vi "KVP Parser.vi"(4 "Values":variant[](array[variant]), 6 "Keys":string[](array[string]), 8 "Strict type matching? (F)":bool, 9 "Default Value Name (empty: label)":string, 10 "Default Value":variant, 11 "Parent Name":string) -> (0 "all found?":bool, 1 "any found?":bool, 2 "Value":variant, 3 "name out":string)   [LabVIEW 2013]
doc: "This VI takes a default value as the input and replaces it recursively (cluster, array) with values found in key value pair arrays."
uses:
  TypeDescriptor/TypeDescriptor_GetPString.vi
  TypeDescriptor/TypeDescriptor_SetName.vi
  <vilib>/Utility/GetType.llb/TD_Create Cluster.vi
  TypeDescriptor/OpenDescriptor.lvlib
  Variant/OpenVariant.lvlib
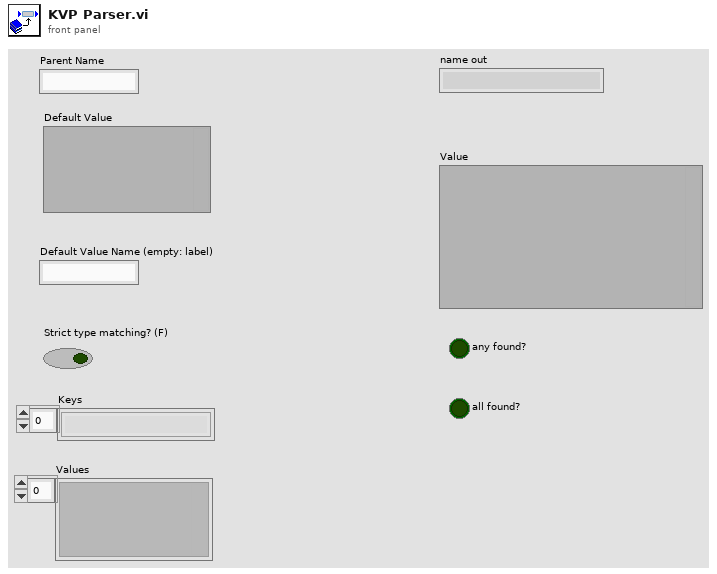
[diagram p1: front panel]
types:
  T1 = typedef "Type Enum.ctl" = enum8{"Void", "I8", "I16", "I32", "I64", "U8", "U16", "U32", "U64", "Single Float", "Double Float", "Extended Float", "Single Complex", "Double Complex", "Extended Complex", "Enum I8 NEVER", "Enum I16 NEVER", "Enum I32 NEVER", "Enum I64 NEVER", "Enum U8", "Enum U16", "Enum U32", "Enum U64", "Single Float With Unit", "Double Float With Unit", "Extended Float With Unit", "Single Complex With Unit", "Double Complex With Unit", "Extended Complex With Unit", "boolU16", "Boolean", "String", "Handle", "Path", "Picture", "C String", "Pascal String", "Tag", "SubString", "Array", "SubArray", "Cluster", "Numeric Cluster", "Variant", "LV Variant", "Measure Data (waveform)", "Refnum", "ExtData", "function", "Typedef", "Poly VI", "bad wire", "LabVIEW Class Instance"}
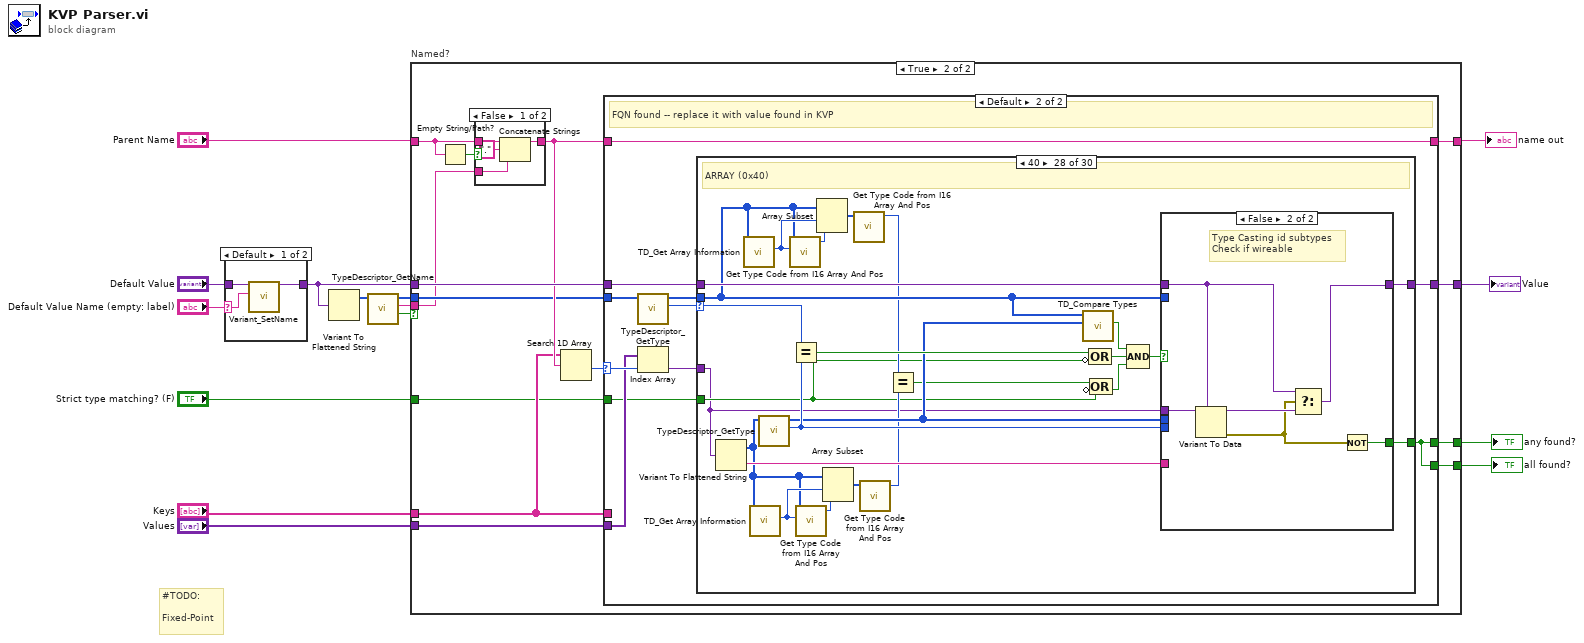
[diagram p0: block diagram]
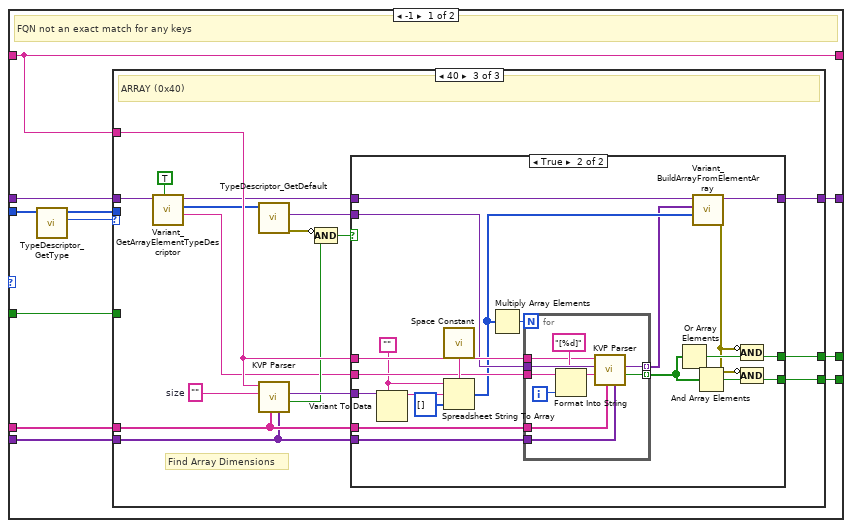
[diagram p5: hidden frame]
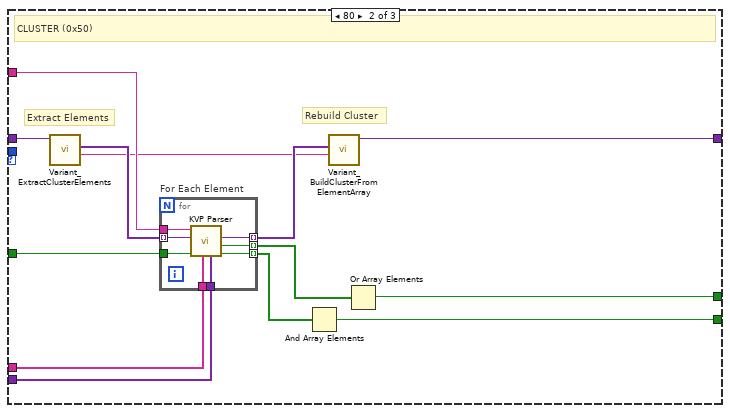
[diagram p7: hidden frame]
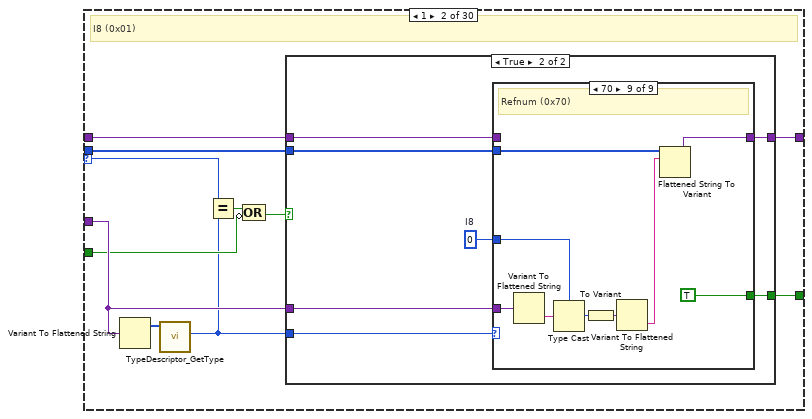
[diagram p10: hidden frame]
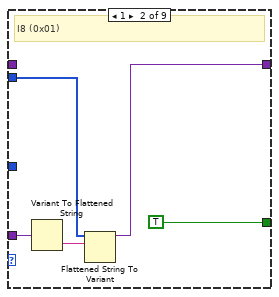
[diagram p13: hidden frame]
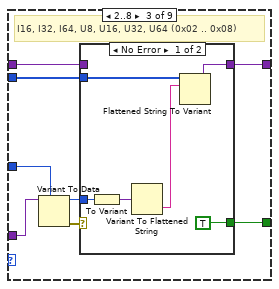
[diagram p14: hidden frame]
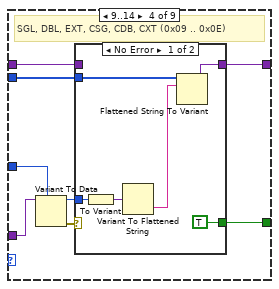
[diagram p16: hidden frame]
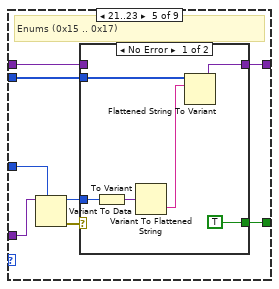
[diagram p18: hidden frame]
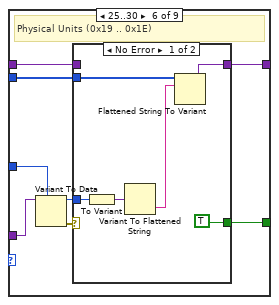
[diagram p20: hidden frame]
diagram:
  # "#TODO: \n\nFixed-Point"
  n1 = case shown="Default" "Default Value Name (empty: label)" {
    selector: "Default Value Name (empty: label)" -> [w17 _]
    tunnel: "Default Value" -> [w18 w19]
    tunnel: [w16 w19] -> w4
    frame Default {
      n2 = call "Variant_SetName.vi"("Name"=w17, "Variant"=w18) -> ("Named Variant"=w16:variant)  [unwired: 9 in]
    }
    frame "" {
    }
  }
  n3 = Variant To Flattened String(Variant=w4) -> (1:w3:i16[])  [unwired: 1 out]
  n4 = call "TypeDescriptor_GetName.vi"("type descriptor"=w3) -> ("found"=w1:bool, "name"=w2:string, "type descriptor dup"=w15:i16[])  [unwired: 8 in]
  n5 = case "Named?" shown="True" w1 {
    tunnel: [w21 w35] -> w13
    tunnel: w4 -> [w21 w34]
    tunnel: w15 -> [_ w26]
    tunnel: w2 -> [_ w22]
    tunnel: "Values" -> [_ w33]
    tunnel: "Keys" -> [_ w27]
    tunnel: "Parent Name" -> [w20 w29]
    tunnel: [w20 w32] -> w14
    tunnel: "Strict type matching? (F)" -> [_ w25]
    tunnel: [_ w24] -> w8
    tunnel: [_ w23] -> w7
    frame False {
      # "No Name Found -- no value to replace"
    }
    frame True {
      # "Has Name?"
      n6 = Empty String/Path?(string/path=w29) -> (empty?=w30:bool)
      n7 = case shown="False" w30 {
        tunnel: w22 -> [w37 w40]
        tunnel: [w38 w40] -> w28
        tunnel: w29 -> [w39 _]
        frame False {
          n8 = Concatenate Strings(w39, "." ("string"), w37) -> (w38:string)
        }
        frame True {
        }
      }
      n9 = Search 1D Array(1D array=w27, element=w28) -> (index of element=w31:i32)  [unwired: 1 in]
      n10 = case shown="Default" w31 {
        selector: w31 -> [_ w127]
        tunnel: [w50 w133] -> w35
        tunnel: w34 -> [w49 w132]
        tunnel: w26 -> [w51 w131]
        tunnel: w33 -> [w47 w126]
        tunnel: w28 -> [w45 w128]
        tunnel: [w45 w128] -> w32
        tunnel: w27 -> [w48 _]
        tunnel: w25 -> [w44 w124]
        tunnel: [w43 w123] -> w24
        tunnel: [w42 w123] -> w23
        frame -1 {
          # "FQN not an exact match for any keys"
          n11 = call "TypeDescriptor_GetType.vi"("type descriptor"=w51) -> ("Type"=w46:u8, "type descriptor dup"=w41:i16[])  [unwired: 9 in]
          n12 = case shown="40" w46 {
            tunnel: [w52 w54 w88] -> w50
            tunnel: w49 -> [w52 w63 w76]
            tunnel: w47 -> [_ w65 w86]
            tunnel: w48 -> [_ w64 w87]
            tunnel: w45 -> [_ w62 w83]
            tunnel: w44 -> [_ w61 _]
            tunnel: [_ w59 w90] -> w43
            tunnel: [_ w57 w89] -> w42
            tunnel: w41 -> [_ _ _]
            frame Default {
              # "No Match"
            }
            frame 80 {
              # "Rebuild Cluster"
              # "Extract Elements"
              # "CLUSTER (0x50)"
              n13 = call "Variant_ExtractClusterElements.vi"("Cluster"=w63) -> ("name"=w53:string, "Elements"=w55:variant[])  [unwired: 8 in, 1 out]
              n14 = for "For Each Element" {
                tunnel: [w73] -> w56 mode=indexing
                tunnel: w65 -> [w66]
                tunnel: w64 -> [w72]
                tunnel: w55 -> [w71] mode=indexing
                tunnel: w62 -> [w70]
                tunnel: [w69] -> w60 mode=indexing
                tunnel: [w68] -> w58 mode=indexing
                tunnel: w61 -> [w67]
                n15 = call "KVP Parser.vi"("Values"=w66, "Keys"=w72, "Strict type matching? (F)"=w67, "Default Value"=w71, "Parent Name"=w70) -> ("all found?"=w69:bool, "any found?"=w68:bool, "Value"=w73:variant)  [unwired: 3 in, 1 out]
              }
              n16 = And Array Elements(Boolean array=w60) -> (logical AND=w59:bool)
              n17 = call "Variant_BuildClusterFromElementArray.vi"("name"=w53, "Elements"=w56) -> ("Cluster"=w54:variant)  [unwired: 9 in]
              n18 = Or Array Elements(Boolean array=w58) -> (logical OR=w57:bool)
            }
            frame 64 {
              w84 = ""  # size
              # "Find Array Dimensions"
              # "ARRAY (0x40)"
              n19 = call "Variant_GetArrayElementTypeDescriptor.vi"("Name Element if empty string (F)"=TRUE, "Array"=w76) -> ("Element Name"=w78:string, "Element Descriptor"=w77:i16[], "Array dup"=w75:variant)  [unwired: 7 in]
              n20 = call "TypeDescriptor_GetDefault.vi"("type descriptor"=w77) -> ("error out"=w74:errorcluster, "Default"=w81:variant)  [unwired: 8 in, 1 out]
              n21 = call "KVP Parser.vi"("Values"=w86, "Keys"=w87, "Default Value"=w84, "Parent Name"=w83) -> ("any found?"=w80:bool, "Value"=w85:variant)  [unwired: 4 in, 2 out]
              n22 = Compound Arithmetic op=AND(invert w74, w80) -> (w79:bool)
              n23 = case shown="True" w79 {
                tunnel: [_ w95] -> w90
                tunnel: [_ w98] -> w89
                tunnel: [w91 w100] -> w88
                tunnel: w87 -> [_ w108]
                tunnel: w86 -> [_ w107]
                tunnel: w85 -> [_ w106]
                tunnel: w83 -> [_ w104]
                tunnel: w78 -> [_ w103]
                tunnel: w75 -> [w91 w101]
                tunnel: w81 -> [_ w94]
                frame False {
                  # "No Array Dimensions Found in the key value pairs"
                }
                frame True {
                  w102 = "" ("format string")
                  n24 = Variant To Data(type=w102, Variant=w106) -> (data=w105:string)  [unwired: 1 in, 1 out]
                  n25 = call <vilib>:"Space Constant.vi"() -> ("String"=w109:string)
                  n26 = Spreadsheet String To Array(delimiter (Tab)=w109, format string=w102, spreadsheet string=w105, array type (2D Dbl)=u32[] [] ("Dimensions")) -> (array=w93:u32[])
                  n27 = Multiply Array Elements(1:w93) -> (0:w112:u32)
                  n28 = for {
                    N: w112 -> [_]
                    tunnel: w94 -> [w122]
                    tunnel: w107 -> [w120]
                    tunnel: w108 -> [w118]
                    tunnel: w104 -> [w117]
                    tunnel: [w116] -> w111 mode=indexing
                    tunnel: w103 -> [w115]
                    tunnel: [w113] -> w92 mode=indexing
                    i -> [w114]
                    n29 = Format Into String(format string="[%d]", initial string=w115, w114) -> (resulting string=w119:string)  [unwired: 1 in, 1 out]
                    n30 = call "KVP Parser.vi"("Values"=w120, "Keys"=w118, "Default Value Name (empty: label)"=w119, "Default Value"=w122, "Parent Name"=w117) -> ("any found?"=w116:bool, "Value"=w113:variant)  [unwired: 3 in, 2 out]
                  }
                  n31 = Or Array Elements(Boolean array=w111) -> (logical OR=w99:bool)
                  n32 = call "Variant_BuildArrayFromElementArray.vi"("Dimensions"=w93, "Elements"=w92, "Default Array"=w101) -> ("error out"=w97:errorcluster, "Output Array"=w100:variant)  [unwired: 7 in]
                  n33 = And Array Elements(Boolean array=w111) -> (logical AND=w96:bool)
                  n34 = Compound Arithmetic op=AND(invert w97, w99) -> (w98:bool)
                  n35 = Compound Arithmetic op=AND(invert w97, w96) -> (w95:bool)
                }
              }
            }
          }
        }
        frame Default {
          # "FQN found -- replace it with value found in KVP"
          n36 = call "TypeDescriptor_GetType.vi"("type descriptor"=w131) -> ("Type"=w129:u8, "type descriptor dup"=w130:i16[])  [unwired: 9 in]
          n37 = Index Array(array=w126, index=w127) -> (element=w125:variant)
          n38 = case shown="40" w129 {
            selector: w129 -> [_ w136 w268 w398 w530 w661 w792 w923 w1054 w1184 w1272 w1361 w1449 w1519 w1588 w1658 w1763 w1867 w1969 w2041 w2110 w2181 w2251 w2320 w2390 w2448 w2749 w2810 _ w2850]
            tunnel: w125 -> [_ w141 w272 w403 w534 w665 w796 w927 w1058 w1189 w1277 w1365 w1453 w1524 w1593 w1663 w1768 w1872 w1975 w2045 w2115 w2185 w2255 w2325 w2395 w2454 w2758 w2791 w2839 w2864]
            tunnel: [w134 w143 w274 w405 w536 w667 w798 w929 w1060 w1191 w1279 w1367 w1455 w1526 w1595 w1665 w1770 w1874 w1977 w2047 w2117 w2187 w2257 w2327 w2397 w2457 w2754 w2813 w2831 w2860] -> w133
            tunnel: w132 -> [w134 w144 w275 w406 w537 w668 w799 w930 w1061 w1192 w1280 w1368 w1456 w1522 w1596 w1666 w1771 w1875 w1978 w2048 w2118 w2188 w2258 w2328 w2398 w2458 w2755 w2814 w2840 w2861]
            tunnel: w130 -> [_ w142 w273 w404 w535 w666 w797 w928 w1059 w1190 w1278 w1366 w1454 w1525 w1594 w1664 w1769 w1873 w1976 w2046 w2116 w2186 w2256 w2326 w2396 w2456 w2753 w2805 _ w2857]
            tunnel: [_ w140 w271 w402 w533 w664 w795 w926 w1057 w1188 w1276 w1364 w1452 w1523 w1592 w1662 w1767 w1871 w1974 w2044 w2114 w2184 w2254 w2324 w2394 w2451 w2751 w2812 w2832 w2855] -> w123
            tunnel: w124 -> [_ w137 w266 w399 w528 w659 w791 w921 w1053 w1185 w1273 w1359 w1447 w1518 w1589 w1659 w1764 w1868 w1971 w2039 w2111 w2180 w2249 w2321 w2391 w2446 w2747 w2793 w2836 w2852]
            frame Default {
            }
            frame 1 {
              # "I8 (0x01)"
              n39 = Variant To Flattened String(Variant=w141) -> (1:w145:i16[])  [unwired: 1 out]
              n40 = call "TypeDescriptor_GetType.vi"("type descriptor"=w145) -> ("Type"=w135:u8)  [unwired: 9 in, 1 out]
              n41 = Equal?(x=w136, y=w135) -> (x = y?=w139:bool)
              n42 = Compound Arithmetic op=OR(w139, invert w137) -> (w138:bool)
              n43 = case shown="True" w138 {
                tunnel: w144 -> [w146 w153]
                tunnel: [w146 w152] -> w143
                tunnel: w142 -> [_ w151]
                tunnel: w135 -> [_ w150]
                tunnel: w141 -> [_ w148]
                tunnel: [_ w147] -> w140
                frame False {
                }
                frame True {
                  w149 = i8 0  # I8
                  n44 = case shown="70" w150 {
                    tunnel: w153 -> [w154 _ w164 w179 w194 w209 w221 w243 _]
                    tunnel: [w154 w156 w166 w181 w196 w211 w227 w245 w264] -> w152
                    tunnel: w151 -> [_ w157 w167 w182 w197 w212 w228 w247 w265]
                    tunnel: w149 -> [_ _ w162 w177 w192 w207 w222 w241 w263]
                    tunnel: w148 -> [_ w159 w161 w176 w191 w206 w226 w240 w259]
                    tunnel: [_ TRUE w160 w175 w190 w205 w220 w239 TRUE] -> w147
                    frame Default {
                      # "INCOMPATIBLE DATATYPES"
                    }
                    frame 1 {
                      # "I8 (0x01)"
                      n45 = Variant To Flattened String(Variant=w159) -> (data string=w158:string)  [unwired: 1 out]
                      n46 = Flattened String To Variant(6:w158, 7:w157) -> (3:w156:variant)  [unwired: 1 in, 1 out]
                    }
                    frame 2..8 {
                      # "I16, I32, I64, U8, U16, U32, U64 (0x02 .. 0x08)"
                      n47 = Variant To Data(type=w162, Variant=w161) -> (data=w163:i8, error out=w165:errorcluster)  [unwired: 1 in]
                      n48 = case shown="No Error" w165 {
                        tunnel: w167 -> [w173 _]
                        tunnel: [w172 w174] -> w166
                        tunnel: w164 -> [_ w174]
                        tunnel: w163 -> [w170 _]
                        tunnel: [TRUE _] -> w160
                        frame No Error {
                          n49 = To Variant(anything=w170) -> (Variant=w169:variant)
                          n50 = Variant To Flattened String(Variant=w169) -> (data string=w171:string)  [unwired: 1 out]
                          n51 = Flattened String To Variant(6:w171, 7:w173) -> (3:w172:variant)  [unwired: 1 in, 1 out]
                        }
                        frame Error {
                        }
                      }
                    }
                    frame 9..14 {
                      # "SGL, DBL, EXT, CSG, CDB, CXT (0x09 .. 0x0E)"
                      n52 = Variant To Data(type=w177, Variant=w176) -> (data=w178:i8, error out=w180:errorcluster)  [unwired: 1 in]
                      n53 = case shown="No Error" w180 {
                        tunnel: w182 -> [w188 _]
                        tunnel: [w187 w189] -> w181
                        tunnel: w179 -> [_ w189]
                        tunnel: w178 -> [w185 _]
                        tunnel: [TRUE _] -> w175
                        frame No Error {
                          n54 = To Variant(anything=w185) -> (Variant=w184:variant)
                          n55 = Variant To Flattened String(Variant=w184) -> (data string=w186:string)  [unwired: 1 out]
                          n56 = Flattened String To Variant(6:w186, 7:w188) -> (3:w187:variant)  [unwired: 1 in, 1 out]
                        }
                        frame Error {
                        }
                      }
                    }
                    frame 21..23 {
                      # "Enums (0x15 .. 0x17)"
                      n57 = Variant To Data(type=w192, Variant=w191) -> (data=w193:i8, error out=w195:errorcluster)  [unwired: 1 in]
                      n58 = case shown="No Error" w195 {
                        tunnel: w197 -> [w203 _]
                        tunnel: [w202 w204] -> w196
                        tunnel: w194 -> [_ w204]
                        tunnel: w193 -> [w200 _]
                        tunnel: [TRUE _] -> w190
                        frame No Error {
                          n59 = To Variant(anything=w200) -> (Variant=w199:variant)
                          n60 = Variant To Flattened String(Variant=w199) -> (data string=w201:string)  [unwired: 1 out]
                          n61 = Flattened String To Variant(6:w201, 7:w203) -> (3:w202:variant)  [unwired: 1 in, 1 out]
                        }
                        frame Error {
                        }
                      }
                    }
                    frame 25..30 {
                      # "Physical Units (0x19 .. 0x1E)"
                      n62 = Variant To Data(type=w207, Variant=w206) -> (data=w208:i8, error out=w210:errorcluster)  [unwired: 1 in]
                      n63 = case shown="No Error" w210 {
                        tunnel: w212 -> [w218 _]
                        tunnel: [w217 w219] -> w211
                        tunnel: w209 -> [_ w219]
                        tunnel: w208 -> [w215 _]
                        tunnel: [TRUE _] -> w205
                        frame No Error {
                          n64 = To Variant(anything=w215) -> (Variant=w214:variant)
                          n65 = Variant To Flattened String(Variant=w214) -> (data string=w216:string)  [unwired: 1 out]
                          n66 = Flattened String To Variant(6:w216, 7:w218) -> (3:w217:variant)  [unwired: 1 in, 1 out]
                        }
                        frame Error {
                        }
                      }
                    }
                    frame 33 {
                      # "Boolean (0x21)"
                      n67 = Variant To Data(type=FALSE, Variant=w226) -> (data=w223:bool, error out=w224:errorcluster)  [unwired: 1 in]
                      n68 = case shown="No Error" w224 {
                        tunnel: w228 -> [w237 _]
                        tunnel: [w236 w238] -> w227
                        tunnel: w223 -> [w233 _]
                        tunnel: w222 -> [w231 _]
                        tunnel: w221 -> [_ w238]
                        tunnel: [TRUE _] -> w220
                        frame No Error {
                          n69 = Boolean To (0,1)(Boolean=w233) -> (0, 1=w232:i16)
                          n70 = Variant To Data(type=w231, Variant=w232) -> (data=w230:i8)  [unwired: 1 in, 1 out]
                          n71 = To Variant(anything=w230) -> (Variant=w234:variant)
                          n72 = Variant To Flattened String(Variant=w234) -> (data string=w235:string)  [unwired: 1 out]
                          n73 = Flattened String To Variant(6:w235, 7:w237) -> (3:w236:variant)  [unwired: 1 in, 1 out]
                        }
                        frame Error {
                        }
                      }
                    }
                    frame 48 {
                      # "STRING (0x30)"
                      n74 = Variant To Data(type="", Variant=w240) -> (data=w242:string, error out=w244:errorcluster)  [unwired: 1 in]
                      n75 = case shown="No Error" w244 {
                        tunnel: w247 -> [w255 _]
                        tunnel: [w254 w256] -> w245
                        tunnel: w243 -> [_ w256]
                        tunnel: w242 -> [w251 _]
                        tunnel: w241 -> [w249 _]
                        tunnel: [TRUE _] -> w239
                        frame No Error {
                          n76 = Fract/Exp String To Number(string=w251, default (0 dbl)=w249) -> (number=w250:i8)  [unwired: 2 in, 1 out]
                          n77 = To Variant(anything=w250) -> (Variant=w253:variant)
                          n78 = Variant To Flattened String(Variant=w253) -> (data string=w252:string)  [unwired: 1 out]
                          n79 = Flattened String To Variant(6:w252, 7:w255) -> (3:w254:variant)  [unwired: 1 in, 1 out]
                        }
                        frame Error {
                        }
                      }
                    }
                    frame 112 {
                      # "Refnum (0x70)"
                      n80 = Variant To Flattened String(Variant=w259) -> (data string=w258:string)  [unwired: 1 out]
                      n81 = Type Cast(type=w263, x=w258) -> (*(type *) &x=w262:i8)
                      n82 = To Variant(anything=w262) -> (Variant=w261:variant)
                      n83 = Variant To Flattened String(Variant=w261) -> (data string=w260:string)  [unwired: 1 out]
                      n84 = Flattened String To Variant(6:w260, 7:w265) -> (3:w264:variant)  [unwired: 1 in, 1 out]
                    }
                  }
                }
              }
            }
            frame 2 {
              # "I16 (0x02)"
              n85 = Variant To Flattened String(Variant=w272) -> (1:w276:i16[])  [unwired: 1 out]
              n86 = call "TypeDescriptor_GetType.vi"("type descriptor"=w276) -> ("Type"=w267:u8)  [unwired: 9 in, 1 out]
              n87 = Equal?(x=w268, y=w267) -> (x = y?=w270:bool)
              n88 = Compound Arithmetic op=OR(w270, invert w266) -> (w269:bool)
              n89 = case shown="True" w269 {
                tunnel: w275 -> [w277 w284]
                tunnel: [w277 w283] -> w274
                tunnel: w273 -> [_ w282]
                tunnel: w267 -> [_ w281]
                tunnel: w272 -> [_ w279]
                tunnel: [_ w278] -> w271
                frame False {
                }
                frame True {
                  w280 = i16 0  # I16
                  n90 = case shown="1, 3..8" w281 {
                    tunnel: w284 -> [w285 _ w295 w310 w325 w340 w352 w374 _]
                    tunnel: [w285 w287 w297 w312 w327 w342 w358 w376 w395] -> w283
                    tunnel: w282 -> [_ w288 w298 w313 w328 w343 w359 w378 w396]
                    tunnel: w280 -> [_ _ w293 w308 w323 w338 w353 w372 w394]
                    tunnel: w279 -> [_ w290 w292 w307 w322 w337 w357 w371 w390]
                    tunnel: [_ TRUE w291 w306 w321 w336 w351 w370 TRUE] -> w278
                    frame Default {
                      # "INCOMPATIBLE DATATYPES"
                    }
                    frame 2 {
                      # "I16 (0x02)"
                      n91 = Variant To Flattened String(Variant=w290) -> (data string=w289:string)  [unwired: 1 out]
                      n92 = Flattened String To Variant(6:w289, 7:w288) -> (3:w287:variant)  [unwired: 1 in, 1 out]
                    }
                    frame 1, 3..8 {
                      # "I8, I32, I64, U8, U16, U32, U64 (0x02 .. 0x08)"
                      n93 = Variant To Data(type=w293, Variant=w292) -> (data=w294:i16, error out=w296:errorcluster)  [unwired: 1 in]
                      n94 = case shown="No Error" w296 {
                        tunnel: w298 -> [w304 _]
                        tunnel: [w303 w305] -> w297
                        tunnel: w295 -> [_ w305]
                        tunnel: w294 -> [w301 _]
                        tunnel: [TRUE _] -> w291
                        frame No Error {
                          n95 = To Variant(anything=w301) -> (Variant=w300:variant)
                          n96 = Variant To Flattened String(Variant=w300) -> (data string=w302:string)  [unwired: 1 out]
                          n97 = Flattened String To Variant(6:w302, 7:w304) -> (3:w303:variant)  [unwired: 1 in, 1 out]
                        }
                        frame Error {
                        }
                      }
                    }
                    frame 9..14 {
                      # "SGL, DBL, EXT, CSG, CDB, CXT (0x09 .. 0x0E)"
                      n98 = Variant To Data(type=w308, Variant=w307) -> (data=w309:i16, error out=w311:errorcluster)  [unwired: 1 in]
                      n99 = case shown="No Error" w311 {
                        tunnel: w313 -> [w319 _]
                        tunnel: [w318 w320] -> w312
                        tunnel: w310 -> [_ w320]
                        tunnel: w309 -> [w316 _]
                        tunnel: [TRUE _] -> w306
                        frame No Error {
                          n100 = To Variant(anything=w316) -> (Variant=w315:variant)
                          n101 = Variant To Flattened String(Variant=w315) -> (data string=w317:string)  [unwired: 1 out]
                          n102 = Flattened String To Variant(6:w317, 7:w319) -> (3:w318:variant)  [unwired: 1 in, 1 out]
                        }
                        frame Error {
                        }
                      }
                    }
                    frame 21..23 {
                      # "Enums (0x15 .. 0x17)"
                      n103 = Variant To Data(type=w323, Variant=w322) -> (data=w324:i16, error out=w326:errorcluster)  [unwired: 1 in]
                      n104 = case shown="No Error" w326 {
                        tunnel: w328 -> [w334 _]
                        tunnel: [w333 w335] -> w327
                        tunnel: w325 -> [_ w335]
                        tunnel: w324 -> [w331 _]
                        tunnel: [TRUE _] -> w321
                        frame No Error {
                          n105 = To Variant(anything=w331) -> (Variant=w330:variant)
                          n106 = Variant To Flattened String(Variant=w330) -> (data string=w332:string)  [unwired: 1 out]
                          n107 = Flattened String To Variant(6:w332, 7:w334) -> (3:w333:variant)  [unwired: 1 in, 1 out]
                        }
                        frame Error {
                        }
                      }
                    }
                    frame 25..30 {
                      # "Physical Units (0x19 .. 0x1E)"
                      n108 = Variant To Data(type=w338, Variant=w337) -> (data=w339:i16, error out=w341:errorcluster)  [unwired: 1 in]
                      n109 = case shown="No Error" w341 {
                        tunnel: w343 -> [w349 _]
                        tunnel: [w348 w350] -> w342
                        tunnel: w340 -> [_ w350]
                        tunnel: w339 -> [w346 _]
                        tunnel: [TRUE _] -> w336
                        frame No Error {
                          n110 = To Variant(anything=w346) -> (Variant=w345:variant)
                          n111 = Variant To Flattened String(Variant=w345) -> (data string=w347:string)  [unwired: 1 out]
                          n112 = Flattened String To Variant(6:w347, 7:w349) -> (3:w348:variant)  [unwired: 1 in, 1 out]
                        }
                        frame Error {
                        }
                      }
                    }
                    frame 33 {
                      # "Boolean (0x21)"
                      n113 = Variant To Data(type=FALSE, Variant=w357) -> (data=w354:bool, error out=w355:errorcluster)  [unwired: 1 in]
                      n114 = case shown="No Error" w355 {
                        tunnel: w359 -> [w368 _]
                        tunnel: [w367 w369] -> w358
                        tunnel: w354 -> [w364 _]
                        tunnel: w353 -> [w362 _]
                        tunnel: w352 -> [_ w369]
                        tunnel: [TRUE _] -> w351
                        frame No Error {
                          n115 = Boolean To (0,1)(Boolean=w364) -> (0, 1=w363:i16)
                          n116 = Variant To Data(type=w362, Variant=w363) -> (data=w361:i16)  [unwired: 1 in, 1 out]
                          n117 = To Variant(anything=w361) -> (Variant=w365:variant)
                          n118 = Variant To Flattened String(Variant=w365) -> (data string=w366:string)  [unwired: 1 out]
                          n119 = Flattened String To Variant(6:w366, 7:w368) -> (3:w367:variant)  [unwired: 1 in, 1 out]
                        }
                        frame Error {
                        }
                      }
                    }
                    frame 48 {
                      # "STRING (0x30)"
                      n120 = Variant To Data(type="", Variant=w371) -> (data=w373:string, error out=w375:errorcluster)  [unwired: 1 in]
                      n121 = case shown="No Error" w375 {
                        tunnel: w378 -> [w386 _]
                        tunnel: [w385 w387] -> w376
                        tunnel: w374 -> [_ w387]
                        tunnel: w373 -> [w382 _]
                        tunnel: w372 -> [w380 _]
                        tunnel: [TRUE _] -> w370
                        frame No Error {
                          n122 = Fract/Exp String To Number(string=w382, default (0 dbl)=w380) -> (number=w381:i16)  [unwired: 2 in, 1 out]
                          n123 = To Variant(anything=w381) -> (Variant=w384:variant)
                          n124 = Variant To Flattened String(Variant=w384) -> (data string=w383:string)  [unwired: 1 out]
                          n125 = Flattened String To Variant(6:w383, 7:w386) -> (3:w385:variant)  [unwired: 1 in, 1 out]
                        }
                        frame Error {
                        }
                      }
                    }
                    frame 112 {
                      # "Refnum (0x70)"
                      n126 = Variant To Flattened String(Variant=w390) -> (data string=w389:string)  [unwired: 1 out]
                      n127 = Type Cast(type=w394, x=w389) -> (*(type *) &x=w393:i16)
                      n128 = To Variant(anything=w393) -> (Variant=w392:variant)
                      n129 = Variant To Flattened String(Variant=w392) -> (data string=w391:string)  [unwired: 1 out]
                      n130 = Flattened String To Variant(6:w391, 7:w396) -> (3:w395:variant)  [unwired: 1 in, 1 out]
                    }
                  }
                }
              }
            }
            frame 3 {
              # "I32 (0x03)"
              n131 = Variant To Flattened String(Variant=w403) -> (1:w407:i16[])  [unwired: 1 out]
              n132 = call "TypeDescriptor_GetType.vi"("type descriptor"=w407) -> ("Type"=w397:u8)  [unwired: 9 in, 1 out]
              n133 = Equal?(x=w398, y=w397) -> (x = y?=w401:bool)
              n134 = Compound Arithmetic op=OR(w401, invert w399) -> (w400:bool)
              n135 = case shown="True" w400 {
                tunnel: w406 -> [w408 w415]
                tunnel: [w408 w414] -> w405
                tunnel: w404 -> [_ w413]
                tunnel: w397 -> [_ w412]
                tunnel: w403 -> [_ w410]
                tunnel: [_ w409] -> w402
                frame False {
                }
                frame True {
                  w411 = 0  # I32
                  n136 = case shown="21" w412 {
                    tunnel: w415 -> [w416 _ w426 w441 w456 w471 w483 w505 _]
                    tunnel: [w416 w418 w428 w443 w458 w473 w489 w507 w526] -> w414
                    tunnel: w413 -> [_ w419 w429 w444 w459 w474 w490 w509 w527]
                    tunnel: w411 -> [_ _ w424 w439 w454 w469 w484 w503 w525]
                    tunnel: w410 -> [_ w421 w423 w438 w453 w468 w488 w502 w521]
                    tunnel: [_ TRUE w422 w437 w452 w467 w482 w501 TRUE] -> w409
                    frame Default {
                      # "INCOMPATIBLE DATATYPES"
                    }
                    frame 3 {
                      # "I32 (0x03)"
                      n137 = Variant To Flattened String(Variant=w421) -> (data string=w420:string)  [unwired: 1 out]
                      n138 = Flattened String To Variant(6:w420, 7:w419) -> (3:w418:variant)  [unwired: 1 in, 1 out]
                    }
                    frame 1, 2, 4..8 {
                      # "I8, I16, I64, U8, U16, U32, U64 (0x02 .. 0x08)"
                      n139 = Variant To Data(type=w424, Variant=w423) -> (data=w425:i32, error out=w427:errorcluster)  [unwired: 1 in]
                      n140 = case shown="No Error" w427 {
                        tunnel: w429 -> [w435 _]
                        tunnel: [w434 w436] -> w428
                        tunnel: w426 -> [_ w436]
                        tunnel: w425 -> [w432 _]
                        tunnel: [TRUE _] -> w422
                        frame No Error {
                          n141 = To Variant(anything=w432) -> (Variant=w431:variant)
                          n142 = Variant To Flattened String(Variant=w431) -> (data string=w433:string)  [unwired: 1 out]
                          n143 = Flattened String To Variant(6:w433, 7:w435) -> (3:w434:variant)  [unwired: 1 in, 1 out]
                        }
                        frame Error {
                        }
                      }
                    }
                    frame 9..14 {
                      # "SGL, DBL, EXT, CSG, CDB, CXT (0x09 .. 0x0E)"
                      n144 = Variant To Data(type=w439, Variant=w438) -> (data=w440:i32, error out=w442:errorcluster)  [unwired: 1 in]
                      n145 = case shown="No Error" w442 {
                        tunnel: w444 -> [w450 _]
                        tunnel: [w449 w451] -> w443
                        tunnel: w441 -> [_ w451]
                        tunnel: w440 -> [w447 _]
                        tunnel: [TRUE _] -> w437
                        frame No Error {
                          n146 = To Variant(anything=w447) -> (Variant=w446:variant)
                          n147 = Variant To Flattened String(Variant=w446) -> (data string=w448:string)  [unwired: 1 out]
                          n148 = Flattened String To Variant(6:w448, 7:w450) -> (3:w449:variant)  [unwired: 1 in, 1 out]
                        }
                        frame Error {
                        }
                      }
                    }
                    frame 21..23 {
                      # "Enums (0x15 .. 0x17)"
                      n149 = Variant To Data(type=w454, Variant=w453) -> (data=w455:i32, error out=w457:errorcluster)  [unwired: 1 in]
                      n150 = case shown="No Error" w457 {
                        tunnel: w459 -> [w465 _]
                        tunnel: [w464 w466] -> w458
                        tunnel: w456 -> [_ w466]
                        tunnel: w455 -> [w462 _]
                        tunnel: [TRUE _] -> w452
                        frame No Error {
                          n151 = To Variant(anything=w462) -> (Variant=w461:variant)
                          n152 = Variant To Flattened String(Variant=w461) -> (data string=w463:string)  [unwired: 1 out]
                          n153 = Flattened String To Variant(6:w463, 7:w465) -> (3:w464:variant)  [unwired: 1 in, 1 out]
                        }
                        frame Error {
                        }
                      }
                    }
                    frame 25..30 {
                      # "Physical Units (0x19 .. 0x1E)"
                      n154 = Variant To Data(type=w469, Variant=w468) -> (data=w470:i32, error out=w472:errorcluster)  [unwired: 1 in]
                      n155 = case shown="No Error" w472 {
                        tunnel: w474 -> [w480 _]
                        tunnel: [w479 w481] -> w473
                        tunnel: w471 -> [_ w481]
                        tunnel: w470 -> [w477 _]
                        tunnel: [TRUE _] -> w467
                        frame No Error {
                          n156 = To Variant(anything=w477) -> (Variant=w476:variant)
                          n157 = Variant To Flattened String(Variant=w476) -> (data string=w478:string)  [unwired: 1 out]
                          n158 = Flattened String To Variant(6:w478, 7:w480) -> (3:w479:variant)  [unwired: 1 in, 1 out]
                        }
                        frame Error {
                        }
                      }
                    }
                    frame 33 {
                      # "Boolean (0x21)"
                      n159 = Variant To Data(type=FALSE, Variant=w488) -> (data=w485:bool, error out=w486:errorcluster)  [unwired: 1 in]
                      n160 = case shown="No Error" w486 {
                        tunnel: w490 -> [w499 _]
                        tunnel: [w498 w500] -> w489
                        tunnel: w485 -> [w495 _]
                        tunnel: w484 -> [w493 _]
                        tunnel: w483 -> [_ w500]
                        tunnel: [TRUE _] -> w482
                        frame No Error {
                          n161 = Boolean To (0,1)(Boolean=w495) -> (0, 1=w494:i16)
                          n162 = Variant To Data(type=w493, Variant=w494) -> (data=w492:i32)  [unwired: 1 in, 1 out]
                          n163 = To Variant(anything=w492) -> (Variant=w496:variant)
                          n164 = Variant To Flattened String(Variant=w496) -> (data string=w497:string)  [unwired: 1 out]
                          n165 = Flattened String To Variant(6:w497, 7:w499) -> (3:w498:variant)  [unwired: 1 in, 1 out]
                        }
                        frame Error {
                        }
                      }
                    }
                    frame 48 {
                      # "STRING (0x30)"
                      n166 = Variant To Data(type="", Variant=w502) -> (data=w504:string, error out=w506:errorcluster)  [unwired: 1 in]
                      n167 = case shown="No Error" w506 {
                        tunnel: w509 -> [w517 _]
                        tunnel: [w516 w518] -> w507
                        tunnel: w505 -> [_ w518]
                        tunnel: w504 -> [w513 _]
                        tunnel: w503 -> [w511 _]
                        tunnel: [TRUE _] -> w501
                        frame No Error {
                          n168 = Fract/Exp String To Number(string=w513, default (0 dbl)=w511) -> (number=w512:i32)  [unwired: 2 in, 1 out]
                          n169 = To Variant(anything=w512) -> (Variant=w515:variant)
                          n170 = Variant To Flattened String(Variant=w515) -> (data string=w514:string)  [unwired: 1 out]
                          n171 = Flattened String To Variant(6:w514, 7:w517) -> (3:w516:variant)  [unwired: 1 in, 1 out]
                        }
                        frame Error {
                        }
                      }
                    }
                    frame 112 {
                      # "Refnum (0x70)"
                      n172 = Variant To Flattened String(Variant=w521) -> (data string=w520:string)  [unwired: 1 out]
                      n173 = Type Cast(type=w525, x=w520) -> (*(type *) &x=w524:i32)
                      n174 = To Variant(anything=w524) -> (Variant=w523:variant)
                      n175 = Variant To Flattened String(Variant=w523) -> (data string=w522:string)  [unwired: 1 out]
                      n176 = Flattened String To Variant(6:w522, 7:w527) -> (3:w526:variant)  [unwired: 1 in, 1 out]
                    }
                  }
                }
              }
            }
            frame 4 {
              # "I64 (0x04)"
              n177 = Variant To Flattened String(Variant=w534) -> (1:w538:i16[])  [unwired: 1 out]
              n178 = call "TypeDescriptor_GetType.vi"("type descriptor"=w538) -> ("Type"=w529:u8)  [unwired: 9 in, 1 out]
              n179 = Equal?(x=w530, y=w529) -> (x = y?=w532:bool)
              n180 = Compound Arithmetic op=OR(w532, invert w528) -> (w531:bool)
              n181 = case shown="True" w531 {
                tunnel: w537 -> [w539 w546]
                tunnel: [w539 w545] -> w536
                tunnel: w535 -> [_ w544]
                tunnel: w529 -> [_ w543]
                tunnel: w534 -> [_ w541]
                tunnel: [_ w540] -> w533
                frame False {
                }
                frame True {
                  w542 = i64 0  # I64
                  n182 = case shown="1..3, 5..8" w543 {
                    tunnel: w546 -> [w547 _ w557 w572 w587 w602 w614 w636 _]
                    tunnel: [w547 w549 w559 w574 w589 w604 w620 w638 w657] -> w545
                    tunnel: w544 -> [_ w550 w560 w575 w590 w605 w621 w640 w658]
                    tunnel: w542 -> [_ _ w555 w570 w585 w600 w615 w634 w656]
                    tunnel: w541 -> [_ w552 w554 w569 w584 w599 w619 w633 w652]
                    tunnel: [_ TRUE w553 w568 w583 w598 w613 w632 TRUE] -> w540
                    frame Default {
                      # "INCOMPATIBLE DATATYPES"
                    }
                    frame 4 {
                      # "I64 (0x04)"
                      n183 = Variant To Flattened String(Variant=w552) -> (data string=w551:string)  [unwired: 1 out]
                      n184 = Flattened String To Variant(6:w551, 7:w550) -> (3:w549:variant)  [unwired: 1 in, 1 out]
                    }
                    frame 1..3, 5..8 {
                      # "I8, I16, I32, U8, U16, U32, U64"
                      n185 = Variant To Data(type=w555, Variant=w554) -> (data=w556:i64, error out=w558:errorcluster)  [unwired: 1 in]
                      n186 = case shown="No Error" w558 {
                        tunnel: w560 -> [w566 _]
                        tunnel: [w565 w567] -> w559
                        tunnel: w557 -> [_ w567]
                        tunnel: w556 -> [w563 _]
                        tunnel: [TRUE _] -> w553
                        frame No Error {
                          n187 = To Variant(anything=w563) -> (Variant=w562:variant)
                          n188 = Variant To Flattened String(Variant=w562) -> (data string=w564:string)  [unwired: 1 out]
                          n189 = Flattened String To Variant(6:w564, 7:w566) -> (3:w565:variant)  [unwired: 1 in, 1 out]
                        }
                        frame Error {
                        }
                      }
                    }
                    frame 9..14 {
                      # "SGL, DBL, EXT, CSG, CDB, CXT (0x09 .. 0x0E)"
                      n190 = Variant To Data(type=w570, Variant=w569) -> (data=w571:i64, error out=w573:errorcluster)  [unwired: 1 in]
                      n191 = case shown="No Error" w573 {
                        tunnel: w575 -> [w581 _]
                        tunnel: [w580 w582] -> w574
                        tunnel: w572 -> [_ w582]
                        tunnel: w571 -> [w578 _]
                        tunnel: [TRUE _] -> w568
                        frame No Error {
                          n192 = To Variant(anything=w578) -> (Variant=w577:variant)
                          n193 = Variant To Flattened String(Variant=w577) -> (data string=w579:string)  [unwired: 1 out]
                          n194 = Flattened String To Variant(6:w579, 7:w581) -> (3:w580:variant)  [unwired: 1 in, 1 out]
                        }
                        frame Error {
                        }
                      }
                    }
                    frame 21..23 {
                      # "Enums (0x15 .. 0x17)"
                      n195 = Variant To Data(type=w585, Variant=w584) -> (data=w586:i64, error out=w588:errorcluster)  [unwired: 1 in]
                      n196 = case shown="No Error" w588 {
                        tunnel: w590 -> [w596 _]
                        tunnel: [w595 w597] -> w589
                        tunnel: w587 -> [_ w597]
                        tunnel: w586 -> [w593 _]
                        tunnel: [TRUE _] -> w583
                        frame No Error {
                          n197 = To Variant(anything=w593) -> (Variant=w592:variant)
                          n198 = Variant To Flattened String(Variant=w592) -> (data string=w594:string)  [unwired: 1 out]
                          n199 = Flattened String To Variant(6:w594, 7:w596) -> (3:w595:variant)  [unwired: 1 in, 1 out]
                        }
                        frame Error {
                        }
                      }
                    }
                    frame 25..30 {
                      # "Physical Units (0x19 .. 0x1E)"
                      n200 = Variant To Data(type=w600, Variant=w599) -> (data=w601:i64, error out=w603:errorcluster)  [unwired: 1 in]
                      n201 = case shown="No Error" w603 {
                        tunnel: w605 -> [w611 _]
                        tunnel: [w610 w612] -> w604
                        tunnel: w602 -> [_ w612]
                        tunnel: w601 -> [w608 _]
                        tunnel: [TRUE _] -> w598
                        frame No Error {
                          n202 = To Variant(anything=w608) -> (Variant=w607:variant)
                          n203 = Variant To Flattened String(Variant=w607) -> (data string=w609:string)  [unwired: 1 out]
                          n204 = Flattened String To Variant(6:w609, 7:w611) -> (3:w610:variant)  [unwired: 1 in, 1 out]
                        }
                        frame Error {
                        }
                      }
                    }
                    frame 33 {
                      # "Boolean (0x21)"
                      n205 = Variant To Data(type=FALSE, Variant=w619) -> (data=w616:bool, error out=w617:errorcluster)  [unwired: 1 in]
                      n206 = case shown="No Error" w617 {
                        tunnel: w621 -> [w630 _]
                        tunnel: [w629 w631] -> w620
                        tunnel: w616 -> [w626 _]
                        tunnel: w615 -> [w624 _]
                        tunnel: w614 -> [_ w631]
                        tunnel: [TRUE _] -> w613
                        frame No Error {
                          n207 = Boolean To (0,1)(Boolean=w626) -> (0, 1=w625:i16)
                          n208 = Variant To Data(type=w624, Variant=w625) -> (data=w623:i64)  [unwired: 1 in, 1 out]
                          n209 = To Variant(anything=w623) -> (Variant=w627:variant)
                          n210 = Variant To Flattened String(Variant=w627) -> (data string=w628:string)  [unwired: 1 out]
                          n211 = Flattened String To Variant(6:w628, 7:w630) -> (3:w629:variant)  [unwired: 1 in, 1 out]
                        }
                        frame Error {
                        }
                      }
                    }
                    frame 48 {
                      # "STRING (0x30)"
                      n212 = Variant To Data(type="", Variant=w633) -> (data=w635:string, error out=w637:errorcluster)  [unwired: 1 in]
                      n213 = case shown="No Error" w637 {
                        tunnel: w640 -> [w648 _]
                        tunnel: [w647 w649] -> w638
                        tunnel: w636 -> [_ w649]
                        tunnel: w635 -> [w644 _]
                        tunnel: w634 -> [w642 _]
                        tunnel: [TRUE _] -> w632
                        frame No Error {
                          n214 = Fract/Exp String To Number(string=w644, default (0 dbl)=w642) -> (number=w643:i64)  [unwired: 2 in, 1 out]
                          n215 = To Variant(anything=w643) -> (Variant=w646:variant)
                          n216 = Variant To Flattened String(Variant=w646) -> (data string=w645:string)  [unwired: 1 out]
                          n217 = Flattened String To Variant(6:w645, 7:w648) -> (3:w647:variant)  [unwired: 1 in, 1 out]
                        }
                        frame Error {
                        }
                      }
                    }
                    frame 112 {
                      # "Refnum (0x70)"
                      n218 = Variant To Flattened String(Variant=w652) -> (data string=w651:string)  [unwired: 1 out]
                      n219 = Type Cast(type=w656, x=w651) -> (*(type *) &x=w655:i64)
                      n220 = To Variant(anything=w655) -> (Variant=w654:variant)
                      n221 = Variant To Flattened String(Variant=w654) -> (data string=w653:string)  [unwired: 1 out]
                      n222 = Flattened String To Variant(6:w653, 7:w658) -> (3:w657:variant)  [unwired: 1 in, 1 out]
                    }
                  }
                }
              }
            }
            frame 5 {
              # "U8 (0x05)"
              n223 = Variant To Flattened String(Variant=w665) -> (1:w669:i16[])  [unwired: 1 out]
              n224 = call "TypeDescriptor_GetType.vi"("type descriptor"=w669) -> ("Type"=w660:u8)  [unwired: 9 in, 1 out]
              n225 = Equal?(x=w661, y=w660) -> (x = y?=w663:bool)
              n226 = Compound Arithmetic op=OR(w663, invert w659) -> (w662:bool)
              n227 = case shown="True" w662 {
                tunnel: w668 -> [w670 w677]
                tunnel: [w670 w676] -> w667
                tunnel: w666 -> [_ w675]
                tunnel: w660 -> [_ w674]
                tunnel: w665 -> [_ w672]
                tunnel: [_ w671] -> w664
                frame False {
                }
                frame True {
                  w673 = u8 0  # U8
                  n228 = case shown="1..4, 6..8" w674 {
                    tunnel: w677 -> [w678 _ w688 w703 w718 w733 w745 w767 _]
                    tunnel: [w678 w680 w690 w705 w720 w735 w751 w769 w788] -> w676
                    tunnel: w675 -> [_ w681 w691 w706 w721 w736 w752 w771 w789]
                    tunnel: w673 -> [_ _ w686 w701 w716 w731 w746 w765 w787]
                    tunnel: w672 -> [_ w683 w685 w700 w715 w730 w750 w764 w783]
                    tunnel: [_ TRUE w684 w699 w714 w729 w744 w763 TRUE] -> w671
                    frame Default {
                      # "INCOMPATIBLE DATATYPES"
                    }
                    frame 5 {
                      # "U8 (0x05)"
                      n229 = Variant To Flattened String(Variant=w683) -> (data string=w682:string)  [unwired: 1 out]
                      n230 = Flattened String To Variant(6:w682, 7:w681) -> (3:w680:variant)  [unwired: 1 in, 1 out]
                    }
                    frame 1..4, 6..8 {
                      # "I8, I16, I32, I64, U16, U32, U64"
                      n231 = Variant To Data(type=w686, Variant=w685) -> (data=w687:u8, error out=w689:errorcluster)  [unwired: 1 in]
                      n232 = case shown="No Error" w689 {
                        tunnel: w691 -> [w697 _]
                        tunnel: [w696 w698] -> w690
                        tunnel: w688 -> [_ w698]
                        tunnel: w687 -> [w694 _]
                        tunnel: [TRUE _] -> w684
                        frame No Error {
                          n233 = To Variant(anything=w694) -> (Variant=w693:variant)
                          n234 = Variant To Flattened String(Variant=w693) -> (data string=w695:string)  [unwired: 1 out]
                          n235 = Flattened String To Variant(6:w695, 7:w697) -> (3:w696:variant)  [unwired: 1 in, 1 out]
                        }
                        frame Error {
                        }
                      }
                    }
                    frame 9..14 {
                      # "SGL, DBL, EXT, CSG, CDB, CXT (0x09 .. 0x0E)"
                      n236 = Variant To Data(type=w701, Variant=w700) -> (data=w702:u8, error out=w704:errorcluster)  [unwired: 1 in]
                      n237 = case shown="No Error" w704 {
                        tunnel: w706 -> [w712 _]
                        tunnel: [w711 w713] -> w705
                        tunnel: w703 -> [_ w713]
                        tunnel: w702 -> [w709 _]
                        tunnel: [TRUE _] -> w699
                        frame No Error {
                          n238 = To Variant(anything=w709) -> (Variant=w708:variant)
                          n239 = Variant To Flattened String(Variant=w708) -> (data string=w710:string)  [unwired: 1 out]
                          n240 = Flattened String To Variant(6:w710, 7:w712) -> (3:w711:variant)  [unwired: 1 in, 1 out]
                        }
                        frame Error {
                        }
                      }
                    }
                    frame 21..23 {
                      # "Enums (0x15 .. 0x17)"
                      n241 = Variant To Data(type=w716, Variant=w715) -> (data=w717:u8, error out=w719:errorcluster)  [unwired: 1 in]
                      n242 = case shown="No Error" w719 {
                        tunnel: w721 -> [w727 _]
                        tunnel: [w726 w728] -> w720
                        tunnel: w718 -> [_ w728]
                        tunnel: w717 -> [w724 _]
                        tunnel: [TRUE _] -> w714
                        frame No Error {
                          n243 = To Variant(anything=w724) -> (Variant=w723:variant)
                          n244 = Variant To Flattened String(Variant=w723) -> (data string=w725:string)  [unwired: 1 out]
                          n245 = Flattened String To Variant(6:w725, 7:w727) -> (3:w726:variant)  [unwired: 1 in, 1 out]
                        }
                        frame Error {
                        }
                      }
                    }
                    frame 25..30 {
                      # "Physical Units (0x19 .. 0x1E)"
                      n246 = Variant To Data(type=w731, Variant=w730) -> (data=w732:u8, error out=w734:errorcluster)  [unwired: 1 in]
                      n247 = case shown="No Error" w734 {
                        tunnel: w736 -> [w742 _]
                        tunnel: [w741 w743] -> w735
                        tunnel: w733 -> [_ w743]
                        tunnel: w732 -> [w739 _]
                        tunnel: [TRUE _] -> w729
                        frame No Error {
                          n248 = To Variant(anything=w739) -> (Variant=w738:variant)
                          n249 = Variant To Flattened String(Variant=w738) -> (data string=w740:string)  [unwired: 1 out]
                          n250 = Flattened String To Variant(6:w740, 7:w742) -> (3:w741:variant)  [unwired: 1 in, 1 out]
                        }
                        frame Error {
                        }
                      }
                    }
                    frame 33 {
                      # "Boolean (0x21)"
                      n251 = Variant To Data(type=FALSE, Variant=w750) -> (data=w747:bool, error out=w748:errorcluster)  [unwired: 1 in]
                      n252 = case shown="No Error" w748 {
                        tunnel: w752 -> [w761 _]
                        tunnel: [w760 w762] -> w751
                        tunnel: w747 -> [w757 _]
                        tunnel: w746 -> [w755 _]
                        tunnel: w745 -> [_ w762]
                        tunnel: [TRUE _] -> w744
                        frame No Error {
                          n253 = Boolean To (0,1)(Boolean=w757) -> (0, 1=w756:i16)
                          n254 = Variant To Data(type=w755, Variant=w756) -> (data=w754:u8)  [unwired: 1 in, 1 out]
                          n255 = To Variant(anything=w754) -> (Variant=w758:variant)
                          n256 = Variant To Flattened String(Variant=w758) -> (data string=w759:string)  [unwired: 1 out]
                          n257 = Flattened String To Variant(6:w759, 7:w761) -> (3:w760:variant)  [unwired: 1 in, 1 out]
                        }
                        frame Error {
                        }
                      }
                    }
                    frame 48 {
                      # "STRING (0x30)"
                      n258 = Variant To Data(type="", Variant=w764) -> (data=w766:string, error out=w768:errorcluster)  [unwired: 1 in]
                      n259 = case shown="No Error" w768 {
                        tunnel: w771 -> [w779 _]
                        tunnel: [w778 w780] -> w769
                        tunnel: w767 -> [_ w780]
                        tunnel: w766 -> [w775 _]
                        tunnel: w765 -> [w773 _]
                        tunnel: [TRUE _] -> w763
                        frame No Error {
                          n260 = Fract/Exp String To Number(string=w775, default (0 dbl)=w773) -> (number=w774:u8)  [unwired: 2 in, 1 out]
                          n261 = To Variant(anything=w774) -> (Variant=w777:variant)
                          n262 = Variant To Flattened String(Variant=w777) -> (data string=w776:string)  [unwired: 1 out]
                          n263 = Flattened String To Variant(6:w776, 7:w779) -> (3:w778:variant)  [unwired: 1 in, 1 out]
                        }
                        frame Error {
                        }
                      }
                    }
                    frame 112 {
                      # "Refnum (0x70)"
                      n264 = Variant To Flattened String(Variant=w783) -> (data string=w782:string)  [unwired: 1 out]
                      n265 = Type Cast(type=w787, x=w782) -> (*(type *) &x=w786:u8)
                      n266 = To Variant(anything=w786) -> (Variant=w785:variant)
                      n267 = Variant To Flattened String(Variant=w785) -> (data string=w784:string)  [unwired: 1 out]
                      n268 = Flattened String To Variant(6:w784, 7:w789) -> (3:w788:variant)  [unwired: 1 in, 1 out]
                    }
                  }
                }
              }
            }
            frame 6 {
              # "U16 (0x06)"
              n269 = Variant To Flattened String(Variant=w796) -> (1:w800:i16[])  [unwired: 1 out]
              n270 = call "TypeDescriptor_GetType.vi"("type descriptor"=w800) -> ("Type"=w790:u8)  [unwired: 9 in, 1 out]
              n271 = Equal?(x=w792, y=w790) -> (x = y?=w794:bool)
              n272 = Compound Arithmetic op=OR(w794, invert w791) -> (w793:bool)
              n273 = case shown="True" w793 {
                tunnel: w799 -> [w801 w808]
                tunnel: [w801 w807] -> w798
                tunnel: w797 -> [_ w806]
                tunnel: w790 -> [_ w805]
                tunnel: w796 -> [_ w803]
                tunnel: [_ w802] -> w795
                frame False {
                }
                frame True {
                  w804 = u16 0  # U16
                  n274 = case shown="1..5, 7, 8" w805 {
                    tunnel: w808 -> [w809 _ w819 w834 w849 w864 w876 w898 _]
                    tunnel: [w809 w811 w821 w836 w851 w866 w882 w900 w919] -> w807
                    tunnel: w806 -> [_ w812 w822 w837 w852 w867 w883 w902 w920]
                    tunnel: w804 -> [_ _ w817 w832 w847 w862 w877 w896 w918]
                    tunnel: w803 -> [_ w814 w816 w831 w846 w861 w881 w895 w914]
                    tunnel: [_ TRUE w815 w830 w845 w860 w875 w894 TRUE] -> w802
                    frame Default {
                      # "INCOMPATIBLE DATATYPES"
                    }
                    frame 6 {
                      # "U16 (0x06)"
                      n275 = Variant To Flattened String(Variant=w814) -> (data string=w813:string)  [unwired: 1 out]
                      n276 = Flattened String To Variant(6:w813, 7:w812) -> (3:w811:variant)  [unwired: 1 in, 1 out]
                    }
                    frame 1..5, 7, 8 {
                      # "I8, I16, I32, I64, U8, U32, U64"
                      n277 = Variant To Data(type=w817, Variant=w816) -> (data=w818:u16, error out=w820:errorcluster)  [unwired: 1 in]
                      n278 = case shown="No Error" w820 {
                        tunnel: w822 -> [w828 _]
                        tunnel: [w827 w829] -> w821
                        tunnel: w819 -> [_ w829]
                        tunnel: w818 -> [w825 _]
                        tunnel: [TRUE _] -> w815
                        frame No Error {
                          n279 = To Variant(anything=w825) -> (Variant=w824:variant)
                          n280 = Variant To Flattened String(Variant=w824) -> (data string=w826:string)  [unwired: 1 out]
                          n281 = Flattened String To Variant(6:w826, 7:w828) -> (3:w827:variant)  [unwired: 1 in, 1 out]
                        }
                        frame Error {
                        }
                      }
                    }
                    frame 9..14 {
                      # "SGL, DBL, EXT, CSG, CDB, CXT (0x09 .. 0x0E)"
                      n282 = Variant To Data(type=w832, Variant=w831) -> (data=w833:u16, error out=w835:errorcluster)  [unwired: 1 in]
                      n283 = case shown="No Error" w835 {
                        tunnel: w837 -> [w843 _]
                        tunnel: [w842 w844] -> w836
                        tunnel: w834 -> [_ w844]
                        tunnel: w833 -> [w840 _]
                        tunnel: [TRUE _] -> w830
                        frame No Error {
                          n284 = To Variant(anything=w840) -> (Variant=w839:variant)
                          n285 = Variant To Flattened String(Variant=w839) -> (data string=w841:string)  [unwired: 1 out]
                          n286 = Flattened String To Variant(6:w841, 7:w843) -> (3:w842:variant)  [unwired: 1 in, 1 out]
                        }
                        frame Error {
                        }
                      }
                    }
                    frame 21..23 {
                      # "Enums (0x15 .. 0x17)"
                      n287 = Variant To Data(type=w847, Variant=w846) -> (data=w848:u16, error out=w850:errorcluster)  [unwired: 1 in]
                      n288 = case shown="No Error" w850 {
                        tunnel: w852 -> [w858 _]
                        tunnel: [w857 w859] -> w851
                        tunnel: w849 -> [_ w859]
                        tunnel: w848 -> [w855 _]
                        tunnel: [TRUE _] -> w845
                        frame No Error {
                          n289 = To Variant(anything=w855) -> (Variant=w854:variant)
                          n290 = Variant To Flattened String(Variant=w854) -> (data string=w856:string)  [unwired: 1 out]
                          n291 = Flattened String To Variant(6:w856, 7:w858) -> (3:w857:variant)  [unwired: 1 in, 1 out]
                        }
                        frame Error {
                        }
                      }
                    }
                    frame 25..30 {
                      # "Physical Units (0x19 .. 0x1E)"
                      n292 = Variant To Data(type=w862, Variant=w861) -> (data=w863:u16, error out=w865:errorcluster)  [unwired: 1 in]
                      n293 = case shown="No Error" w865 {
                        tunnel: w867 -> [w873 _]
                        tunnel: [w872 w874] -> w866
                        tunnel: w864 -> [_ w874]
                        tunnel: w863 -> [w870 _]
                        tunnel: [TRUE _] -> w860
                        frame No Error {
                          n294 = To Variant(anything=w870) -> (Variant=w869:variant)
                          n295 = Variant To Flattened String(Variant=w869) -> (data string=w871:string)  [unwired: 1 out]
                          n296 = Flattened String To Variant(6:w871, 7:w873) -> (3:w872:variant)  [unwired: 1 in, 1 out]
                        }
                        frame Error {
                        }
                      }
                    }
                    frame 33 {
                      # "Boolean (0x21)"
                      n297 = Variant To Data(type=FALSE, Variant=w881) -> (data=w878:bool, error out=w879:errorcluster)  [unwired: 1 in]
                      n298 = case shown="No Error" w879 {
                        tunnel: w883 -> [w892 _]
                        tunnel: [w891 w893] -> w882
                        tunnel: w878 -> [w888 _]
                        tunnel: w877 -> [w886 _]
                        tunnel: w876 -> [_ w893]
                        tunnel: [TRUE _] -> w875
                        frame No Error {
                          n299 = Boolean To (0,1)(Boolean=w888) -> (0, 1=w887:i16)
                          n300 = Variant To Data(type=w886, Variant=w887) -> (data=w885:u16)  [unwired: 1 in, 1 out]
                          n301 = To Variant(anything=w885) -> (Variant=w889:variant)
                          n302 = Variant To Flattened String(Variant=w889) -> (data string=w890:string)  [unwired: 1 out]
                          n303 = Flattened String To Variant(6:w890, 7:w892) -> (3:w891:variant)  [unwired: 1 in, 1 out]
                        }
                        frame Error {
                        }
                      }
                    }
                    frame 48 {
                      # "STRING (0x30)"
                      n304 = Variant To Data(type="", Variant=w895) -> (data=w897:string, error out=w899:errorcluster)  [unwired: 1 in]
                      n305 = case shown="No Error" w899 {
                        tunnel: w902 -> [w910 _]
                        tunnel: [w909 w911] -> w900
                        tunnel: w898 -> [_ w911]
                        tunnel: w897 -> [w906 _]
                        tunnel: w896 -> [w904 _]
                        tunnel: [TRUE _] -> w894
                        frame No Error {
                          n306 = Fract/Exp String To Number(string=w906, default (0 dbl)=w904) -> (number=w905:u16)  [unwired: 2 in, 1 out]
                          n307 = To Variant(anything=w905) -> (Variant=w908:variant)
                          n308 = Variant To Flattened String(Variant=w908) -> (data string=w907:string)  [unwired: 1 out]
                          n309 = Flattened String To Variant(6:w907, 7:w910) -> (3:w909:variant)  [unwired: 1 in, 1 out]
                        }
                        frame Error {
                        }
                      }
                    }
                    frame 112 {
                      # "Refnum (0x70)"
                      n310 = Variant To Flattened String(Variant=w914) -> (data string=w913:string)  [unwired: 1 out]
                      n311 = Type Cast(type=w918, x=w913) -> (*(type *) &x=w917:u16)
                      n312 = To Variant(anything=w917) -> (Variant=w916:variant)
                      n313 = Variant To Flattened String(Variant=w916) -> (data string=w915:string)  [unwired: 1 out]
                      n314 = Flattened String To Variant(6:w915, 7:w920) -> (3:w919:variant)  [unwired: 1 in, 1 out]
                    }
                  }
                }
              }
            }
            frame 7 {
              # "U32 (0x07)"
              n315 = Variant To Flattened String(Variant=w927) -> (1:w931:i16[])  [unwired: 1 out]
              n316 = call "TypeDescriptor_GetType.vi"("type descriptor"=w931) -> ("Type"=w922:u8)  [unwired: 9 in, 1 out]
              n317 = Equal?(x=w923, y=w922) -> (x = y?=w925:bool)
              n318 = Compound Arithmetic op=OR(w925, invert w921) -> (w924:bool)
              n319 = case shown="True" w924 {
                tunnel: w930 -> [w932 w939]
                tunnel: [w932 w938] -> w929
                tunnel: w928 -> [_ w937]
                tunnel: w922 -> [_ w936]
                tunnel: w927 -> [_ w934]
                tunnel: [_ w933] -> w926
                frame False {
                }
                frame True {
                  w935 = u32 0  # U32
                  n320 = case shown="1..6, 8" w936 {
                    tunnel: w939 -> [w940 _ w950 w965 w980 w995 w1007 w1029 _]
                    tunnel: [w940 w942 w952 w967 w982 w997 w1013 w1031 w1050] -> w938
                    tunnel: w937 -> [_ w943 w953 w968 w983 w998 w1014 w1033 w1051]
                    tunnel: w935 -> [_ _ w948 w963 w978 w993 w1008 w1027 w1049]
                    tunnel: w934 -> [_ w945 w947 w962 w977 w992 w1012 w1026 w1045]
                    tunnel: [_ TRUE w946 w961 w976 w991 w1006 w1025 TRUE] -> w933
                    frame Default {
                      # "INCOMPATIBLE DATATYPES"
                    }
                    frame 7 {
                      # "U32 (0x07)"
                      n321 = Variant To Flattened String(Variant=w945) -> (data string=w944:string)  [unwired: 1 out]
                      n322 = Flattened String To Variant(6:w944, 7:w943) -> (3:w942:variant)  [unwired: 1 in, 1 out]
                    }
                    frame 1..6, 8 {
                      # "I8, I16, I32, I64, U8, U16, U64"
                      n323 = Variant To Data(type=w948, Variant=w947) -> (data=w949:u32, error out=w951:errorcluster)  [unwired: 1 in]
                      n324 = case shown="No Error" w951 {
                        tunnel: w953 -> [w959 _]
                        tunnel: [w958 w960] -> w952
                        tunnel: w950 -> [_ w960]
                        tunnel: w949 -> [w956 _]
                        tunnel: [TRUE _] -> w946
                        frame No Error {
                          n325 = To Variant(anything=w956) -> (Variant=w955:variant)
                          n326 = Variant To Flattened String(Variant=w955) -> (data string=w957:string)  [unwired: 1 out]
                          n327 = Flattened String To Variant(6:w957, 7:w959) -> (3:w958:variant)  [unwired: 1 in, 1 out]
                        }
                        frame Error {
                        }
                      }
                    }
                    frame 9..14 {
                      # "SGL, DBL, EXT, CSG, CDB, CXT (0x09 .. 0x0E)"
                      n328 = Variant To Data(type=w963, Variant=w962) -> (data=w964:u32, error out=w966:errorcluster)  [unwired: 1 in]
                      n329 = case shown="No Error" w966 {
                        tunnel: w968 -> [w974 _]
                        tunnel: [w973 w975] -> w967
                        tunnel: w965 -> [_ w975]
                        tunnel: w964 -> [w971 _]
                        tunnel: [TRUE _] -> w961
                        frame No Error {
                          n330 = To Variant(anything=w971) -> (Variant=w970:variant)
                          n331 = Variant To Flattened String(Variant=w970) -> (data string=w972:string)  [unwired: 1 out]
                          n332 = Flattened String To Variant(6:w972, 7:w974) -> (3:w973:variant)  [unwired: 1 in, 1 out]
                        }
                        frame Error {
                        }
                      }
                    }
                    frame 21..23 {
                      # "Enums (0x15 .. 0x17)"
                      n333 = Variant To Data(type=w978, Variant=w977) -> (data=w979:u32, error out=w981:errorcluster)  [unwired: 1 in]
                      n334 = case shown="No Error" w981 {
                        tunnel: w983 -> [w989 _]
                        tunnel: [w988 w990] -> w982
                        tunnel: w980 -> [_ w990]
                        tunnel: w979 -> [w986 _]
                        tunnel: [TRUE _] -> w976
                        frame No Error {
                          n335 = To Variant(anything=w986) -> (Variant=w985:variant)
                          n336 = Variant To Flattened String(Variant=w985) -> (data string=w987:string)  [unwired: 1 out]
                          n337 = Flattened String To Variant(6:w987, 7:w989) -> (3:w988:variant)  [unwired: 1 in, 1 out]
                        }
                        frame Error {
                        }
                      }
                    }
                    frame 25..30 {
                      # "Physical Units (0x19 .. 0x1E)"
                      n338 = Variant To Data(type=w993, Variant=w992) -> (data=w994:u32, error out=w996:errorcluster)  [unwired: 1 in]
                      n339 = case shown="No Error" w996 {
                        tunnel: w998 -> [w1004 _]
                        tunnel: [w1003 w1005] -> w997
                        tunnel: w995 -> [_ w1005]
                        tunnel: w994 -> [w1001 _]
                        tunnel: [TRUE _] -> w991
                        frame No Error {
                          n340 = To Variant(anything=w1001) -> (Variant=w1000:variant)
                          n341 = Variant To Flattened String(Variant=w1000) -> (data string=w1002:string)  [unwired: 1 out]
                          n342 = Flattened String To Variant(6:w1002, 7:w1004) -> (3:w1003:variant)  [unwired: 1 in, 1 out]
                        }
                        frame Error {
                        }
                      }
                    }
                    frame 33 {
                      # "Boolean (0x21)"
                      n343 = Variant To Data(type=FALSE, Variant=w1012) -> (data=w1009:bool, error out=w1010:errorcluster)  [unwired: 1 in]
                      n344 = case shown="No Error" w1010 {
                        tunnel: w1014 -> [w1023 _]
                        tunnel: [w1022 w1024] -> w1013
                        tunnel: w1009 -> [w1019 _]
                        tunnel: w1008 -> [w1017 _]
                        tunnel: w1007 -> [_ w1024]
                        tunnel: [TRUE _] -> w1006
                        frame No Error {
                          n345 = Boolean To (0,1)(Boolean=w1019) -> (0, 1=w1018:i16)
                          n346 = Variant To Data(type=w1017, Variant=w1018) -> (data=w1016:u32)  [unwired: 1 in, 1 out]
                          n347 = To Variant(anything=w1016) -> (Variant=w1020:variant)
                          n348 = Variant To Flattened String(Variant=w1020) -> (data string=w1021:string)  [unwired: 1 out]
                          n349 = Flattened String To Variant(6:w1021, 7:w1023) -> (3:w1022:variant)  [unwired: 1 in, 1 out]
                        }
                        frame Error {
                        }
                      }
                    }
                    frame 48 {
                      # "STRING (0x30)"
                      n350 = Variant To Data(type="", Variant=w1026) -> (data=w1028:string, error out=w1030:errorcluster)  [unwired: 1 in]
                      n351 = case shown="No Error" w1030 {
                        tunnel: w1033 -> [w1041 _]
                        tunnel: [w1040 w1042] -> w1031
                        tunnel: w1029 -> [_ w1042]
                        tunnel: w1028 -> [w1037 _]
                        tunnel: w1027 -> [w1035 _]
                        tunnel: [TRUE _] -> w1025
                        frame No Error {
                          n352 = Fract/Exp String To Number(string=w1037, default (0 dbl)=w1035) -> (number=w1036:u32)  [unwired: 2 in, 1 out]
                          n353 = To Variant(anything=w1036) -> (Variant=w1039:variant)
                          n354 = Variant To Flattened String(Variant=w1039) -> (data string=w1038:string)  [unwired: 1 out]
                          n355 = Flattened String To Variant(6:w1038, 7:w1041) -> (3:w1040:variant)  [unwired: 1 in, 1 out]
                        }
                        frame Error {
                        }
                      }
                    }
                    frame 112 {
                      # "Refnum (0x70)"
                      n356 = Variant To Flattened String(Variant=w1045) -> (data string=w1044:string)  [unwired: 1 out]
                      n357 = Type Cast(type=w1049, x=w1044) -> (*(type *) &x=w1048:u32)
                      n358 = To Variant(anything=w1048) -> (Variant=w1047:variant)
                      n359 = Variant To Flattened String(Variant=w1047) -> (data string=w1046:string)  [unwired: 1 out]
                      n360 = Flattened String To Variant(6:w1046, 7:w1051) -> (3:w1050:variant)  [unwired: 1 in, 1 out]
                    }
                  }
                }
              }
            }
            frame 8 {
              # "U64 (0x08)"
              n361 = Variant To Flattened String(Variant=w1058) -> (1:w1062:i16[])  [unwired: 1 out]
              n362 = call "TypeDescriptor_GetType.vi"("type descriptor"=w1062) -> ("Type"=w1052:u8)  [unwired: 9 in, 1 out]
              n363 = Equal?(x=w1054, y=w1052) -> (x = y?=w1056:bool)
              n364 = Compound Arithmetic op=OR(w1056, invert w1053) -> (w1055:bool)
              n365 = case shown="True" w1055 {
                tunnel: w1061 -> [w1063 w1070]
                tunnel: [w1063 w1069] -> w1060
                tunnel: w1059 -> [_ w1068]
                tunnel: w1052 -> [_ w1067]
                tunnel: w1058 -> [_ w1065]
                tunnel: [_ w1064] -> w1057
                frame False {
                }
                frame True {
                  w1066 = u64 0  # U64
                  n366 = case shown="1..7" w1067 {
                    tunnel: w1070 -> [w1071 _ w1081 w1096 w1111 w1126 w1138 w1160 _]
                    tunnel: [w1071 w1073 w1083 w1098 w1113 w1128 w1144 w1162 w1181] -> w1069
                    tunnel: w1068 -> [_ w1074 w1084 w1099 w1114 w1129 w1145 w1164 w1182]
                    tunnel: w1066 -> [_ _ w1079 w1094 w1109 w1124 w1139 w1158 w1180]
                    tunnel: w1065 -> [_ w1076 w1078 w1093 w1108 w1123 w1143 w1157 w1176]
                    tunnel: [_ TRUE w1077 w1092 w1107 w1122 w1137 w1156 TRUE] -> w1064
                    frame Default {
                      # "INCOMPATIBLE DATATYPES"
                    }
                    frame 8 {
                      # "U64 (0x08)"
                      n367 = Variant To Flattened String(Variant=w1076) -> (data string=w1075:string)  [unwired: 1 out]
                      n368 = Flattened String To Variant(6:w1075, 7:w1074) -> (3:w1073:variant)  [unwired: 1 in, 1 out]
                    }
                    frame 1..7 {
                      # "I8, I16, I32, I64, U8, U16, U32"
                      n369 = Variant To Data(type=w1079, Variant=w1078) -> (data=w1080:u64, error out=w1082:errorcluster)  [unwired: 1 in]
                      n370 = case shown="No Error" w1082 {
                        tunnel: w1084 -> [w1090 _]
                        tunnel: [w1089 w1091] -> w1083
                        tunnel: w1081 -> [_ w1091]
                        tunnel: w1080 -> [w1087 _]
                        tunnel: [TRUE _] -> w1077
                        frame No Error {
                          n371 = To Variant(anything=w1087) -> (Variant=w1086:variant)
                          n372 = Variant To Flattened String(Variant=w1086) -> (data string=w1088:string)  [unwired: 1 out]
                          n373 = Flattened String To Variant(6:w1088, 7:w1090) -> (3:w1089:variant)  [unwired: 1 in, 1 out]
                        }
                        frame Error {
                        }
                      }
                    }
                    frame 9..14 {
                      # "SGL, DBL, EXT, CSG, CDB, CXT (0x09 .. 0x0E)"
                      n374 = Variant To Data(type=w1094, Variant=w1093) -> (data=w1095:u64, error out=w1097:errorcluster)  [unwired: 1 in]
                      n375 = case shown="No Error" w1097 {
                        tunnel: w1099 -> [w1105 _]
                        tunnel: [w1104 w1106] -> w1098
                        tunnel: w1096 -> [_ w1106]
                        tunnel: w1095 -> [w1102 _]
                        tunnel: [TRUE _] -> w1092
                        frame No Error {
                          n376 = To Variant(anything=w1102) -> (Variant=w1101:variant)
                          n377 = Variant To Flattened String(Variant=w1101) -> (data string=w1103:string)  [unwired: 1 out]
                          n378 = Flattened String To Variant(6:w1103, 7:w1105) -> (3:w1104:variant)  [unwired: 1 in, 1 out]
                        }
                        frame Error {
                        }
                      }
                    }
                    frame 21..23 {
                      # "Enums (0x15 .. 0x17)"
                      n379 = Variant To Data(type=w1109, Variant=w1108) -> (data=w1110:u64, error out=w1112:errorcluster)  [unwired: 1 in]
                      n380 = case shown="No Error" w1112 {
                        tunnel: w1114 -> [w1120 _]
                        tunnel: [w1119 w1121] -> w1113
                        tunnel: w1111 -> [_ w1121]
                        tunnel: w1110 -> [w1117 _]
                        tunnel: [TRUE _] -> w1107
                        frame No Error {
                          n381 = To Variant(anything=w1117) -> (Variant=w1116:variant)
                          n382 = Variant To Flattened String(Variant=w1116) -> (data string=w1118:string)  [unwired: 1 out]
                          n383 = Flattened String To Variant(6:w1118, 7:w1120) -> (3:w1119:variant)  [unwired: 1 in, 1 out]
                        }
                        frame Error {
                        }
                      }
                    }
                    frame 25..30 {
                      # "Physical Units (0x19 .. 0x1E)"
                      n384 = Variant To Data(type=w1124, Variant=w1123) -> (data=w1125:u64, error out=w1127:errorcluster)  [unwired: 1 in]
                      n385 = case shown="No Error" w1127 {
                        tunnel: w1129 -> [w1135 _]
                        tunnel: [w1134 w1136] -> w1128
                        tunnel: w1126 -> [_ w1136]
                        tunnel: w1125 -> [w1132 _]
                        tunnel: [TRUE _] -> w1122
                        frame No Error {
                          n386 = To Variant(anything=w1132) -> (Variant=w1131:variant)
                          n387 = Variant To Flattened String(Variant=w1131) -> (data string=w1133:string)  [unwired: 1 out]
                          n388 = Flattened String To Variant(6:w1133, 7:w1135) -> (3:w1134:variant)  [unwired: 1 in, 1 out]
                        }
                        frame Error {
                        }
                      }
                    }
                    frame 33 {
                      # "Boolean (0x21)"
                      n389 = Variant To Data(type=FALSE, Variant=w1143) -> (data=w1140:bool, error out=w1141:errorcluster)  [unwired: 1 in]
                      n390 = case shown="No Error" w1141 {
                        tunnel: w1145 -> [w1154 _]
                        tunnel: [w1153 w1155] -> w1144
                        tunnel: w1140 -> [w1150 _]
                        tunnel: w1139 -> [w1148 _]
                        tunnel: w1138 -> [_ w1155]
                        tunnel: [TRUE _] -> w1137
                        frame No Error {
                          n391 = Boolean To (0,1)(Boolean=w1150) -> (0, 1=w1149:i16)
                          n392 = Variant To Data(type=w1148, Variant=w1149) -> (data=w1147:u64)  [unwired: 1 in, 1 out]
                          n393 = To Variant(anything=w1147) -> (Variant=w1151:variant)
                          n394 = Variant To Flattened String(Variant=w1151) -> (data string=w1152:string)  [unwired: 1 out]
                          n395 = Flattened String To Variant(6:w1152, 7:w1154) -> (3:w1153:variant)  [unwired: 1 in, 1 out]
                        }
                        frame Error {
                        }
                      }
                    }
                    frame 48 {
                      # "STRING (0x30)"
                      n396 = Variant To Data(type="", Variant=w1157) -> (data=w1159:string, error out=w1161:errorcluster)  [unwired: 1 in]
                      n397 = case shown="No Error" w1161 {
                        tunnel: w1164 -> [w1172 _]
                        tunnel: [w1171 w1173] -> w1162
                        tunnel: w1160 -> [_ w1173]
                        tunnel: w1159 -> [w1168 _]
                        tunnel: w1158 -> [w1166 _]
                        tunnel: [TRUE _] -> w1156
                        frame No Error {
                          n398 = Fract/Exp String To Number(string=w1168, default (0 dbl)=w1166) -> (number=w1167:u64)  [unwired: 2 in, 1 out]
                          n399 = To Variant(anything=w1167) -> (Variant=w1170:variant)
                          n400 = Variant To Flattened String(Variant=w1170) -> (data string=w1169:string)  [unwired: 1 out]
                          n401 = Flattened String To Variant(6:w1169, 7:w1172) -> (3:w1171:variant)  [unwired: 1 in, 1 out]
                        }
                        frame Error {
                        }
                      }
                    }
                    frame 112 {
                      # "Refnum (0x70)"
                      n402 = Variant To Flattened String(Variant=w1176) -> (data string=w1175:string)  [unwired: 1 out]
                      n403 = Type Cast(type=w1180, x=w1175) -> (*(type *) &x=w1179:u64)
                      n404 = To Variant(anything=w1179) -> (Variant=w1178:variant)
                      n405 = Variant To Flattened String(Variant=w1178) -> (data string=w1177:string)  [unwired: 1 out]
                      n406 = Flattened String To Variant(6:w1177, 7:w1182) -> (3:w1181:variant)  [unwired: 1 in, 1 out]
                    }
                  }
                }
              }
            }
            frame 9 {
              # "SGL (0x09)"
              n407 = Variant To Flattened String(Variant=w1189) -> (1:w1193:i16[])  [unwired: 1 out]
              n408 = call "TypeDescriptor_GetType.vi"("type descriptor"=w1193) -> ("Type"=w1183:u8)  [unwired: 9 in, 1 out]
              n409 = Equal?(x=w1184, y=w1183) -> (x = y?=w1187:bool)
              n410 = Compound Arithmetic op=OR(w1187, invert w1185) -> (w1186:bool)
              n411 = case shown="True" w1186 {
                tunnel: w1192 -> [w1194 w1201]
                tunnel: [w1194 w1200] -> w1191
                tunnel: w1190 -> [_ w1199]
                tunnel: w1183 -> [_ w1198]
                tunnel: w1189 -> [_ w1196]
                tunnel: [_ w1195] -> w1188
                frame False {
                }
                frame True {
                  w1197 = sgl 0.0  # SGL
                  n412 = case shown="30" w1198 {
                    tunnel: w1201 -> [w1202 _ w1212 w1227 w1242 w1257]
                    tunnel: [w1202 w1203 w1214 w1229 w1244 w1259] -> w1200
                    tunnel: w1199 -> [_ w1205 w1215 w1230 w1245 w1261]
                    tunnel: w1197 -> [_ _ w1210 w1225 w1240 w1255]
                    tunnel: w1196 -> [_ w1207 w1209 w1224 w1239 w1254]
                    tunnel: [_ TRUE w1208 w1223 w1238 w1253] -> w1195
                    frame Default {
                      # "INCOMPATIBLE DATATYPES"
                    }
                    frame 9 {
                      # "SGL (0x09)"
                      n413 = Variant To Flattened String(Variant=w1207) -> (data string=w1206:string)  [unwired: 1 out]
                      n414 = Flattened String To Variant(6:w1206, 7:w1205) -> (3:w1203:variant)  [unwired: 1 in, 1 out]
                    }
                    frame 1..8 {
                      # "I8, I16, I32, I64, U8, U16, U32, U64"
                      n415 = Variant To Data(type=w1210, Variant=w1209) -> (data=w1211:sgl, error out=w1213:errorcluster)  [unwired: 1 in]
                      n416 = case shown="No Error" w1213 {
                        tunnel: w1215 -> [w1221 _]
                        tunnel: [w1220 w1222] -> w1214
                        tunnel: w1212 -> [_ w1222]
                        tunnel: w1211 -> [w1218 _]
                        tunnel: [TRUE _] -> w1208
                        frame No Error {
                          n417 = To Variant(anything=w1218) -> (Variant=w1217:variant)
                          n418 = Variant To Flattened String(Variant=w1217) -> (data string=w1219:string)  [unwired: 1 out]
                          n419 = Flattened String To Variant(6:w1219, 7:w1221) -> (3:w1220:variant)  [unwired: 1 in, 1 out]
                        }
                        frame Error {
                        }
                      }
                    }
                    frame 10..14 {
                      # "DBL, EXT, CSG, CDB, CXT (0x10 .. 0x0E)"
                      n420 = Variant To Data(type=w1225, Variant=w1224) -> (data=w1226:sgl, error out=w1228:errorcluster)  [unwired: 1 in]
                      n421 = case shown="No Error" w1228 {
                        tunnel: w1230 -> [w1236 _]
                        tunnel: [w1235 w1237] -> w1229
                        tunnel: w1227 -> [_ w1237]
                        tunnel: w1226 -> [w1233 _]
                        tunnel: [TRUE _] -> w1223
                        frame No Error {
                          n422 = To Variant(anything=w1233) -> (Variant=w1232:variant)
                          n423 = Variant To Flattened String(Variant=w1232) -> (data string=w1234:string)  [unwired: 1 out]
                          n424 = Flattened String To Variant(6:w1234, 7:w1236) -> (3:w1235:variant)  [unwired: 1 in, 1 out]
                        }
                        frame Error {
                        }
                      }
                    }
                    frame 25..30 {
                      # "Physical Units (0x19 .. 0x1E)"
                      n425 = Variant To Data(type=w1240, Variant=w1239) -> (data=w1241:sgl, error out=w1243:errorcluster)  [unwired: 1 in]
                      n426 = case shown="No Error" w1243 {
                        tunnel: w1245 -> [w1251 _]
                        tunnel: [w1250 w1252] -> w1244
                        tunnel: w1242 -> [_ w1252]
                        tunnel: w1241 -> [w1248 _]
                        tunnel: [TRUE _] -> w1238
                        frame No Error {
                          n427 = To Variant(anything=w1248) -> (Variant=w1247:variant)
                          n428 = Variant To Flattened String(Variant=w1247) -> (data string=w1249:string)  [unwired: 1 out]
                          n429 = Flattened String To Variant(6:w1249, 7:w1251) -> (3:w1250:variant)  [unwired: 1 in, 1 out]
                        }
                        frame Error {
                        }
                      }
                    }
                    frame 48 {
                      # "STRING (0x30)"
                      n430 = Variant To Data(type="", Variant=w1254) -> (data=w1256:string, error out=w1258:errorcluster)  [unwired: 1 in]
                      n431 = case shown="No Error" w1258 {
                        tunnel: w1261 -> [w1269 _]
                        tunnel: [w1268 w1270] -> w1259
                        tunnel: w1257 -> [_ w1270]
                        tunnel: w1256 -> [w1265 _]
                        tunnel: w1255 -> [w1263 _]
                        tunnel: [TRUE _] -> w1253
                        frame No Error {
                          n432 = Fract/Exp String To Number(string=w1265, default (0 dbl)=w1263) -> (number=w1264:sgl)  [unwired: 2 in, 1 out]
                          n433 = To Variant(anything=w1264) -> (Variant=w1267:variant)
                          n434 = Variant To Flattened String(Variant=w1267) -> (data string=w1266:string)  [unwired: 1 out]
                          n435 = Flattened String To Variant(6:w1266, 7:w1269) -> (3:w1268:variant)  [unwired: 1 in, 1 out]
                        }
                        frame Error {
                        }
                      }
                    }
                  }
                }
              }
            }
            frame 10 {
              # "DBL (0xA)"
              n436 = Variant To Flattened String(Variant=w1277) -> (1:w1281:i16[])  [unwired: 1 out]
              n437 = call "TypeDescriptor_GetType.vi"("type descriptor"=w1281) -> ("Type"=w1271:u8)  [unwired: 9 in, 1 out]
              n438 = Equal?(x=w1272, y=w1271) -> (x = y?=w1275:bool)
              n439 = Compound Arithmetic op=OR(w1275, invert w1273) -> (w1274:bool)
              n440 = case shown="True" w1274 {
                tunnel: w1280 -> [w1282 w1289]
                tunnel: [w1282 w1288] -> w1279
                tunnel: w1278 -> [_ w1287]
                tunnel: w1271 -> [_ w1286]
                tunnel: w1277 -> [_ w1284]
                tunnel: [_ w1283] -> w1276
                frame False {
                }
                frame True {
                  w1285 = 0.0  # DBL
                  n441 = case shown="1..8" w1286 {
                    tunnel: w1289 -> [w1290 _ w1300 w1315 w1330 w1345]
                    tunnel: [w1290 w1292 w1302 w1317 w1332 w1347] -> w1288
                    tunnel: w1287 -> [_ w1293 w1303 w1318 w1333 w1349]
                    tunnel: w1285 -> [_ _ w1298 w1313 w1328 w1343]
                    tunnel: w1284 -> [_ w1295 w1297 w1312 w1327 w1342]
                    tunnel: [_ TRUE w1296 w1311 w1326 w1341] -> w1283
                    frame Default {
                      # "INCOMPATIBLE DATATYPES"
                    }
                    frame 10 {
                      # "DBL (0x0A)"
                      n442 = Variant To Flattened String(Variant=w1295) -> (data string=w1294:string)  [unwired: 1 out]
                      n443 = Flattened String To Variant(6:w1294, 7:w1293) -> (3:w1292:variant)  [unwired: 1 in, 1 out]
                    }
                    frame 1..8 {
                      # "I8, I16, I32, I64, U8, U16, U32, U64"
                      n444 = Variant To Data(type=w1298, Variant=w1297) -> (data=w1299:dbl, error out=w1301:errorcluster)  [unwired: 1 in]
                      n445 = case shown="No Error" w1301 {
                        tunnel: w1303 -> [w1309 _]
                        tunnel: [w1308 w1310] -> w1302
                        tunnel: w1300 -> [_ w1310]
                        tunnel: w1299 -> [w1306 _]
                        tunnel: [TRUE _] -> w1296
                        frame No Error {
                          n446 = To Variant(anything=w1306) -> (Variant=w1305:variant)
                          n447 = Variant To Flattened String(Variant=w1305) -> (data string=w1307:string)  [unwired: 1 out]
                          n448 = Flattened String To Variant(6:w1307, 7:w1309) -> (3:w1308:variant)  [unwired: 1 in, 1 out]
                        }
                        frame Error {
                        }
                      }
                    }
                    frame 9, 11..14 {
                      # "SGL, EXT, CSG, CDB, CXT (0x09 .. 0x0E)"
                      n449 = Variant To Data(type=w1313, Variant=w1312) -> (data=w1314:dbl, error out=w1316:errorcluster)  [unwired: 1 in]
                      n450 = case shown="No Error" w1316 {
                        tunnel: w1318 -> [w1324 _]
                        tunnel: [w1323 w1325] -> w1317
                        tunnel: w1315 -> [_ w1325]
                        tunnel: w1314 -> [w1321 _]
                        tunnel: [TRUE _] -> w1311
                        frame No Error {
                          n451 = To Variant(anything=w1321) -> (Variant=w1320:variant)
                          n452 = Variant To Flattened String(Variant=w1320) -> (data string=w1322:string)  [unwired: 1 out]
                          n453 = Flattened String To Variant(6:w1322, 7:w1324) -> (3:w1323:variant)  [unwired: 1 in, 1 out]
                        }
                        frame Error {
                        }
                      }
                    }
                    frame 25..30 {
                      # "Physical Units (0x19 .. 0x1E)"
                      n454 = Variant To Data(type=w1328, Variant=w1327) -> (data=w1329:dbl, error out=w1331:errorcluster)  [unwired: 1 in]
                      n455 = case shown="No Error" w1331 {
                        tunnel: w1333 -> [w1339 _]
                        tunnel: [w1338 w1340] -> w1332
                        tunnel: w1330 -> [_ w1340]
                        tunnel: w1329 -> [w1336 _]
                        tunnel: [TRUE _] -> w1326
                        frame No Error {
                          n456 = To Variant(anything=w1336) -> (Variant=w1335:variant)
                          n457 = Variant To Flattened String(Variant=w1335) -> (data string=w1337:string)  [unwired: 1 out]
                          n458 = Flattened String To Variant(6:w1337, 7:w1339) -> (3:w1338:variant)  [unwired: 1 in, 1 out]
                        }
                        frame Error {
                        }
                      }
                    }
                    frame 48 {
                      # "STRING (0x30)"
                      n459 = Variant To Data(type="", Variant=w1342) -> (data=w1344:string, error out=w1346:errorcluster)  [unwired: 1 in]
                      n460 = case shown="No Error" w1346 {
                        tunnel: w1349 -> [w1357 _]
                        tunnel: [w1356 w1358] -> w1347
                        tunnel: w1345 -> [_ w1358]
                        tunnel: w1344 -> [w1353 _]
                        tunnel: w1343 -> [w1351 _]
                        tunnel: [TRUE _] -> w1341
                        frame No Error {
                          n461 = Fract/Exp String To Number(string=w1353, default (0 dbl)=w1351) -> (number=w1352:dbl)  [unwired: 2 in, 1 out]
                          n462 = To Variant(anything=w1352) -> (Variant=w1355:variant)
                          n463 = Variant To Flattened String(Variant=w1355) -> (data string=w1354:string)  [unwired: 1 out]
                          n464 = Flattened String To Variant(6:w1354, 7:w1357) -> (3:w1356:variant)  [unwired: 1 in, 1 out]
                        }
                        frame Error {
                        }
                      }
                    }
                  }
                }
              }
            }
            frame 11 {
              # "EXT (0x0B)"
              n465 = Variant To Flattened String(Variant=w1365) -> (1:w1369:i16[])  [unwired: 1 out]
              n466 = call "TypeDescriptor_GetType.vi"("type descriptor"=w1369) -> ("Type"=w1360:u8)  [unwired: 9 in, 1 out]
              n467 = Equal?(x=w1361, y=w1360) -> (x = y?=w1363:bool)
              n468 = Compound Arithmetic op=OR(w1363, invert w1359) -> (w1362:bool)
              n469 = case shown="True" w1362 {
                tunnel: w1368 -> [w1370 w1377]
                tunnel: [w1370 w1376] -> w1367
                tunnel: w1366 -> [_ w1375]
                tunnel: w1360 -> [_ w1374]
                tunnel: w1365 -> [_ w1372]
                tunnel: [_ w1371] -> w1364
                frame False {
                }
                frame True {
                  w1373 = ext 0.0  # EXT
                  n470 = case shown="1..8" w1374 {
                    tunnel: w1377 -> [w1378 _ w1388 w1403 w1418 w1433]
                    tunnel: [w1378 w1379 w1390 w1405 w1420 w1435] -> w1376
                    tunnel: w1375 -> [_ w1381 w1391 w1406 w1421 w1437]
                    tunnel: w1373 -> [_ _ w1386 w1401 w1416 w1431]
                    tunnel: w1372 -> [_ w1383 w1385 w1400 w1415 w1430]
                    tunnel: [_ TRUE w1384 w1399 w1414 w1429] -> w1371
                    frame Default {
                      # "INCOMPATIBLE DATATYPES"
                    }
                    frame 11 {
                      # "EXT (0x0B)"
                      n471 = Variant To Flattened String(Variant=w1383) -> (data string=w1382:string)  [unwired: 1 out]
                      n472 = Flattened String To Variant(6:w1382, 7:w1381) -> (3:w1379:variant)  [unwired: 1 in, 1 out]
                    }
                    frame 1..8 {
                      # "I8, I16, I32, I64, U8, U16, U32, U64"
                      n473 = Variant To Data(type=w1386, Variant=w1385) -> (data=w1387:ext, error out=w1389:errorcluster)  [unwired: 1 in]
                      n474 = case shown="No Error" w1389 {
                        tunnel: w1391 -> [w1397 _]
                        tunnel: [w1396 w1398] -> w1390
                        tunnel: w1388 -> [_ w1398]
                        tunnel: w1387 -> [w1394 _]
                        tunnel: [TRUE _] -> w1384
                        frame No Error {
                          n475 = To Variant(anything=w1394) -> (Variant=w1393:variant)
                          n476 = Variant To Flattened String(Variant=w1393) -> (data string=w1395:string)  [unwired: 1 out]
                          n477 = Flattened String To Variant(6:w1395, 7:w1397) -> (3:w1396:variant)  [unwired: 1 in, 1 out]
                        }
                        frame Error {
                        }
                      }
                    }
                    frame 9, 10, 12..14 {
                      # "SGL, DBL, CSG, CDB, CXT (0x09 .. 0x0E)"
                      n478 = Variant To Data(type=w1401, Variant=w1400) -> (data=w1402:ext, error out=w1404:errorcluster)  [unwired: 1 in]
                      n479 = case shown="No Error" w1404 {
                        tunnel: w1406 -> [w1412 _]
                        tunnel: [w1411 w1413] -> w1405
                        tunnel: w1403 -> [_ w1413]
                        tunnel: w1402 -> [w1409 _]
                        tunnel: [TRUE _] -> w1399
                        frame No Error {
                          n480 = To Variant(anything=w1409) -> (Variant=w1408:variant)
                          n481 = Variant To Flattened String(Variant=w1408) -> (data string=w1410:string)  [unwired: 1 out]
                          n482 = Flattened String To Variant(6:w1410, 7:w1412) -> (3:w1411:variant)  [unwired: 1 in, 1 out]
                        }
                        frame Error {
                        }
                      }
                    }
                    frame 25..30 {
                      # "Physical Units (0x19 .. 0x1E)"
                      n483 = Variant To Data(type=w1416, Variant=w1415) -> (data=w1417:ext, error out=w1419:errorcluster)  [unwired: 1 in]
                      n484 = case shown="No Error" w1419 {
                        tunnel: w1421 -> [w1427 _]
                        tunnel: [w1426 w1428] -> w1420
                        tunnel: w1418 -> [_ w1428]
                        tunnel: w1417 -> [w1424 _]
                        tunnel: [TRUE _] -> w1414
                        frame No Error {
                          n485 = To Variant(anything=w1424) -> (Variant=w1423:variant)
                          n486 = Variant To Flattened String(Variant=w1423) -> (data string=w1425:string)  [unwired: 1 out]
                          n487 = Flattened String To Variant(6:w1425, 7:w1427) -> (3:w1426:variant)  [unwired: 1 in, 1 out]
                        }
                        frame Error {
                        }
                      }
                    }
                    frame 48 {
                      # "STRING (0x30)"
                      n488 = Variant To Data(type="", Variant=w1430) -> (data=w1432:string, error out=w1434:errorcluster)  [unwired: 1 in]
                      n489 = case shown="No Error" w1434 {
                        tunnel: w1437 -> [w1445 _]
                        tunnel: [w1444 w1446] -> w1435
                        tunnel: w1433 -> [_ w1446]
                        tunnel: w1432 -> [w1441 _]
                        tunnel: w1431 -> [w1439 _]
                        tunnel: [TRUE _] -> w1429
                        frame No Error {
                          n490 = Fract/Exp String To Number(string=w1441, default (0 dbl)=w1439) -> (number=w1440:ext)  [unwired: 2 in, 1 out]
                          n491 = To Variant(anything=w1440) -> (Variant=w1443:variant)
                          n492 = Variant To Flattened String(Variant=w1443) -> (data string=w1442:string)  [unwired: 1 out]
                          n493 = Flattened String To Variant(6:w1442, 7:w1445) -> (3:w1444:variant)  [unwired: 1 in, 1 out]
                        }
                        frame Error {
                        }
                      }
                    }
                  }
                }
              }
            }
            frame 12 {
              # "CSG (0x0C)"
              n494 = Variant To Flattened String(Variant=w1453) -> (1:w1457:i16[])  [unwired: 1 out]
              n495 = call "TypeDescriptor_GetType.vi"("type descriptor"=w1457) -> ("Type"=w1448:u8)  [unwired: 9 in, 1 out]
              n496 = Equal?(x=w1449, y=w1448) -> (x = y?=w1451:bool)
              n497 = Compound Arithmetic op=OR(w1451, invert w1447) -> (w1450:bool)
              n498 = case shown="True" w1450 {
                tunnel: w1456 -> [w1458 w1465]
                tunnel: [w1458 w1464] -> w1455
                tunnel: w1454 -> [_ w1463]
                tunnel: w1448 -> [_ w1462]
                tunnel: w1453 -> [_ w1460]
                tunnel: [_ w1459] -> w1452
                frame False {
                }
                frame True {
                  w1461 = csg 0.0+0.0i  # CSG
                  n499 = case shown="1..8" w1462 {
                    tunnel: w1465 -> [w1466 _ w1476 w1491 w1506]
                    tunnel: [w1466 w1467 w1478 w1493 w1508] -> w1464
                    tunnel: w1463 -> [_ w1469 w1479 w1494 w1509]
                    tunnel: w1461 -> [_ _ w1474 w1489 w1504]
                    tunnel: w1460 -> [_ w1471 w1473 w1488 w1503]
                    tunnel: [_ TRUE w1472 w1487 w1502] -> w1459
                    frame Default {
                      # "INCOMPATIBLE DATATYPES"
                    }
                    frame 12 {
                      # "CSG (0x0C)"
                      n500 = Variant To Flattened String(Variant=w1471) -> (data string=w1470:string)  [unwired: 1 out]
                      n501 = Flattened String To Variant(6:w1470, 7:w1469) -> (3:w1467:variant)  [unwired: 1 in, 1 out]
                    }
                    frame 1..8 {
                      # "I8, I16, I32, I64, U8, U16, U32, U64"
                      n502 = Variant To Data(type=w1474, Variant=w1473) -> (data=w1475:csg, error out=w1477:errorcluster)  [unwired: 1 in]
                      n503 = case shown="No Error" w1477 {
                        tunnel: w1479 -> [w1485 _]
                        tunnel: [w1484 w1486] -> w1478
                        tunnel: w1476 -> [_ w1486]
                        tunnel: w1475 -> [w1482 _]
                        tunnel: [TRUE _] -> w1472
                        frame No Error {
                          n504 = To Variant(anything=w1482) -> (Variant=w1481:variant)
                          n505 = Variant To Flattened String(Variant=w1481) -> (data string=w1483:string)  [unwired: 1 out]
                          n506 = Flattened String To Variant(6:w1483, 7:w1485) -> (3:w1484:variant)  [unwired: 1 in, 1 out]
                        }
                        frame Error {
                        }
                      }
                    }
                    frame 9..11, 13, 14 {
                      # "SGL, DBL, EXT, CDB, CXT (0x09 .. 0x0E)"
                      n507 = Variant To Data(type=w1489, Variant=w1488) -> (data=w1490:csg, error out=w1492:errorcluster)  [unwired: 1 in]
                      n508 = case shown="No Error" w1492 {
                        tunnel: w1494 -> [w1500 _]
                        tunnel: [w1499 w1501] -> w1493
                        tunnel: w1491 -> [_ w1501]
                        tunnel: w1490 -> [w1497 _]
                        tunnel: [TRUE _] -> w1487
                        frame No Error {
                          n509 = To Variant(anything=w1497) -> (Variant=w1496:variant)
                          n510 = Variant To Flattened String(Variant=w1496) -> (data string=w1498:string)  [unwired: 1 out]
                          n511 = Flattened String To Variant(6:w1498, 7:w1500) -> (3:w1499:variant)  [unwired: 1 in, 1 out]
                        }
                        frame Error {
                        }
                      }
                    }
                    frame 25..30 {
                      # "Physical Units (0x19 .. 0x1E)"
                      n512 = Variant To Data(type=w1504, Variant=w1503) -> (data=w1505:csg, error out=w1507:errorcluster)  [unwired: 1 in]
                      n513 = case shown="No Error" w1507 {
                        tunnel: w1509 -> [w1515 _]
                        tunnel: [w1514 w1516] -> w1508
                        tunnel: w1506 -> [_ w1516]
                        tunnel: w1505 -> [w1512 _]
                        tunnel: [TRUE _] -> w1502
                        frame No Error {
                          n514 = To Variant(anything=w1512) -> (Variant=w1511:variant)
                          n515 = Variant To Flattened String(Variant=w1511) -> (data string=w1513:string)  [unwired: 1 out]
                          n516 = Flattened String To Variant(6:w1513, 7:w1515) -> (3:w1514:variant)  [unwired: 1 in, 1 out]
                        }
                        frame Error {
                        }
                      }
                    }
                  }
                }
              }
            }
            frame 13 {
              # "CDB (0x0D)"
              n517 = Variant To Flattened String(Variant=w1524) -> (1:w1527:i16[])  [unwired: 1 out]
              n518 = call "TypeDescriptor_GetType.vi"("type descriptor"=w1527) -> ("Type"=w1517:u8)  [unwired: 9 in, 1 out]
              n519 = Equal?(x=w1519, y=w1517) -> (x = y?=w1521:bool)
              n520 = Compound Arithmetic op=OR(w1521, invert w1518) -> (w1520:bool)
              n521 = case shown="True" w1520 {
                tunnel: [w1528 w1534] -> w1526
                tunnel: w1525 -> [_ w1533]
                tunnel: w1517 -> [_ w1532]
                tunnel: w1524 -> [_ w1530]
                tunnel: [_ w1529] -> w1523
                tunnel: w1522 -> [w1528 w1535]
                frame False {
                }
                frame True {
                  w1531 = cdb 0.0+0.0i  # CDB
                  n522 = case shown="1..8" w1532 {
                    tunnel: w1535 -> [w1536 _ w1546 w1561 w1576]
                    tunnel: [w1536 w1537 w1548 w1563 w1578] -> w1534
                    tunnel: w1533 -> [_ w1539 w1549 w1564 w1579]
                    tunnel: w1531 -> [_ _ w1544 w1559 w1574]
                    tunnel: w1530 -> [_ w1541 w1543 w1558 w1573]
                    tunnel: [_ TRUE w1542 w1557 w1572] -> w1529
                    frame Default {
                      # "INCOMPATIBLE DATATYPES"
                    }
                    frame 13 {
                      # "CDB (0x0D)"
                      n523 = Variant To Flattened String(Variant=w1541) -> (data string=w1540:string)  [unwired: 1 out]
                      n524 = Flattened String To Variant(6:w1540, 7:w1539) -> (3:w1537:variant)  [unwired: 1 in, 1 out]
                    }
                    frame 1..8 {
                      # "I8, I16, I32, I64, U8, U16, U32, U64"
                      n525 = Variant To Data(type=w1544, Variant=w1543) -> (data=w1545:cdb, error out=w1547:errorcluster)  [unwired: 1 in]
                      n526 = case shown="No Error" w1547 {
                        tunnel: w1549 -> [w1555 _]
                        tunnel: [w1554 w1556] -> w1548
                        tunnel: w1546 -> [_ w1556]
                        tunnel: w1545 -> [w1552 _]
                        tunnel: [TRUE _] -> w1542
                        frame No Error {
                          n527 = To Variant(anything=w1552) -> (Variant=w1551:variant)
                          n528 = Variant To Flattened String(Variant=w1551) -> (data string=w1553:string)  [unwired: 1 out]
                          n529 = Flattened String To Variant(6:w1553, 7:w1555) -> (3:w1554:variant)  [unwired: 1 in, 1 out]
                        }
                        frame Error {
                        }
                      }
                    }
                    frame 9..12, 14 {
                      # "SGL, DBL, EXT, CSG, CXT (0x09 .. 0x0E)"
                      n530 = Variant To Data(type=w1559, Variant=w1558) -> (data=w1560:cdb, error out=w1562:errorcluster)  [unwired: 1 in]
                      n531 = case shown="No Error" w1562 {
                        tunnel: w1564 -> [w1570 _]
                        tunnel: [w1569 w1571] -> w1563
                        tunnel: w1561 -> [_ w1571]
                        tunnel: w1560 -> [w1567 _]
                        tunnel: [TRUE _] -> w1557
                        frame No Error {
                          n532 = To Variant(anything=w1567) -> (Variant=w1566:variant)
                          n533 = Variant To Flattened String(Variant=w1566) -> (data string=w1568:string)  [unwired: 1 out]
                          n534 = Flattened String To Variant(6:w1568, 7:w1570) -> (3:w1569:variant)  [unwired: 1 in, 1 out]
                        }
                        frame Error {
                        }
                      }
                    }
                    frame 25..30 {
                      # "Physical Units (0x19 .. 0x1E)"
                      n535 = Variant To Data(type=w1574, Variant=w1573) -> (data=w1575:cdb, error out=w1577:errorcluster)  [unwired: 1 in]
                      n536 = case shown="No Error" w1577 {
                        tunnel: w1579 -> [w1585 _]
                        tunnel: [w1584 w1586] -> w1578
                        tunnel: w1576 -> [_ w1586]
                        tunnel: w1575 -> [w1582 _]
                        tunnel: [TRUE _] -> w1572
                        frame No Error {
                          n537 = To Variant(anything=w1582) -> (Variant=w1581:variant)
                          n538 = Variant To Flattened String(Variant=w1581) -> (data string=w1583:string)  [unwired: 1 out]
                          n539 = Flattened String To Variant(6:w1583, 7:w1585) -> (3:w1584:variant)  [unwired: 1 in, 1 out]
                        }
                        frame Error {
                        }
                      }
                    }
                  }
                }
              }
            }
            frame 14 {
              # "CXT (0x0E)"
              n540 = Variant To Flattened String(Variant=w1593) -> (1:w1597:i16[])  [unwired: 1 out]
              n541 = call "TypeDescriptor_GetType.vi"("type descriptor"=w1597) -> ("Type"=w1587:u8)  [unwired: 9 in, 1 out]
              n542 = Equal?(x=w1588, y=w1587) -> (x = y?=w1591:bool)
              n543 = Compound Arithmetic op=OR(w1591, invert w1589) -> (w1590:bool)
              n544 = case shown="True" w1590 {
                tunnel: w1596 -> [w1598 w1605]
                tunnel: [w1598 w1604] -> w1595
                tunnel: w1594 -> [_ w1603]
                tunnel: w1587 -> [_ w1602]
                tunnel: w1593 -> [_ w1600]
                tunnel: [_ w1599] -> w1592
                frame False {
                }
                frame True {
                  w1601 = cxt 0.0+0.0i  # CXT
                  n545 = case shown="1..8" w1602 {
                    tunnel: w1605 -> [w1606 _ w1616 w1631 w1646]
                    tunnel: [w1606 w1607 w1618 w1633 w1648] -> w1604
                    tunnel: w1603 -> [_ w1609 w1619 w1634 w1649]
                    tunnel: w1601 -> [_ _ w1614 w1629 w1644]
                    tunnel: w1600 -> [_ w1611 w1613 w1628 w1643]
                    tunnel: [_ TRUE w1612 w1627 w1642] -> w1599
                    frame Default {
                      # "INCOMPATIBLE DATATYPES"
                    }
                    frame 14 {
                      # "CXT (0x0E)"
                      n546 = Variant To Flattened String(Variant=w1611) -> (data string=w1610:string)  [unwired: 1 out]
                      n547 = Flattened String To Variant(6:w1610, 7:w1609) -> (3:w1607:variant)  [unwired: 1 in, 1 out]
                    }
                    frame 1..8 {
                      # "I8, I16, I32, I64, U8, U16, U32, U64"
                      n548 = Variant To Data(type=w1614, Variant=w1613) -> (data=w1615:cxt, error out=w1617:errorcluster)  [unwired: 1 in]
                      n549 = case shown="No Error" w1617 {
                        tunnel: w1619 -> [w1625 _]
                        tunnel: [w1624 w1626] -> w1618
                        tunnel: w1616 -> [_ w1626]
                        tunnel: w1615 -> [w1622 _]
                        tunnel: [TRUE _] -> w1612
                        frame No Error {
                          n550 = To Variant(anything=w1622) -> (Variant=w1621:variant)
                          n551 = Variant To Flattened String(Variant=w1621) -> (data string=w1623:string)  [unwired: 1 out]
                          n552 = Flattened String To Variant(6:w1623, 7:w1625) -> (3:w1624:variant)  [unwired: 1 in, 1 out]
                        }
                        frame Error {
                        }
                      }
                    }
                    frame 9..13 {
                      # "SGL, DBL, EXT, CSG, CDB (0x09 .. 0x0E)"
                      n553 = Variant To Data(type=w1629, Variant=w1628) -> (data=w1630:cxt, error out=w1632:errorcluster)  [unwired: 1 in]
                      n554 = case shown="No Error" w1632 {
                        tunnel: w1634 -> [w1640 _]
                        tunnel: [w1639 w1641] -> w1633
                        tunnel: w1631 -> [_ w1641]
                        tunnel: w1630 -> [w1637 _]
                        tunnel: [TRUE _] -> w1627
                        frame No Error {
                          n555 = To Variant(anything=w1637) -> (Variant=w1636:variant)
                          n556 = Variant To Flattened String(Variant=w1636) -> (data string=w1638:string)  [unwired: 1 out]
                          n557 = Flattened String To Variant(6:w1638, 7:w1640) -> (3:w1639:variant)  [unwired: 1 in, 1 out]
                        }
                        frame Error {
                        }
                      }
                    }
                    frame 25..30 {
                      # "Physical Units (0x19 .. 0x1E)"
                      n558 = Variant To Data(type=w1644, Variant=w1643) -> (data=w1645:cxt, error out=w1647:errorcluster)  [unwired: 1 in]
                      n559 = case shown="No Error" w1647 {
                        tunnel: w1649 -> [w1655 _]
                        tunnel: [w1654 w1656] -> w1648
                        tunnel: w1646 -> [_ w1656]
                        tunnel: w1645 -> [w1652 _]
                        tunnel: [TRUE _] -> w1642
                        frame No Error {
                          n560 = To Variant(anything=w1652) -> (Variant=w1651:variant)
                          n561 = Variant To Flattened String(Variant=w1651) -> (data string=w1653:string)  [unwired: 1 out]
                          n562 = Flattened String To Variant(6:w1653, 7:w1655) -> (3:w1654:variant)  [unwired: 1 in, 1 out]
                        }
                        frame Error {
                        }
                      }
                    }
                  }
                }
              }
            }
            frame 23 {
              # "Enum U32 (0x17)"
              n563 = Variant To Flattened String(Variant=w1663) -> (1:w1667:i16[])  [unwired: 1 out]
              n564 = call "TypeDescriptor_GetType.vi"("type descriptor"=w1667) -> ("Type"=w1657:u8)  [unwired: 9 in, 1 out]
              n565 = Equal?(x=w1658, y=w1657) -> (x = y?=w1661:bool)
              n566 = Compound Arithmetic op=OR(w1661, invert w1659) -> (w1660:bool)
              n567 = case shown="True" w1660 {
                tunnel: w1666 -> [w1668 w1670]
                tunnel: [w1668 w1675] -> w1665
                tunnel: w1664 -> [_ w1674]
                tunnel: w1657 -> [_ w1673]
                tunnel: w1663 -> [_ w1669]
                tunnel: [_ w1671] -> w1662
                frame False {
                }
                frame True {
                  w1672 = u32 0  # U32
                  n568 = case shown="30" w1673 {
                    tunnel: w1670 -> [w1676 w1678 _ _ _ w1714 w1736 w1751]
                    tunnel: [w1676 w1684 w1695 w1704 w1712 w1722 w1738 w1753] -> w1675
                    tunnel: w1674 -> [_ w1677 w1696 w1697 w1705 w1719 w1739 w1754]
                    tunnel: w1672 -> [_ w1681 _ _ _ w1716 w1734 w1749]
                    tunnel: w1669 -> [_ w1680 w1693 w1702 w1710 w1720 w1733 w1748]
                    tunnel: [_ w1679 TRUE TRUE TRUE w1713 w1732 w1747] -> w1671
                    frame Default {
                      # "INCOMPATIBLE DATATYPES"
                    }
                    frame 1..8 {
                      # "I8, I16, I32, I64, U8, U16, U32, U64"
                      n569 = Variant To Data(type=w1681, Variant=w1680) -> (data=w1682:u32, error out=w1683:errorcluster)  [unwired: 1 in]
                      n570 = case shown="No Error" w1683 {
                        tunnel: w1677 -> [w1690 _]
                        tunnel: [w1689 w1691] -> w1684
                        tunnel: w1678 -> [_ w1691]
                        tunnel: w1682 -> [w1687 _]
                        tunnel: [TRUE _] -> w1679
                        frame No Error {
                          n571 = To Variant(anything=w1687) -> (Variant=w1686:variant)
                          n572 = Variant To Flattened String(Variant=w1686) -> (data string=w1688:string)  [unwired: 1 out]
                          n573 = Flattened String To Variant(6:w1688, 7:w1690) -> (3:w1689:variant)  [unwired: 1 in, 1 out]
                        }
                        frame Error {
                        }
                      }
                    }
                    frame 23 {
                      # "Enum U32"
                      n574 = Variant To Flattened String(Variant=w1693) -> (data string=w1692:string)  [unwired: 1 out]
                      n575 = Flattened String To Variant(6:w1692, 7:w1696) -> (3:w1695:variant)  [unwired: 1 in, 1 out]
                    }
                    frame 22 {
                      # "Enum U16"
                      n576 = Variant To Flattened String(Variant=w1702) -> (data string=w1701:string)  [unwired: 1 out]
                      n577 = Byte Array To String(unsigned byte array=u8[] [0, 0]) -> (string=w1700:string)
                      n578 = Concatenate Strings(w1700, w1701) -> (w1698:string)
                      n579 = Flattened String To Variant(6:w1698, 7:w1697) -> (3:w1704:variant)  [unwired: 1 in, 1 out]
                    }
                    frame 21 {
                      # "Enum U8"
                      n580 = Variant To Flattened String(Variant=w1710) -> (data string=w1709:string)  [unwired: 1 out]
                      n581 = Byte Array To String(unsigned byte array=u8[] [0, 0, 0]) -> (string=w1708:string)
                      n582 = Concatenate Strings(w1708, w1709) -> (w1706:string)
                      n583 = Flattened String To Variant(6:w1706, 7:w1705) -> (3:w1712:variant)  [unwired: 1 in, 1 out]
                    }
                    frame 48 {
                      # "String (0x30)"
                      n584 = call "TypeDescriptor_ListElementNames.vi"("type descriptor"=w1719) -> ("element names"=w1718:string[])  [unwired: 7 in, 3 out]
                      n585 = Variant To Data(type="", Variant=w1720) -> (data=w1717:string)  [unwired: 1 in, 1 out]
                      n586 = Search 1D Array(1D array=w1718, element=w1717) -> (index of element=w1715:i32)  [unwired: 1 in]
                      n587 = case shown="Default" w1715 {
                        selector: w1715 -> [_ w1725]
                        tunnel: [w1723 w1731] -> w1722
                        tunnel: w1719 -> [_ w1730]
                        tunnel: w1716 -> [_ w1728]
                        tunnel: w1714 -> [w1723 _]
                        tunnel: [_ TRUE] -> w1713
                        frame -1 {
                        }
                        frame Default {
                          n588 = Variant To Data(type=w1728, Variant=w1725) -> (data=w1727:u32)  [unwired: 1 in, 1 out]
                          n589 = To Variant(anything=w1727) -> (Variant=w1729:variant)
                          n590 = Variant To Flattened String(Variant=w1729) -> (data string=w1726:string)  [unwired: 1 out]
                          n591 = Flattened String To Variant(6:w1726, 7:w1730) -> (3:w1731:variant)  [unwired: 1 in, 1 out]
                        }
                      }
                    }
                    frame 9..13 {
                      # "SGL, DBL, EXT, CSG, CDB (0x09 .. 0x0E)"
                      n592 = Variant To Data(type=w1734, Variant=w1733) -> (data=w1735:u32, error out=w1737:errorcluster)  [unwired: 1 in]
                      n593 = case shown="No Error" w1737 {
                        tunnel: w1739 -> [w1745 _]
                        tunnel: [w1744 w1746] -> w1738
                        tunnel: w1736 -> [_ w1746]
                        tunnel: w1735 -> [w1742 _]
                        tunnel: [TRUE _] -> w1732
                        frame No Error {
                          n594 = To Variant(anything=w1742) -> (Variant=w1741:variant)
                          n595 = Variant To Flattened String(Variant=w1741) -> (data string=w1743:string)  [unwired: 1 out]
                          n596 = Flattened String To Variant(6:w1743, 7:w1745) -> (3:w1744:variant)  [unwired: 1 in, 1 out]
                        }
                        frame Error {
                        }
                      }
                    }
                    frame 25..30 {
                      # "Physical Units (0x19 .. 0x1E)"
                      n597 = Variant To Data(type=w1749, Variant=w1748) -> (data=w1750:u32, error out=w1752:errorcluster)  [unwired: 1 in]
                      n598 = case shown="No Error" w1752 {
                        tunnel: w1754 -> [w1760 _]
                        tunnel: [w1759 w1761] -> w1753
                        tunnel: w1751 -> [_ w1761]
                        tunnel: w1750 -> [w1757 _]
                        tunnel: [TRUE _] -> w1747
                        frame No Error {
                          n599 = To Variant(anything=w1757) -> (Variant=w1756:variant)
                          n600 = Variant To Flattened String(Variant=w1756) -> (data string=w1758:string)  [unwired: 1 out]
                          n601 = Flattened String To Variant(6:w1758, 7:w1760) -> (3:w1759:variant)  [unwired: 1 in, 1 out]
                        }
                        frame Error {
                        }
                      }
                    }
                  }
                }
              }
            }
            frame 22 {
              # "Enum U16 (0x16)"
              n602 = Variant To Flattened String(Variant=w1768) -> (1:w1772:i16[])  [unwired: 1 out]
              n603 = call "TypeDescriptor_GetType.vi"("type descriptor"=w1772) -> ("Type"=w1762:u8)  [unwired: 9 in, 1 out]
              n604 = Equal?(x=w1763, y=w1762) -> (x = y?=w1766:bool)
              n605 = Compound Arithmetic op=OR(w1766, invert w1764) -> (w1765:bool)
              n606 = case shown="True" w1765 {
                tunnel: w1771 -> [w1773 w1775]
                tunnel: [w1773 w1780] -> w1770
                tunnel: w1769 -> [_ w1779]
                tunnel: w1762 -> [_ w1778]
                tunnel: w1768 -> [_ w1774]
                tunnel: [_ w1776] -> w1767
                frame False {
                }
                frame True {
                  w1777 = u16 0  # U16
                  n607 = case shown="17" w1778 {
                    tunnel: w1775 -> [w1781 w1783 _ _ _ w1818 w1840 w1855]
                    tunnel: [w1781 w1789 w1800 w1808 w1816 w1826 w1842 w1857] -> w1780
                    tunnel: w1779 -> [_ w1782 w1801 w1805 w1809 w1823 w1843 w1858]
                    tunnel: w1777 -> [_ w1786 _ _ _ w1820 w1838 w1853]
                    tunnel: w1774 -> [_ w1785 w1798 w1806 w1814 w1824 w1837 w1852]
                    tunnel: [_ w1784 TRUE TRUE TRUE w1817 w1836 w1851] -> w1776
                    frame Default {
                      # "INCOMPATIBLE DATATYPES"
                    }
                    frame 1..8 {
                      # "I8, I16, I32, I64, U8, U16, U32, U64"
                      n608 = Variant To Data(type=w1786, Variant=w1785) -> (data=w1787:u16, error out=w1788:errorcluster)  [unwired: 1 in]
                      n609 = case shown="No Error" w1788 {
                        tunnel: w1782 -> [w1795 _]
                        tunnel: [w1794 w1796] -> w1789
                        tunnel: w1783 -> [_ w1796]
                        tunnel: w1787 -> [w1792 _]
                        tunnel: [TRUE _] -> w1784
                        frame No Error {
                          n610 = To Variant(anything=w1792) -> (Variant=w1791:variant)
                          n611 = Variant To Flattened String(Variant=w1791) -> (data string=w1793:string)  [unwired: 1 out]
                          n612 = Flattened String To Variant(6:w1793, 7:w1795) -> (3:w1794:variant)  [unwired: 1 in, 1 out]
                        }
                        frame Error {
                        }
                      }
                    }
                    frame 22 {
                      # "Enum U16"
                      n613 = Variant To Flattened String(Variant=w1798) -> (data string=w1797:string)  [unwired: 1 out]
                      n614 = Flattened String To Variant(6:w1797, 7:w1801) -> (3:w1800:variant)  [unwired: 1 in, 1 out]
                    }
                    frame 23 {
                      # "Enum U32"
                      n615 = Variant To Flattened String(Variant=w1806) -> (data string=w1804:string)  [unwired: 1 out]
                      n616 = String Subset(string=w1804, offset (0)=2) -> (substring=w1802:string)  [unwired: 1 in]
                      n617 = Flattened String To Variant(6:w1802, 7:w1805) -> (3:w1808:variant)  [unwired: 1 in, 1 out]
                    }
                    frame 21 {
                      # "Enum U8"
                      n618 = Variant To Flattened String(Variant=w1814) -> (data string=w1813:string)  [unwired: 1 out]
                      n619 = Byte Array To String(unsigned byte array=u8[] [0]) -> (string=w1812:string)
                      n620 = Concatenate Strings(w1812, w1813) -> (w1810:string)
                      n621 = Flattened String To Variant(6:w1810, 7:w1809) -> (3:w1816:variant)  [unwired: 1 in, 1 out]
                    }
                    frame 48 {
                      # "String (0x30)"
                      n622 = call "TypeDescriptor_ListElementNames.vi"("type descriptor"=w1823) -> ("element names"=w1822:string[])  [unwired: 7 in, 3 out]
                      n623 = Variant To Data(type="", Variant=w1824) -> (data=w1821:string)  [unwired: 1 in, 1 out]
                      n624 = Search 1D Array(1D array=w1822, element=w1821) -> (index of element=w1819:i32)  [unwired: 1 in]
                      n625 = case shown="Default" w1819 {
                        selector: w1819 -> [_ w1829]
                        tunnel: [w1827 w1835] -> w1826
                        tunnel: w1823 -> [_ w1834]
                        tunnel: w1820 -> [_ w1832]
                        tunnel: w1818 -> [w1827 _]
                        tunnel: [_ TRUE] -> w1817
                        frame -1 {
                        }
                        frame Default {
                          n626 = Variant To Data(type=w1832, Variant=w1829) -> (data=w1831:u16)  [unwired: 1 in, 1 out]
                          n627 = To Variant(anything=w1831) -> (Variant=w1833:variant)
                          n628 = Variant To Flattened String(Variant=w1833) -> (data string=w1830:string)  [unwired: 1 out]
                          n629 = Flattened String To Variant(6:w1830, 7:w1834) -> (3:w1835:variant)  [unwired: 1 in, 1 out]
                        }
                      }
                    }
                    frame 9..13 {
                      # "SGL, DBL, EXT, CSG, CDB (0x09 .. 0x0E)"
                      n630 = Variant To Data(type=w1838, Variant=w1837) -> (data=w1839:u16, error out=w1841:errorcluster)  [unwired: 1 in]
                      n631 = case shown="No Error" w1841 {
                        tunnel: w1843 -> [w1849 _]
                        tunnel: [w1848 w1850] -> w1842
                        tunnel: w1840 -> [_ w1850]
                        tunnel: w1839 -> [w1846 _]
                        tunnel: [TRUE _] -> w1836
                        frame No Error {
                          n632 = To Variant(anything=w1846) -> (Variant=w1845:variant)
                          n633 = Variant To Flattened String(Variant=w1845) -> (data string=w1847:string)  [unwired: 1 out]
                          n634 = Flattened String To Variant(6:w1847, 7:w1849) -> (3:w1848:variant)  [unwired: 1 in, 1 out]
                        }
                        frame Error {
                        }
                      }
                    }
                    frame 25..30 {
                      # "Physical Units (0x19 .. 0x1E)"
                      n635 = Variant To Data(type=w1853, Variant=w1852) -> (data=w1854:u16, error out=w1856:errorcluster)  [unwired: 1 in]
                      n636 = case shown="No Error" w1856 {
                        tunnel: w1858 -> [w1864 _]
                        tunnel: [w1863 w1865] -> w1857
                        tunnel: w1855 -> [_ w1865]
                        tunnel: w1854 -> [w1861 _]
                        tunnel: [TRUE _] -> w1851
                        frame No Error {
                          n637 = To Variant(anything=w1861) -> (Variant=w1860:variant)
                          n638 = Variant To Flattened String(Variant=w1860) -> (data string=w1862:string)  [unwired: 1 out]
                          n639 = Flattened String To Variant(6:w1862, 7:w1864) -> (3:w1863:variant)  [unwired: 1 in, 1 out]
                        }
                        frame Error {
                        }
                      }
                    }
                  }
                }
              }
            }
            frame 21 {
              # "Enum U8 (0x15)"
              n640 = Variant To Flattened String(Variant=w1872) -> (1:w1876:i16[])  [unwired: 1 out]
              n641 = call "TypeDescriptor_GetType.vi"("type descriptor"=w1876) -> ("Type"=w1866:u8)  [unwired: 9 in, 1 out]
              n642 = Equal?(x=w1867, y=w1866) -> (x = y?=w1870:bool)
              n643 = Compound Arithmetic op=OR(w1870, invert w1868) -> (w1869:bool)
              n644 = case shown="True" w1869 {
                tunnel: w1875 -> [w1877 w1879]
                tunnel: [w1877 w1884] -> w1874
                tunnel: w1873 -> [_ w1883]
                tunnel: w1866 -> [_ w1882]
                tunnel: w1872 -> [_ w1878]
                tunnel: [_ w1880] -> w1871
                frame False {
                }
                frame True {
                  w1881 = u8 0  # U8
                  n645 = case shown="30" w1882 {
                    tunnel: w1879 -> [w1885 w1887 _ _ _ w1921 w1943 w1958]
                    tunnel: [w1885 w1893 w1904 w1912 w1919 w1929 w1945 w1960] -> w1884
                    tunnel: w1883 -> [_ w1886 w1905 w1909 w1916 w1926 w1946 w1961]
                    tunnel: w1881 -> [_ w1890 _ _ _ w1923 w1941 w1956]
                    tunnel: w1878 -> [_ w1889 w1902 w1910 w1917 w1927 w1940 w1955]
                    tunnel: [_ w1888 TRUE TRUE TRUE w1920 w1939 w1954] -> w1880
                    frame Default {
                      # "INCOMPATIBLE DATATYPES"
                    }
                    frame 1..8 {
                      # "I8, I16, I32, I64, U8, U16, U32, U64"
                      n646 = Variant To Data(type=w1890, Variant=w1889) -> (data=w1891:u8, error out=w1892:errorcluster)  [unwired: 1 in]
                      n647 = case shown="No Error" w1892 {
                        tunnel: w1886 -> [w1899 _]
                        tunnel: [w1898 w1900] -> w1893
                        tunnel: w1887 -> [_ w1900]
                        tunnel: w1891 -> [w1896 _]
                        tunnel: [TRUE _] -> w1888
                        frame No Error {
                          n648 = To Variant(anything=w1896) -> (Variant=w1895:variant)
                          n649 = Variant To Flattened String(Variant=w1895) -> (data string=w1897:string)  [unwired: 1 out]
                          n650 = Flattened String To Variant(6:w1897, 7:w1899) -> (3:w1898:variant)  [unwired: 1 in, 1 out]
                        }
                        frame Error {
                        }
                      }
                    }
                    frame 21 {
                      # "Enum U8"
                      n651 = Variant To Flattened String(Variant=w1902) -> (data string=w1901:string)  [unwired: 1 out]
                      n652 = Flattened String To Variant(6:w1901, 7:w1905) -> (3:w1904:variant)  [unwired: 1 in, 1 out]
                    }
                    frame 23 {
                      # "Enum U32"
                      n653 = Variant To Flattened String(Variant=w1910) -> (data string=w1908:string)  [unwired: 1 out]
                      n654 = String Subset(string=w1908, offset (0)=3) -> (substring=w1906:string)  [unwired: 1 in]
                      n655 = Flattened String To Variant(6:w1906, 7:w1909) -> (3:w1912:variant)  [unwired: 1 in, 1 out]
                    }
                    frame 22 {
                      # "Enum U16"
                      n656 = Variant To Flattened String(Variant=w1917) -> (data string=w1915:string)  [unwired: 1 out]
                      n657 = String Subset(string=w1915, offset (0)=1) -> (substring=w1914:string)  [unwired: 1 in]
                      n658 = Flattened String To Variant(6:w1914, 7:w1916) -> (3:w1919:variant)  [unwired: 1 in, 1 out]
                    }
                    frame 48 {
                      # "String (0x30)"
                      n659 = call "TypeDescriptor_ListElementNames.vi"("type descriptor"=w1926) -> ("element names"=w1925:string[])  [unwired: 7 in, 3 out]
                      n660 = Variant To Data(type="", Variant=w1927) -> (data=w1924:string)  [unwired: 1 in, 1 out]
                      n661 = Search 1D Array(1D array=w1925, element=w1924) -> (index of element=w1922:i32)  [unwired: 1 in]
                      n662 = case shown="Default" w1922 {
                        selector: w1922 -> [_ w1932]
                        tunnel: [w1930 w1938] -> w1929
                        tunnel: w1926 -> [_ w1937]
                        tunnel: w1923 -> [_ w1935]
                        tunnel: w1921 -> [w1930 _]
                        tunnel: [_ TRUE] -> w1920
                        frame -1 {
                        }
                        frame Default {
                          n663 = Variant To Data(type=w1935, Variant=w1932) -> (data=w1934:u8)  [unwired: 1 in, 1 out]
                          n664 = To Variant(anything=w1934) -> (Variant=w1936:variant)
                          n665 = Variant To Flattened String(Variant=w1936) -> (data string=w1933:string)  [unwired: 1 out]
                          n666 = Flattened String To Variant(6:w1933, 7:w1937) -> (3:w1938:variant)  [unwired: 1 in, 1 out]
                        }
                      }
                    }
                    frame 9..13 {
                      # "SGL, DBL, EXT, CSG, CDB (0x09 .. 0x0E)"
                      n667 = Variant To Data(type=w1941, Variant=w1940) -> (data=w1942:u8, error out=w1944:errorcluster)  [unwired: 1 in]
                      n668 = case shown="No Error" w1944 {
                        tunnel: w1946 -> [w1952 _]
                        tunnel: [w1951 w1953] -> w1945
                        tunnel: w1943 -> [_ w1953]
                        tunnel: w1942 -> [w1949 _]
                        tunnel: [TRUE _] -> w1939
                        frame No Error {
                          n669 = To Variant(anything=w1949) -> (Variant=w1948:variant)
                          n670 = Variant To Flattened String(Variant=w1948) -> (data string=w1950:string)  [unwired: 1 out]
                          n671 = Flattened String To Variant(6:w1950, 7:w1952) -> (3:w1951:variant)  [unwired: 1 in, 1 out]
                        }
                        frame Error {
                        }
                      }
                    }
                    frame 25..30 {
                      # "Physical Units (0x19 .. 0x1E)"
                      n672 = Variant To Data(type=w1956, Variant=w1955) -> (data=w1957:u8, error out=w1959:errorcluster)  [unwired: 1 in]
                      n673 = case shown="No Error" w1959 {
                        tunnel: w1961 -> [w1967 _]
                        tunnel: [w1966 w1968] -> w1960
                        tunnel: w1958 -> [_ w1968]
                        tunnel: w1957 -> [w1964 _]
                        tunnel: [TRUE _] -> w1954
                        frame No Error {
                          n674 = To Variant(anything=w1964) -> (Variant=w1963:variant)
                          n675 = Variant To Flattened String(Variant=w1963) -> (data string=w1965:string)  [unwired: 1 out]
                          n676 = Flattened String To Variant(6:w1965, 7:w1967) -> (3:w1966:variant)  [unwired: 1 in, 1 out]
                        }
                        frame Error {
                        }
                      }
                    }
                  }
                }
              }
            }
            frame 25 {
              # "SGL PhysUnit (0x19)"
              n677 = Variant To Flattened String(Variant=w1975) -> (1:w1979:i16[])  [unwired: 1 out]
              n678 = call "TypeDescriptor_GetType.vi"("type descriptor"=w1979) -> ("Type"=w1970:u8)  [unwired: 9 in, 1 out]
              n679 = Equal?(x=w1969, y=w1970) -> (x = y?=w1973:bool)
              n680 = Compound Arithmetic op=OR(w1973, invert w1971) -> (w1972:bool)
              n681 = case shown="True" w1972 {
                tunnel: w1978 -> [w1980 w1987]
                tunnel: [w1980 w1986] -> w1977
                tunnel: w1976 -> [_ w1985]
                tunnel: w1970 -> [_ w1984]
                tunnel: w1975 -> [_ w1982]
                tunnel: [_ w1981] -> w1974
                frame False {
                }
                frame True {
                  w1983 = sgl 0.0  # SGL
                  n682 = case shown="1..8" w1984 {
                    tunnel: w1987 -> [w1988 _ w1998 w2013 w2028]
                    tunnel: [w1988 w1990 w2000 w2015 w2030] -> w1986
                    tunnel: w1985 -> [_ w1991 w2001 w2016 w2031]
                    tunnel: w1983 -> [_ _ w1996 w2011 w2026]
                    tunnel: w1982 -> [_ w1993 w1995 w2010 w2025]
                    tunnel: [_ TRUE w1994 w2009 w2024] -> w1981
                    frame Default {
                      # "INCOMPATIBLE DATATYPES"
                    }
                    frame 25 {
                      # "SGL PhysUnit (0x19)"
                      n683 = Variant To Flattened String(Variant=w1993) -> (data string=w1992:string)  [unwired: 1 out]
                      n684 = Flattened String To Variant(6:w1992, 7:w1991) -> (3:w1990:variant)  [unwired: 1 in, 1 out]
                    }
                    frame 1..8 {
                      # "I8, I16, I32, I64, U8, U16, U32, U64"
                      n685 = Variant To Data(type=w1996, Variant=w1995) -> (data=w1997:sgl, error out=w1999:errorcluster)  [unwired: 1 in]
                      n686 = case shown="No Error" w1999 {
                        tunnel: w2001 -> [w2007 _]
                        tunnel: [w2006 w2008] -> w2000
                        tunnel: w1998 -> [_ w2008]
                        tunnel: w1997 -> [w2004 _]
                        tunnel: [TRUE _] -> w1994
                        frame No Error {
                          n687 = To Variant(anything=w2004) -> (Variant=w2003:variant)
                          n688 = Variant To Flattened String(Variant=w2003) -> (data string=w2005:string)  [unwired: 1 out]
                          n689 = Flattened String To Variant(6:w2005, 7:w2007) -> (3:w2006:variant)  [unwired: 1 in, 1 out]
                        }
                        frame Error {
                        }
                      }
                    }
                    frame 9..14 {
                      # "SGL, DBL, EXT, CSG, CDB (0x09 .. 0x0E)"
                      n690 = Variant To Data(type=w2011, Variant=w2010) -> (data=w2012:sgl, error out=w2014:errorcluster)  [unwired: 1 in]
                      n691 = case shown="No Error" w2014 {
                        tunnel: w2016 -> [w2022 _]
                        tunnel: [w2021 w2023] -> w2015
                        tunnel: w2013 -> [_ w2023]
                        tunnel: w2012 -> [w2019 _]
                        tunnel: [TRUE _] -> w2009
                        frame No Error {
                          n692 = To Variant(anything=w2019) -> (Variant=w2018:variant)
                          n693 = Variant To Flattened String(Variant=w2018) -> (data string=w2020:string)  [unwired: 1 out]
                          n694 = Flattened String To Variant(6:w2020, 7:w2022) -> (3:w2021:variant)  [unwired: 1 in, 1 out]
                        }
                        frame Error {
                        }
                      }
                    }
                    frame 26..30 {
                      # "Physical Units (0x19 .. 0x1E)"
                      n695 = Variant To Data(type=w2026, Variant=w2025) -> (data=w2027:sgl, error out=w2029:errorcluster)  [unwired: 1 in]
                      n696 = case shown="No Error" w2029 {
                        tunnel: w2031 -> [w2037 _]
                        tunnel: [w2036 w2038] -> w2030
                        tunnel: w2028 -> [_ w2038]
                        tunnel: w2027 -> [w2034 _]
                        tunnel: [TRUE _] -> w2024
                        frame No Error {
                          n697 = To Variant(anything=w2034) -> (Variant=w2033:variant)
                          n698 = Variant To Flattened String(Variant=w2033) -> (data string=w2035:string)  [unwired: 1 out]
                          n699 = Flattened String To Variant(6:w2035, 7:w2037) -> (3:w2036:variant)  [unwired: 1 in, 1 out]
                        }
                        frame Error {
                        }
                      }
                    }
                  }
                }
              }
            }
            frame 26 {
              # "DBL PhysUnit (0x1A)"
              n700 = Variant To Flattened String(Variant=w2045) -> (1:w2049:i16[])  [unwired: 1 out]
              n701 = call "TypeDescriptor_GetType.vi"("type descriptor"=w2049) -> ("Type"=w2040:u8)  [unwired: 9 in, 1 out]
              n702 = Equal?(x=w2041, y=w2040) -> (x = y?=w2043:bool)
              n703 = Compound Arithmetic op=OR(w2043, invert w2039) -> (w2042:bool)
              n704 = case shown="True" w2042 {
                tunnel: w2048 -> [w2050 w2057]
                tunnel: [w2050 w2056] -> w2047
                tunnel: w2046 -> [_ w2055]
                tunnel: w2040 -> [_ w2054]
                tunnel: w2045 -> [_ w2052]
                tunnel: [_ w2051] -> w2044
                frame False {
                }
                frame True {
                  w2053 = 0.0  # DBL
                  n705 = case shown="1..8" w2054 {
                    tunnel: w2057 -> [w2058 _ w2068 w2083 w2098]
                    tunnel: [w2058 w2060 w2070 w2085 w2100] -> w2056
                    tunnel: w2055 -> [_ w2061 w2071 w2086 w2101]
                    tunnel: w2053 -> [_ _ w2066 w2081 w2096]
                    tunnel: w2052 -> [_ w2063 w2065 w2080 w2095]
                    tunnel: [_ TRUE w2064 w2079 w2094] -> w2051
                    frame Default {
                      # "INCOMPATIBLE DATATYPES"
                    }
                    frame 26 {
                      # "DBL PhysUnit (0x1A)"
                      n706 = Variant To Flattened String(Variant=w2063) -> (data string=w2062:string)  [unwired: 1 out]
                      n707 = Flattened String To Variant(6:w2062, 7:w2061) -> (3:w2060:variant)  [unwired: 1 in, 1 out]
                    }
                    frame 1..8 {
                      # "I8, I16, I32, I64, U8, U16, U32, U64"
                      n708 = Variant To Data(type=w2066, Variant=w2065) -> (data=w2067:dbl, error out=w2069:errorcluster)  [unwired: 1 in]
                      n709 = case shown="No Error" w2069 {
                        tunnel: w2071 -> [w2077 _]
                        tunnel: [w2076 w2078] -> w2070
                        tunnel: w2068 -> [_ w2078]
                        tunnel: w2067 -> [w2074 _]
                        tunnel: [TRUE _] -> w2064
                        frame No Error {
                          n710 = To Variant(anything=w2074) -> (Variant=w2073:variant)
                          n711 = Variant To Flattened String(Variant=w2073) -> (data string=w2075:string)  [unwired: 1 out]
                          n712 = Flattened String To Variant(6:w2075, 7:w2077) -> (3:w2076:variant)  [unwired: 1 in, 1 out]
                        }
                        frame Error {
                        }
                      }
                    }
                    frame 9..14 {
                      # "SGL, DBL, EXT, CSG, CDB (0x09 .. 0x0E)"
                      n713 = Variant To Data(type=w2081, Variant=w2080) -> (data=w2082:dbl, error out=w2084:errorcluster)  [unwired: 1 in]
                      n714 = case shown="No Error" w2084 {
                        tunnel: w2086 -> [w2092 _]
                        tunnel: [w2091 w2093] -> w2085
                        tunnel: w2083 -> [_ w2093]
                        tunnel: w2082 -> [w2089 _]
                        tunnel: [TRUE _] -> w2079
                        frame No Error {
                          n715 = To Variant(anything=w2089) -> (Variant=w2088:variant)
                          n716 = Variant To Flattened String(Variant=w2088) -> (data string=w2090:string)  [unwired: 1 out]
                          n717 = Flattened String To Variant(6:w2090, 7:w2092) -> (3:w2091:variant)  [unwired: 1 in, 1 out]
                        }
                        frame Error {
                        }
                      }
                    }
                    frame 25, 27..30 {
                      # "Physical Units (0x19 .. 0x1E)"
                      n718 = Variant To Data(type=w2096, Variant=w2095) -> (data=w2097:dbl, error out=w2099:errorcluster)  [unwired: 1 in]
                      n719 = case shown="No Error" w2099 {
                        tunnel: w2101 -> [w2107 _]
                        tunnel: [w2106 w2108] -> w2100
                        tunnel: w2098 -> [_ w2108]
                        tunnel: w2097 -> [w2104 _]
                        tunnel: [TRUE _] -> w2094
                        frame No Error {
                          n720 = To Variant(anything=w2104) -> (Variant=w2103:variant)
                          n721 = Variant To Flattened String(Variant=w2103) -> (data string=w2105:string)  [unwired: 1 out]
                          n722 = Flattened String To Variant(6:w2105, 7:w2107) -> (3:w2106:variant)  [unwired: 1 in, 1 out]
                        }
                        frame Error {
                        }
                      }
                    }
                  }
                }
              }
            }
            frame 27 {
              # "EXT PhysUnit (0x1B)"
              n723 = Variant To Flattened String(Variant=w2115) -> (1:w2119:i16[])  [unwired: 1 out]
              n724 = call "TypeDescriptor_GetType.vi"("type descriptor"=w2119) -> ("Type"=w2109:u8)  [unwired: 9 in, 1 out]
              n725 = Equal?(x=w2110, y=w2109) -> (x = y?=w2113:bool)
              n726 = Compound Arithmetic op=OR(w2113, invert w2111) -> (w2112:bool)
              n727 = case shown="True" w2112 {
                tunnel: w2118 -> [w2120 w2127]
                tunnel: [w2120 w2126] -> w2117
                tunnel: w2116 -> [_ w2125]
                tunnel: w2109 -> [_ w2124]
                tunnel: w2115 -> [_ w2122]
                tunnel: [_ w2121] -> w2114
                frame False {
                }
                frame True {
                  w2123 = ext 0.0  # EXT
                  n728 = case shown="1..8" w2124 {
                    tunnel: w2127 -> [w2128 _ w2138 w2153 w2168]
                    tunnel: [w2128 w2130 w2140 w2155 w2170] -> w2126
                    tunnel: w2125 -> [_ w2131 w2141 w2156 w2171]
                    tunnel: w2123 -> [_ _ w2136 w2151 w2166]
                    tunnel: w2122 -> [_ w2133 w2135 w2150 w2165]
                    tunnel: [_ TRUE w2134 w2149 w2164] -> w2121
                    frame Default {
                      # "INCOMPATIBLE DATATYPES"
                    }
                    frame 27 {
                      # "EXT PhysUnit (0x1B)"
                      n729 = Variant To Flattened String(Variant=w2133) -> (data string=w2132:string)  [unwired: 1 out]
                      n730 = Flattened String To Variant(6:w2132, 7:w2131) -> (3:w2130:variant)  [unwired: 1 in, 1 out]
                    }
                    frame 1..8 {
                      # "I8, I16, I32, I64, U8, U16, U32, U64"
                      n731 = Variant To Data(type=w2136, Variant=w2135) -> (data=w2137:ext, error out=w2139:errorcluster)  [unwired: 1 in]
                      n732 = case shown="No Error" w2139 {
                        tunnel: w2141 -> [w2147 _]
                        tunnel: [w2146 w2148] -> w2140
                        tunnel: w2138 -> [_ w2148]
                        tunnel: w2137 -> [w2144 _]
                        tunnel: [TRUE _] -> w2134
                        frame No Error {
                          n733 = To Variant(anything=w2144) -> (Variant=w2143:variant)
                          n734 = Variant To Flattened String(Variant=w2143) -> (data string=w2145:string)  [unwired: 1 out]
                          n735 = Flattened String To Variant(6:w2145, 7:w2147) -> (3:w2146:variant)  [unwired: 1 in, 1 out]
                        }
                        frame Error {
                        }
                      }
                    }
                    frame 9..14 {
                      # "SGL, DBL, EXT, CSG, CDB (0x09 .. 0x0E)"
                      n736 = Variant To Data(type=w2151, Variant=w2150) -> (data=w2152:ext, error out=w2154:errorcluster)  [unwired: 1 in]
                      n737 = case shown="No Error" w2154 {
                        tunnel: w2156 -> [w2162 _]
                        tunnel: [w2161 w2163] -> w2155
                        tunnel: w2153 -> [_ w2163]
                        tunnel: w2152 -> [w2159 _]
                        tunnel: [TRUE _] -> w2149
                        frame No Error {
                          n738 = To Variant(anything=w2159) -> (Variant=w2158:variant)
                          n739 = Variant To Flattened String(Variant=w2158) -> (data string=w2160:string)  [unwired: 1 out]
                          n740 = Flattened String To Variant(6:w2160, 7:w2162) -> (3:w2161:variant)  [unwired: 1 in, 1 out]
                        }
                        frame Error {
                        }
                      }
                    }
                    frame 25, 26, 28..30 {
                      # "Physical Units (0x19 .. 0x1E)"
                      n741 = Variant To Data(type=w2166, Variant=w2165) -> (data=w2167:ext, error out=w2169:errorcluster)  [unwired: 1 in]
                      n742 = case shown="No Error" w2169 {
                        tunnel: w2171 -> [w2177 _]
                        tunnel: [w2176 w2178] -> w2170
                        tunnel: w2168 -> [_ w2178]
                        tunnel: w2167 -> [w2174 _]
                        tunnel: [TRUE _] -> w2164
                        frame No Error {
                          n743 = To Variant(anything=w2174) -> (Variant=w2173:variant)
                          n744 = Variant To Flattened String(Variant=w2173) -> (data string=w2175:string)  [unwired: 1 out]
                          n745 = Flattened String To Variant(6:w2175, 7:w2177) -> (3:w2176:variant)  [unwired: 1 in, 1 out]
                        }
                        frame Error {
                        }
                      }
                    }
                  }
                }
              }
            }
            frame 28 {
              # "CSG PhysUnit (0x1C)"
              n746 = Variant To Flattened String(Variant=w2185) -> (1:w2189:i16[])  [unwired: 1 out]
              n747 = call "TypeDescriptor_GetType.vi"("type descriptor"=w2189) -> ("Type"=w2182:u8)  [unwired: 9 in, 1 out]
              n748 = Equal?(x=w2181, y=w2182) -> (x = y?=w2183:bool)
              n749 = Compound Arithmetic op=OR(w2183, invert w2180) -> (w2179:bool)
              n750 = case shown="True" w2179 {
                tunnel: w2188 -> [w2190 w2197]
                tunnel: [w2190 w2196] -> w2187
                tunnel: w2186 -> [_ w2195]
                tunnel: w2185 -> [_ w2193]
                tunnel: [_ w2192] -> w2184
                tunnel: w2182 -> [_ w2191]
                frame False {
                }
                frame True {
                  w2194 = csg 0.0+0.0i  # CSG
                  n751 = case shown="1..8" w2191 {
                    tunnel: w2197 -> [w2198 _ w2208 w2223 w2238]
                    tunnel: [w2198 w2200 w2210 w2225 w2240] -> w2196
                    tunnel: w2195 -> [_ w2201 w2211 w2226 w2241]
                    tunnel: w2194 -> [_ _ w2206 w2221 w2236]
                    tunnel: w2193 -> [_ w2203 w2205 w2220 w2235]
                    tunnel: [_ TRUE w2204 w2219 w2234] -> w2192
                    frame Default {
                      # "INCOMPATIBLE DATATYPES"
                    }
                    frame 28 {
                      # "CSG PhysUnit (0x1C)"
                      n752 = Variant To Flattened String(Variant=w2203) -> (data string=w2202:string)  [unwired: 1 out]
                      n753 = Flattened String To Variant(6:w2202, 7:w2201) -> (3:w2200:variant)  [unwired: 1 in, 1 out]
                    }
                    frame 1..8 {
                      # "I8, I16, I32, I64, U8, U16, U32, U64"
                      n754 = Variant To Data(type=w2206, Variant=w2205) -> (data=w2207:csg, error out=w2209:errorcluster)  [unwired: 1 in]
                      n755 = case shown="No Error" w2209 {
                        tunnel: w2211 -> [w2217 _]
                        tunnel: [w2216 w2218] -> w2210
                        tunnel: w2208 -> [_ w2218]
                        tunnel: w2207 -> [w2214 _]
                        tunnel: [TRUE _] -> w2204
                        frame No Error {
                          n756 = To Variant(anything=w2214) -> (Variant=w2213:variant)
                          n757 = Variant To Flattened String(Variant=w2213) -> (data string=w2215:string)  [unwired: 1 out]
                          n758 = Flattened String To Variant(6:w2215, 7:w2217) -> (3:w2216:variant)  [unwired: 1 in, 1 out]
                        }
                        frame Error {
                        }
                      }
                    }
                    frame 9..14 {
                      # "SGL, DBL, EXT, CSG, CDB (0x09 .. 0x0E)"
                      n759 = Variant To Data(type=w2221, Variant=w2220) -> (data=w2222:csg, error out=w2224:errorcluster)  [unwired: 1 in]
                      n760 = case shown="No Error" w2224 {
                        tunnel: w2226 -> [w2232 _]
                        tunnel: [w2231 w2233] -> w2225
                        tunnel: w2223 -> [_ w2233]
                        tunnel: w2222 -> [w2229 _]
                        tunnel: [TRUE _] -> w2219
                        frame No Error {
                          n761 = To Variant(anything=w2229) -> (Variant=w2228:variant)
                          n762 = Variant To Flattened String(Variant=w2228) -> (data string=w2230:string)  [unwired: 1 out]
                          n763 = Flattened String To Variant(6:w2230, 7:w2232) -> (3:w2231:variant)  [unwired: 1 in, 1 out]
                        }
                        frame Error {
                        }
                      }
                    }
                    frame 25..27, 29, 30 {
                      # "Physical Units (0x19 .. 0x1E)"
                      n764 = Variant To Data(type=w2236, Variant=w2235) -> (data=w2237:csg, error out=w2239:errorcluster)  [unwired: 1 in]
                      n765 = case shown="No Error" w2239 {
                        tunnel: w2241 -> [w2247 _]
                        tunnel: [w2246 w2248] -> w2240
                        tunnel: w2238 -> [_ w2248]
                        tunnel: w2237 -> [w2244 _]
                        tunnel: [TRUE _] -> w2234
                        frame No Error {
                          n766 = To Variant(anything=w2244) -> (Variant=w2243:variant)
                          n767 = Variant To Flattened String(Variant=w2243) -> (data string=w2245:string)  [unwired: 1 out]
                          n768 = Flattened String To Variant(6:w2245, 7:w2247) -> (3:w2246:variant)  [unwired: 1 in, 1 out]
                        }
                        frame Error {
                        }
                      }
                    }
                  }
                }
              }
            }
            frame 29 {
              # "CDB PhysUnit (0x1D)"
              n769 = Variant To Flattened String(Variant=w2255) -> (1:w2259:i16[])  [unwired: 1 out]
              n770 = call "TypeDescriptor_GetType.vi"("type descriptor"=w2259) -> ("Type"=w2250:u8)  [unwired: 9 in, 1 out]
              n771 = Equal?(x=w2251, y=w2250) -> (x = y?=w2253:bool)
              n772 = Compound Arithmetic op=OR(w2253, invert w2249) -> (w2252:bool)
              n773 = case shown="True" w2252 {
                tunnel: w2258 -> [w2260 w2267]
                tunnel: [w2260 w2266] -> w2257
                tunnel: w2256 -> [_ w2265]
                tunnel: w2250 -> [_ w2264]
                tunnel: w2255 -> [_ w2262]
                tunnel: [_ w2261] -> w2254
                frame False {
                }
                frame True {
                  w2263 = cdb 0.0+0.0i  # CDB
                  n774 = case shown="19..1C, 1E" w2264 {
                    tunnel: w2267 -> [w2268 _ w2278 w2293 w2308]
                    tunnel: [w2268 w2269 w2280 w2295 w2310] -> w2266
                    tunnel: w2265 -> [_ w2271 w2281 w2296 w2311]
                    tunnel: w2263 -> [_ _ w2276 w2291 w2306]
                    tunnel: w2262 -> [_ w2273 w2275 w2290 w2305]
                    tunnel: [_ TRUE w2274 w2289 w2304] -> w2261
                    frame Default {
                      # "INCOMPATIBLE DATATYPES"
                    }
                    frame 29 {
                      # "CDB PhysUnit (0x1D)"
                      n775 = Variant To Flattened String(Variant=w2273) -> (data string=w2272:string)  [unwired: 1 out]
                      n776 = Flattened String To Variant(6:w2272, 7:w2271) -> (3:w2269:variant)  [unwired: 1 in, 1 out]
                    }
                    frame 1..8 {
                      # "I8, I16, I32, I64, U8, U16, U32, U64"
                      n777 = Variant To Data(type=w2276, Variant=w2275) -> (data=w2277:cdb, error out=w2279:errorcluster)  [unwired: 1 in]
                      n778 = case shown="No Error" w2279 {
                        tunnel: w2281 -> [w2287 _]
                        tunnel: [w2286 w2288] -> w2280
                        tunnel: w2278 -> [_ w2288]
                        tunnel: w2277 -> [w2284 _]
                        tunnel: [TRUE _] -> w2274
                        frame No Error {
                          n779 = To Variant(anything=w2284) -> (Variant=w2283:variant)
                          n780 = Variant To Flattened String(Variant=w2283) -> (data string=w2285:string)  [unwired: 1 out]
                          n781 = Flattened String To Variant(6:w2285, 7:w2287) -> (3:w2286:variant)  [unwired: 1 in, 1 out]
                        }
                        frame Error {
                        }
                      }
                    }
                    frame 9..14 {
                      # "SGL, DBL, EXT, CSG, CDB (0x09 .. 0x0E)"
                      n782 = Variant To Data(type=w2291, Variant=w2290) -> (data=w2292:cdb, error out=w2294:errorcluster)  [unwired: 1 in]
                      n783 = case shown="No Error" w2294 {
                        tunnel: w2296 -> [w2302 _]
                        tunnel: [w2301 w2303] -> w2295
                        tunnel: w2293 -> [_ w2303]
                        tunnel: w2292 -> [w2299 _]
                        tunnel: [TRUE _] -> w2289
                        frame No Error {
                          n784 = To Variant(anything=w2299) -> (Variant=w2298:variant)
                          n785 = Variant To Flattened String(Variant=w2298) -> (data string=w2300:string)  [unwired: 1 out]
                          n786 = Flattened String To Variant(6:w2300, 7:w2302) -> (3:w2301:variant)  [unwired: 1 in, 1 out]
                        }
                        frame Error {
                        }
                      }
                    }
                    frame 25..28, 30 {
                      # "Physical Units (0x19 .. 0x1E)"
                      n787 = Variant To Data(type=w2306, Variant=w2305) -> (data=w2307:cdb, error out=w2309:errorcluster)  [unwired: 1 in]
                      n788 = case shown="No Error" w2309 {
                        tunnel: w2311 -> [w2317 _]
                        tunnel: [w2316 w2318] -> w2310
                        tunnel: w2308 -> [_ w2318]
                        tunnel: w2307 -> [w2314 _]
                        tunnel: [TRUE _] -> w2304
                        frame No Error {
                          n789 = To Variant(anything=w2314) -> (Variant=w2313:variant)
                          n790 = Variant To Flattened String(Variant=w2313) -> (data string=w2315:string)  [unwired: 1 out]
                          n791 = Flattened String To Variant(6:w2315, 7:w2317) -> (3:w2316:variant)  [unwired: 1 in, 1 out]
                        }
                        frame Error {
                        }
                      }
                    }
                  }
                }
              }
            }
            frame 30 {
              # "CXT PhysUnit (0x1E)"
              n792 = Variant To Flattened String(Variant=w2325) -> (1:w2329:i16[])  [unwired: 1 out]
              n793 = call "TypeDescriptor_GetType.vi"("type descriptor"=w2329) -> ("Type"=w2319:u8)  [unwired: 9 in, 1 out]
              n794 = Equal?(x=w2320, y=w2319) -> (x = y?=w2323:bool)
              n795 = Compound Arithmetic op=OR(w2323, invert w2321) -> (w2322:bool)
              n796 = case shown="True" w2322 {
                tunnel: w2328 -> [w2330 w2337]
                tunnel: [w2330 w2336] -> w2327
                tunnel: w2326 -> [_ w2335]
                tunnel: w2319 -> [_ w2334]
                tunnel: w2325 -> [_ w2332]
                tunnel: [_ w2331] -> w2324
                frame False {
                }
                frame True {
                  w2333 = cxt 0.0+0.0i  # CXT
                  n797 = case shown="1..8" w2334 {
                    tunnel: w2337 -> [w2338 _ w2348 w2363 w2378]
                    tunnel: [w2338 w2340 w2350 w2365 w2380] -> w2336
                    tunnel: w2335 -> [_ w2341 w2351 w2366 w2381]
                    tunnel: w2333 -> [_ _ w2346 w2361 w2376]
                    tunnel: w2332 -> [_ w2343 w2345 w2360 w2375]
                    tunnel: [_ TRUE w2344 w2359 w2374] -> w2331
                    frame Default {
                      # "INCOMPATIBLE DATATYPES"
                    }
                    frame 30 {
                      # "CXT PhysUnit (0x1E)"
                      n798 = Variant To Flattened String(Variant=w2343) -> (data string=w2342:string)  [unwired: 1 out]
                      n799 = Flattened String To Variant(6:w2342, 7:w2341) -> (3:w2340:variant)  [unwired: 1 in, 1 out]
                    }
                    frame 1..8 {
                      # "I8, I16, I32, I64, U8, U16, U32, U64"
                      n800 = Variant To Data(type=w2346, Variant=w2345) -> (data=w2347:cxt, error out=w2349:errorcluster)  [unwired: 1 in]
                      n801 = case shown="No Error" w2349 {
                        tunnel: w2351 -> [w2357 _]
                        tunnel: [w2356 w2358] -> w2350
                        tunnel: w2348 -> [_ w2358]
                        tunnel: w2347 -> [w2354 _]
                        tunnel: [TRUE _] -> w2344
                        frame No Error {
                          n802 = To Variant(anything=w2354) -> (Variant=w2353:variant)
                          n803 = Variant To Flattened String(Variant=w2353) -> (data string=w2355:string)  [unwired: 1 out]
                          n804 = Flattened String To Variant(6:w2355, 7:w2357) -> (3:w2356:variant)  [unwired: 1 in, 1 out]
                        }
                        frame Error {
                        }
                      }
                    }
                    frame 9..14 {
                      # "SGL, DBL, EXT, CSG, CDB (0x09 .. 0x0E)"
                      n805 = Variant To Data(type=w2361, Variant=w2360) -> (data=w2362:cxt, error out=w2364:errorcluster)  [unwired: 1 in]
                      n806 = case shown="No Error" w2364 {
                        tunnel: w2366 -> [w2372 _]
                        tunnel: [w2371 w2373] -> w2365
                        tunnel: w2363 -> [_ w2373]
                        tunnel: w2362 -> [w2369 _]
                        tunnel: [TRUE _] -> w2359
                        frame No Error {
                          n807 = To Variant(anything=w2369) -> (Variant=w2368:variant)
                          n808 = Variant To Flattened String(Variant=w2368) -> (data string=w2370:string)  [unwired: 1 out]
                          n809 = Flattened String To Variant(6:w2370, 7:w2372) -> (3:w2371:variant)  [unwired: 1 in, 1 out]
                        }
                        frame Error {
                        }
                      }
                    }
                    frame 25..29 {
                      # "Physical Units (0x19 .. 0x1E)"
                      n810 = Variant To Data(type=w2376, Variant=w2375) -> (data=w2377:cxt, error out=w2379:errorcluster)  [unwired: 1 in]
                      n811 = case shown="No Error" w2379 {
                        tunnel: w2381 -> [w2387 _]
                        tunnel: [w2386 w2388] -> w2380
                        tunnel: w2378 -> [_ w2388]
                        tunnel: w2377 -> [w2384 _]
                        tunnel: [TRUE _] -> w2374
                        frame No Error {
                          n812 = To Variant(anything=w2384) -> (Variant=w2383:variant)
                          n813 = Variant To Flattened String(Variant=w2383) -> (data string=w2385:string)  [unwired: 1 out]
                          n814 = Flattened String To Variant(6:w2385, 7:w2387) -> (3:w2386:variant)  [unwired: 1 in, 1 out]
                        }
                        frame Error {
                        }
                      }
                    }
                  }
                }
              }
            }
            frame 33 {
              # "Boolean (0x21)"
              n815 = Variant To Flattened String(Variant=w2395) -> (1:w2399:i16[])  [unwired: 1 out]
              n816 = call "TypeDescriptor_GetType.vi"("type descriptor"=w2399) -> ("Type"=w2389:u8)  [unwired: 9 in, 1 out]
              n817 = Equal?(x=w2390, y=w2389) -> (x = y?=w2393:bool)
              n818 = Compound Arithmetic op=OR(w2393, invert w2391) -> (w2392:bool)
              n819 = case shown="True" w2392 {
                tunnel: w2398 -> [w2400 w2406]
                tunnel: [w2400 w2405] -> w2397
                tunnel: w2396 -> [_ w2404]
                tunnel: w2389 -> [_ w2403]
                tunnel: w2395 -> [_ w2402]
                tunnel: [_ w2401] -> w2394
                frame False {
                }
                frame True {
                  n820 = case shown="30" w2403 {
                    tunnel: w2406 -> [w2407 _ _ w2427]
                    tunnel: [w2407 w2417 w2422 w2429] -> w2405
                    tunnel: w2404 -> [_ w2418 w2423 w2431]
                    tunnel: w2402 -> [_ w2416 w2420 w2425]
                    tunnel: [_ TRUE TRUE w2424] -> w2401
                    frame Default {
                      # "INCOMPATIBLE DATATYPES"
                    }
                    frame 1..8 {
                      # "I8, I16, I32, I64, U8, U16, U32"
                      n821 = Variant To Flattened String(Variant=w2416) -> (data string=w2415:string)  [unwired: 1 out]
                      n822 = String To Byte Array(string=w2415) -> (unsigned byte array=w2413:u8[])
                      n823 = Not Equal To 0?(x=w2413) -> (x != 0?=w2414:bool[])
                      n824 = Or Array Elements(Boolean array=w2414) -> (logical OR=w2412:bool)
                      n825 = Select(t="\u0001" ("string"), s=w2412, f="\u0000" ("string")) -> (s? t:f=w2409:string)
                      n826 = Flattened String To Variant(6:w2409, 7:w2418) -> (3:w2417:variant)  [unwired: 1 in, 1 out]
                    }
                    frame 33 {
                      # "Boolean (0x21)"
                      n827 = Variant To Flattened String(Variant=w2420) -> (data string=w2421:string)  [unwired: 1 out]
                      n828 = Flattened String To Variant(6:w2421, 7:w2423) -> (3:w2422:variant)  [unwired: 1 in, 1 out]
                    }
                    frame 48 {
                      # "STRING (0x30)"
                      n829 = Variant To Data(type="", Variant=w2425) -> (data=w2426:string, error out=w2428:errorcluster)  [unwired: 1 in]
                      n830 = case shown="No Error" w2428 {
                        tunnel: w2431 -> [w2433 _]
                        tunnel: [w2434 w2445] -> w2429
                        tunnel: w2427 -> [w2435 w2445]
                        tunnel: w2426 -> [w2437 _]
                        tunnel: [TRUE _] -> w2424
                        frame No Error {
                          n831 = To Lower Case(string=w2437) -> (all lower case string=w2436:string)
                          n832 = case shown="\"true\"" w2436 {
                            tunnel: w2435 -> [w2438 _ _]
                            tunnel: [w2438 w2439 w2442] -> w2434
                            tunnel: w2433 -> [_ w2441 w2444]
                            frame Default {
                            }
                            frame "true" {
                              n833 = Flattened String To Variant(6:"\u0001" ("data string"), 7:w2441) -> (3:w2439:variant)  [unwired: 1 in, 1 out]
                            }
                            frame "false" {
                              n834 = Flattened String To Variant(6:"\u0000" ("data string"), 7:w2444) -> (3:w2442:variant)  [unwired: 1 in, 1 out]
                            }
                          }
                        }
                        frame Error {
                        }
                      }
                    }
                  }
                }
              }
            }
            frame 48 {
              # "STRING (0x30)"
              n835 = Variant To Flattened String(Variant=w2454) -> (data string=w2453:string, 1:w2452:i16[])
              n836 = call "TypeDescriptor_GetType.vi"("type descriptor"=w2452) -> ("Type"=w2447:u8, "type descriptor dup"=w2455:i16[])  [unwired: 9 in]
              n837 = Equal?(x=w2448, y=w2447) -> (x = y?=w2450:bool)
              n838 = Compound Arithmetic op=OR(w2450, invert w2446) -> (w2449:bool)
              n839 = case shown="True" w2449 {
                tunnel: w2458 -> [w2459 w2467]
                tunnel: [w2459 w2466] -> w2457
                tunnel: w2456 -> [_ w2465]
                tunnel: w2447 -> [_ w2464]
                tunnel: w2455 -> [_ w2463]
                tunnel: w2454 -> [_ w2462]
                tunnel: w2453 -> [_ w2461]
                tunnel: [_ w2460] -> w2451
                frame False {
                }
                frame True {
                  n840 = case shown="15" w2464 {
                    tunnel: w2461 -> [_ w2472 _ _ _ _ _ _ _ _ _ _ _ _ _ _ _ _ w2743]
                    tunnel: w2467 -> [w2468 _ w2476 w2492 w2509 w2525 w2541 w2557 w2573 w2589 w2605 w2621 w2637 w2654 w2671 w2688 w2705 w2722 _]
                    tunnel: [w2468 w2471 w2478 w2494 w2511 w2527 w2543 w2559 w2575 w2591 w2607 w2623 w2639 w2656 w2673 w2690 w2707 w2724 w2744] -> w2466
                    tunnel: w2465 -> [_ w2470 w2480 w2496 w2512 w2528 w2544 w2560 w2576 w2592 w2608 w2624 w2640 w2657 w2674 w2691 w2708 w2725 w2745]
                    tunnel: w2463 -> [_ _ _ _ _ _ _ _ _ _ _ _ _ _ _ _ _ _ w2739]
                    tunnel: w2462 -> [_ _ w2474 w2490 w2506 w2522 w2538 w2554 w2570 w2586 w2602 w2618 w2634 w2651 w2668 w2685 w2702 w2719 _]
                    tunnel: [_ TRUE w2473 w2489 w2505 w2521 w2537 w2553 w2569 w2585 w2601 w2617 w2633 w2650 w2667 w2684 w2701 w2718 TRUE] -> w2460
                    frame Default {
                      # "INCOMPATIBLE DATATYPES"
                    }
                    frame 48 {
                      # "STRING (0x30)"
                      n841 = Flattened String To Variant(6:w2472, 7:w2470) -> (3:w2471:variant)  [unwired: 1 in, 1 out]
                    }
                    frame 50 {
                      # "PATH (0x32)"
                      n842 = Variant To Data(type=path "", Variant=w2474) -> (data=w2475:path, error out=w2477:errorcluster)  [unwired: 1 in]
                      n843 = case shown="No Error" w2477 {
                        tunnel: w2480 -> [w2487 _]
                        tunnel: [w2486 w2488] -> w2478
                        tunnel: w2476 -> [_ w2488]
                        tunnel: w2475 -> [w2483 _]
                        tunnel: [TRUE _] -> w2473
                        frame No Error {
                          n844 = Path To String(path=w2483) -> (string=w2485:string)
                          n845 = To Variant(anything=w2485) -> (Variant=w2484:variant)
                          n846 = Variant To Flattened String(Variant=w2484) -> (data string=w2482:string)  [unwired: 1 out]
                          n847 = Flattened String To Variant(6:w2482, 7:w2487) -> (3:w2486:variant)  [unwired: 1 in, 1 out]
                        }
                        frame Error {
                        }
                      }
                    }
                    frame 33 {
                      # "BOOLEAN (0x21)"
                      n848 = Variant To Data(type=FALSE, Variant=w2490) -> (data=w2491:bool, error out=w2493:errorcluster)  [unwired: 1 in]
                      n849 = case shown="No Error" w2493 {
                        tunnel: w2496 -> [w2503 _]
                        tunnel: [w2502 w2504] -> w2494
                        tunnel: w2492 -> [_ w2504]
                        tunnel: w2491 -> [w2499 _]
                        tunnel: [TRUE _] -> w2489
                        frame No Error {
                          n850 = Format Into String(w2499) -> (resulting string=w2498:string)  [unwired: 3 in, 1 out]
                          n851 = To Variant(anything=w2498) -> (Variant=w2501:variant)
                          n852 = Variant To Flattened String(Variant=w2501) -> (data string=w2500:string)  [unwired: 1 out]
                          n853 = Flattened String To Variant(6:w2500, 7:w2503) -> (3:w2502:variant)  [unwired: 1 in, 1 out]
                        }
                        frame Error {
                        }
                      }
                    }
                    frame 1 {
                      # "I8 (0x01)"
                      n854 = Variant To Data(type=i8 0, Variant=w2506) -> (data=w2508:i8, error out=w2510:errorcluster)  [unwired: 1 in]
                      n855 = case shown="No Error" w2510 {
                        tunnel: w2512 -> [w2519 _]
                        tunnel: [w2518 w2520] -> w2511
                        tunnel: w2509 -> [_ w2520]
                        tunnel: w2508 -> [w2515 _]
                        tunnel: [TRUE _] -> w2505
                        frame No Error {
                          n856 = Format Into String(w2515) -> (resulting string=w2514:string)  [unwired: 3 in, 1 out]
                          n857 = To Variant(anything=w2514) -> (Variant=w2517:variant)
                          n858 = Variant To Flattened String(Variant=w2517) -> (data string=w2516:string)  [unwired: 1 out]
                          n859 = Flattened String To Variant(6:w2516, 7:w2519) -> (3:w2518:variant)  [unwired: 1 in, 1 out]
                        }
                        frame Error {
                        }
                      }
                    }
                    frame 2 {
                      # "I16 (0x02)"
                      n860 = Variant To Data(type=i16 0, Variant=w2522) -> (data=w2524:i16, error out=w2526:errorcluster)  [unwired: 1 in]
                      n861 = case shown="No Error" w2526 {
                        tunnel: w2528 -> [w2535 _]
                        tunnel: [w2534 w2536] -> w2527
                        tunnel: w2525 -> [_ w2536]
                        tunnel: w2524 -> [w2531 _]
                        tunnel: [TRUE _] -> w2521
                        frame No Error {
                          n862 = Format Into String(w2531) -> (resulting string=w2530:string)  [unwired: 3 in, 1 out]
                          n863 = To Variant(anything=w2530) -> (Variant=w2533:variant)
                          n864 = Variant To Flattened String(Variant=w2533) -> (data string=w2532:string)  [unwired: 1 out]
                          n865 = Flattened String To Variant(6:w2532, 7:w2535) -> (3:w2534:variant)  [unwired: 1 in, 1 out]
                        }
                        frame Error {
                        }
                      }
                    }
                    frame 3 {
                      # "I32 (0x03)"
                      n866 = Variant To Data(type=0, Variant=w2538) -> (data=w2540:i32, error out=w2542:errorcluster)  [unwired: 1 in]
                      n867 = case shown="No Error" w2542 {
                        tunnel: w2544 -> [w2551 _]
                        tunnel: [w2550 w2552] -> w2543
                        tunnel: w2541 -> [_ w2552]
                        tunnel: w2540 -> [w2547 _]
                        tunnel: [TRUE _] -> w2537
                        frame No Error {
                          n868 = Format Into String(w2547) -> (resulting string=w2546:string)  [unwired: 3 in, 1 out]
                          n869 = To Variant(anything=w2546) -> (Variant=w2549:variant)
                          n870 = Variant To Flattened String(Variant=w2549) -> (data string=w2548:string)  [unwired: 1 out]
                          n871 = Flattened String To Variant(6:w2548, 7:w2551) -> (3:w2550:variant)  [unwired: 1 in, 1 out]
                        }
                        frame Error {
                        }
                      }
                    }
                    frame 4 {
                      # "I64 (0x04)"
                      n872 = Variant To Data(type=i64 0, Variant=w2554) -> (data=w2556:i64, error out=w2558:errorcluster)  [unwired: 1 in]
                      n873 = case shown="No Error" w2558 {
                        tunnel: w2560 -> [w2567 _]
                        tunnel: [w2566 w2568] -> w2559
                        tunnel: w2557 -> [_ w2568]
                        tunnel: w2556 -> [w2563 _]
                        tunnel: [TRUE _] -> w2553
                        frame No Error {
                          n874 = Format Into String(w2563) -> (resulting string=w2562:string)  [unwired: 3 in, 1 out]
                          n875 = To Variant(anything=w2562) -> (Variant=w2565:variant)
                          n876 = Variant To Flattened String(Variant=w2565) -> (data string=w2564:string)  [unwired: 1 out]
                          n877 = Flattened String To Variant(6:w2564, 7:w2567) -> (3:w2566:variant)  [unwired: 1 in, 1 out]
                        }
                        frame Error {
                        }
                      }
                    }
                    frame 5 {
                      # "U8 (0x05)"
                      n878 = Variant To Data(type=u8 0, Variant=w2570) -> (data=w2572:u8, error out=w2574:errorcluster)  [unwired: 1 in]
                      n879 = case shown="No Error" w2574 {
                        tunnel: w2576 -> [w2583 _]
                        tunnel: [w2582 w2584] -> w2575
                        tunnel: w2573 -> [_ w2584]
                        tunnel: w2572 -> [w2579 _]
                        tunnel: [TRUE _] -> w2569
                        frame No Error {
                          n880 = Format Into String(w2579) -> (resulting string=w2578:string)  [unwired: 3 in, 1 out]
                          n881 = To Variant(anything=w2578) -> (Variant=w2581:variant)
                          n882 = Variant To Flattened String(Variant=w2581) -> (data string=w2580:string)  [unwired: 1 out]
                          n883 = Flattened String To Variant(6:w2580, 7:w2583) -> (3:w2582:variant)  [unwired: 1 in, 1 out]
                        }
                        frame Error {
                        }
                      }
                    }
                    frame 6 {
                      # "U16 (0x06)"
                      n884 = Variant To Data(type=u16 0, Variant=w2586) -> (data=w2588:u16, error out=w2590:errorcluster)  [unwired: 1 in]
                      n885 = case shown="No Error" w2590 {
                        tunnel: w2592 -> [w2599 _]
                        tunnel: [w2598 w2600] -> w2591
                        tunnel: w2589 -> [_ w2600]
                        tunnel: w2588 -> [w2595 _]
                        tunnel: [TRUE _] -> w2585
                        frame No Error {
                          n886 = Format Into String(w2595) -> (resulting string=w2594:string)  [unwired: 3 in, 1 out]
                          n887 = To Variant(anything=w2594) -> (Variant=w2597:variant)
                          n888 = Variant To Flattened String(Variant=w2597) -> (data string=w2596:string)  [unwired: 1 out]
                          n889 = Flattened String To Variant(6:w2596, 7:w2599) -> (3:w2598:variant)  [unwired: 1 in, 1 out]
                        }
                        frame Error {
                        }
                      }
                    }
                    frame 7 {
                      # "U32 (0x07)"
                      n890 = Variant To Data(type=u32 0, Variant=w2602) -> (data=w2604:u32, error out=w2606:errorcluster)  [unwired: 1 in]
                      n891 = case shown="No Error" w2606 {
                        tunnel: w2608 -> [w2615 _]
                        tunnel: [w2614 w2616] -> w2607
                        tunnel: w2605 -> [_ w2616]
                        tunnel: w2604 -> [w2611 _]
                        tunnel: [TRUE _] -> w2601
                        frame No Error {
                          n892 = Format Into String(w2611) -> (resulting string=w2610:string)  [unwired: 3 in, 1 out]
                          n893 = To Variant(anything=w2610) -> (Variant=w2613:variant)
                          n894 = Variant To Flattened String(Variant=w2613) -> (data string=w2612:string)  [unwired: 1 out]
                          n895 = Flattened String To Variant(6:w2612, 7:w2615) -> (3:w2614:variant)  [unwired: 1 in, 1 out]
                        }
                        frame Error {
                        }
                      }
                    }
                    frame 8 {
                      # "U64 (0x08)"
                      n896 = Variant To Data(type=u64 0, Variant=w2618) -> (data=w2620:u64, error out=w2622:errorcluster)  [unwired: 1 in]
                      n897 = case shown="No Error" w2622 {
                        tunnel: w2624 -> [w2631 _]
                        tunnel: [w2630 w2632] -> w2623
                        tunnel: w2621 -> [_ w2632]
                        tunnel: w2620 -> [w2627 _]
                        tunnel: [TRUE _] -> w2617
                        frame No Error {
                          n898 = Format Into String(w2627) -> (resulting string=w2626:string)  [unwired: 3 in, 1 out]
                          n899 = To Variant(anything=w2626) -> (Variant=w2629:variant)
                          n900 = Variant To Flattened String(Variant=w2629) -> (data string=w2628:string)  [unwired: 1 out]
                          n901 = Flattened String To Variant(6:w2628, 7:w2631) -> (3:w2630:variant)  [unwired: 1 in, 1 out]
                        }
                        frame Error {
                        }
                      }
                    }
                    frame 9 {
                      # "SGL (0x09)"
                      n902 = Variant To Data(type=sgl 0.0, Variant=w2634) -> (data=w2636:sgl, error out=w2638:errorcluster)  [unwired: 1 in]
                      n903 = case shown="No Error" w2638 {
                        tunnel: w2640 -> [w2648 _]
                        tunnel: [w2647 w2649] -> w2639
                        tunnel: w2637 -> [_ w2649]
                        tunnel: w2636 -> [w2642 _]
                        tunnel: [TRUE _] -> w2633
                        frame No Error {
                          n904 = Format Into String(format string="%#.6g", w2642) -> (resulting string=w2644:string)  [unwired: 2 in, 1 out]
                          n905 = To Variant(anything=w2644) -> (Variant=w2646:variant)
                          n906 = Variant To Flattened String(Variant=w2646) -> (data string=w2645:string)  [unwired: 1 out]
                          n907 = Flattened String To Variant(6:w2645, 7:w2648) -> (3:w2647:variant)  [unwired: 1 in, 1 out]
                        }
                        frame Error {
                        }
                      }
                    }
                    frame 10 {
                      # "DBL (0x0A)"
                      n908 = Variant To Data(type=0.0, Variant=w2651) -> (data=w2653:dbl, error out=w2655:errorcluster)  [unwired: 1 in]
                      n909 = case shown="No Error" w2655 {
                        tunnel: w2657 -> [w2665 _]
                        tunnel: [w2664 w2666] -> w2656
                        tunnel: w2654 -> [_ w2666]
                        tunnel: w2653 -> [w2659 _]
                        tunnel: [TRUE _] -> w2650
                        frame No Error {
                          n910 = Format Into String(format string="%#.15g", w2659) -> (resulting string=w2661:string)  [unwired: 2 in, 1 out]
                          n911 = To Variant(anything=w2661) -> (Variant=w2663:variant)
                          n912 = Variant To Flattened String(Variant=w2663) -> (data string=w2662:string)  [unwired: 1 out]
                          n913 = Flattened String To Variant(6:w2662, 7:w2665) -> (3:w2664:variant)  [unwired: 1 in, 1 out]
                        }
                        frame Error {
                        }
                      }
                    }
                    frame 11 {
                      # "EXT (0x0B)"
                      n914 = Variant To Data(type=ext 0.0, Variant=w2668) -> (data=w2670:ext, error out=w2672:errorcluster)  [unwired: 1 in]
                      n915 = case shown="No Error" w2672 {
                        tunnel: w2674 -> [w2682 _]
                        tunnel: [w2681 w2683] -> w2673
                        tunnel: w2671 -> [_ w2683]
                        tunnel: w2670 -> [w2676 _]
                        tunnel: [TRUE _] -> w2667
                        frame No Error {
                          n916 = Format Into String(format string="%#.20g", w2676) -> (resulting string=w2678:string)  [unwired: 2 in, 1 out]
                          n917 = To Variant(anything=w2678) -> (Variant=w2680:variant)
                          n918 = Variant To Flattened String(Variant=w2680) -> (data string=w2679:string)  [unwired: 1 out]
                          n919 = Flattened String To Variant(6:w2679, 7:w2682) -> (3:w2681:variant)  [unwired: 1 in, 1 out]
                        }
                        frame Error {
                        }
                      }
                    }
                    frame 12 {
                      # "CSG (0x0C)"
                      n920 = Variant To Data(type=csg 0.0+0.0i, Variant=w2685) -> (data=w2687:csg, error out=w2689:errorcluster)  [unwired: 1 in]
                      n921 = case shown="No Error" w2689 {
                        tunnel: w2691 -> [w2699 _]
                        tunnel: [w2698 w2700] -> w2690
                        tunnel: w2688 -> [_ w2700]
                        tunnel: w2687 -> [w2692 _]
                        tunnel: [TRUE _] -> w2684
                        frame No Error {
                          n922 = Format Into String(format string="%#.20f", w2692) -> (resulting string=w2695:string)  [unwired: 2 in, 1 out]
                          n923 = To Variant(anything=w2695) -> (Variant=w2697:variant)
                          n924 = Variant To Flattened String(Variant=w2697) -> (data string=w2696:string)  [unwired: 1 out]
                          n925 = Flattened String To Variant(6:w2696, 7:w2699) -> (3:w2698:variant)  [unwired: 1 in, 1 out]
                        }
                        frame Error {
                        }
                      }
                    }
                    frame 13 {
                      # "CDB (0x0D)"
                      n926 = Variant To Data(type=cdb 0.0+0.0i, Variant=w2702) -> (data=w2704:cdb, error out=w2706:errorcluster)  [unwired: 1 in]
                      n927 = case shown="No Error" w2706 {
                        tunnel: w2708 -> [w2716 _]
                        tunnel: [w2715 w2717] -> w2707
                        tunnel: w2705 -> [_ w2717]
                        tunnel: w2704 -> [w2712 _]
                        tunnel: [TRUE _] -> w2701
                        frame No Error {
                          n928 = Format Into String(format string="%#.20f", w2712) -> (resulting string=w2711:string)  [unwired: 2 in, 1 out]
                          n929 = To Variant(anything=w2711) -> (Variant=w2714:variant)
                          n930 = Variant To Flattened String(Variant=w2714) -> (data string=w2713:string)  [unwired: 1 out]
                          n931 = Flattened String To Variant(6:w2713, 7:w2716) -> (3:w2715:variant)  [unwired: 1 in, 1 out]
                        }
                        frame Error {
                        }
                      }
                    }
                    frame 14 {
                      # "CXT (0x0E)"
                      n932 = Variant To Data(type=cxt 0.0+0.0i, Variant=w2719) -> (data=w2721:cxt, error out=w2723:errorcluster)  [unwired: 1 in]
                      n933 = case shown="No Error" w2723 {
                        tunnel: w2725 -> [w2733 _]
                        tunnel: [w2732 w2734] -> w2724
                        tunnel: w2722 -> [_ w2734]
                        tunnel: w2721 -> [w2729 _]
                        tunnel: [TRUE _] -> w2718
                        frame No Error {
                          n934 = Format Into String(format string="%#.20f", w2729) -> (resulting string=w2728:string)  [unwired: 2 in, 1 out]
                          n935 = To Variant(anything=w2728) -> (Variant=w2731:variant)
                          n936 = Variant To Flattened String(Variant=w2731) -> (data string=w2730:string)  [unwired: 1 out]
                          n937 = Flattened String To Variant(6:w2730, 7:w2733) -> (3:w2732:variant)  [unwired: 1 in, 1 out]
                        }
                        frame Error {
                        }
                      }
                    }
                    frame 21 {
                      # "EnumU8 (0x15)"
                      n938 = String To Byte Array(string=w2743) -> (unsigned byte array=w2740:u8[])
                      n939 = Index Array(array=w2740) -> (element=w2736:u8)  [unwired: 1 in]
                      n940 = call "TypeDescriptor_ListElementNames.vi"("type descriptor"=w2739) -> ("element names"=w2738:string[])  [unwired: 7 in, 3 out]
                      n941 = Index Array(array=w2738, index=w2736) -> (element=w2737:string)
                      n942 = To Variant(anything=w2737) -> (Variant=w2742:variant)
                      n943 = Variant To Flattened String(Variant=w2742) -> (data string=w2741:string)  [unwired: 1 out]
                      n944 = Flattened String To Variant(6:w2741, 7:w2745) -> (3:w2744:variant)  [unwired: 1 in, 1 out]
                    }
                  }
                }
              }
            }
            frame 50 {
              # "PATH (0x32)"
              n945 = Variant To Flattened String(Variant=w2758) -> (data string=w2757:string, 1:w2756:i16[])
              n946 = call "TypeDescriptor_GetType.vi"("type descriptor"=w2756) -> ("Type"=w2748:u8, "type descriptor dup"=w2752:i16[])  [unwired: 9 in]
              n947 = Equal?(x=w2749, y=w2748) -> (x = y?=w2750:bool)
              n948 = Compound Arithmetic op=OR(w2750, invert w2747) -> (w2746:bool)
              n949 = case shown="True" w2746 {
                tunnel: w2757 -> [_ w2766]
                tunnel: w2755 -> [w2759 w2765]
                tunnel: [w2759 w2764] -> w2754
                tunnel: w2753 -> [_ w2763]
                tunnel: w2752 -> [_ w2762]
                tunnel: [_ w2761] -> w2751
                tunnel: w2748 -> [_ w2760]
                frame False {
                }
                frame True {
                  n950 = case shown="30" w2760 {
                    tunnel: w2766 -> [_ w2771 w2780]
                    tunnel: w2765 -> [w2767 _ w2774]
                    tunnel: [w2767 w2770 w2776] -> w2764
                    tunnel: w2763 -> [_ w2769 w2782]
                    tunnel: w2762 -> [_ _ w2781]
                    tunnel: [_ TRUE w2772] -> w2761
                    frame Default {
                      # "INCOMPATIBLE DATATYPES"
                    }
                    frame 50 {
                      # "PATH (0x32)"
                      n951 = Flattened String To Variant(6:w2771, 7:w2769) -> (3:w2770:variant)  [unwired: 1 in, 1 out]
                    }
                    frame 48 {
                      # "STRING (0x30)"
                      n952 = Flattened String To Variant(6:w2780, 7:w2781) -> (0:w2777:errorcluster, 3:w2779:variant)  [unwired: 1 in]
                      n953 = Variant To Data(error in=w2777, type="", Variant=w2779) -> (data=w2773:string, error out=w2775:errorcluster)
                      n954 = case shown="No Error" w2775 {
                        tunnel: w2782 -> [w2789 _]
                        tunnel: [w2788 w2790] -> w2776
                        tunnel: w2774 -> [_ w2790]
                        tunnel: w2773 -> [w2785 _]
                        tunnel: [TRUE _] -> w2772
                        frame No Error {
                          n955 = String To Path(string=w2785) -> (path=w2787:path)
                          n956 = To Variant(anything=w2787) -> (Variant=w2786:variant)
                          n957 = Variant To Flattened String(Variant=w2786) -> (data string=w2784:string)  [unwired: 1 out]
                          n958 = Flattened String To Variant(6:w2784, 7:w2789) -> (3:w2788:variant)  [unwired: 1 in, 1 out]
                        }
                        frame Error {
                        }
                      }
                    }
                  }
                }
              }
            }
            frame 64 {
              # "ARRAY (0x40)"
              n959 = Variant To Flattened String(Variant=w2791) -> (data string=w2815:string, 1:w2798:i16[])
              n960 = call <vilib>:"TD_Get Array Information.vi"("Type descriptor"=w2805) -> ("Contained TD Offset"=w2808:i32)  [unwired: 8 in, 2 out]
              n961 = call <vilib>:"TD_Get Array Information.vi"("Type descriptor"=w2798) -> ("Contained TD Offset"=w2799:i32)  [unwired: 8 in, 2 out]
              n962 = call "TypeDescriptor_GetType.vi"("type descriptor"=w2798) -> ("Type"=w2809:u8, "type descriptor dup"=w2804:i16[])  [unwired: 9 in]
              n963 = call <vilib>:"Get Type Code from I16 Array And Pos.vi"("Pos in Type Descriptor (0)"=w2808, "Type descriptor"=w2805) -> ("Size (Words)"=w2807:i32)  [unwired: 7 in, 2 out]
              n964 = Equal?(x=w2810, y=w2809) -> (x = y?=w2811:bool)
              n965 = call <vilib>:"Get Type Code from I16 Array And Pos.vi"("Pos in Type Descriptor (0)"=w2799, "Type descriptor"=w2798) -> ("Size (Words)"=w2800:i32)  [unwired: 7 in, 2 out]
              n966 = Array Subset(array=w2805, index=w2808, length=w2807) -> (w2806:i16[])
              n967 = Array Subset(array=w2798, index=w2799, length=w2800) -> (w2801:i16[])
              n968 = call <vilib>:"Get Type Code from I16 Array And Pos.vi"("Type descriptor"=w2806) -> ("Type Enum"=w2797:T1)  [unwired: 8 in, 2 out]
              n969 = call <vilib>:"Get Type Code from I16 Array And Pos.vi"("Type descriptor"=w2801) -> ("Type Enum"=w2796:T1)  [unwired: 8 in, 2 out]
              n970 = Equal?(x=w2797, y=w2796) -> (x = y?=w2794:bool)
              n971 = call <vilib>:"TD_Compare Types.vi"("Type descriptor 2"=w2804, "Type descriptor"=w2805) -> ("Types Wireable?"=w2803:bool)  [unwired: 9 in]
              n972 = Compound Arithmetic op=OR(w2811, invert w2793) -> (w2795:bool)
              n973 = Compound Arithmetic op=OR(w2794, invert w2793) -> (w2792:bool)
              n974 = Compound Arithmetic op=AND(w2803, w2795, w2792) -> (w2802:bool)
              n975 = case shown="False" w2802 {
                tunnel: w2815 -> [w2822 _]
                tunnel: w2814 -> [w2820 w2825]
                tunnel: [w2818 w2828] -> w2813
                tunnel: w2805 -> [w2821 _]
                tunnel: w2804 -> [_ _]
                tunnel: [w2816 w2827] -> w2812
                tunnel: w2809 -> [_ _]
                tunnel: w2791 -> [_ w2826]
                frame True {
                  n976 = Flattened String To Variant(6:w2822, 7:w2821) -> (0:w2817:errorcluster, 3:w2819:variant)  [unwired: 1 in]
                  n977 = Select(t=w2820, s=w2817, f=w2819) -> (s? t:f=w2818:variant)
                  n978 = Not(x=w2817) -> (.not. x?=w2816:bool)
                }
                frame False {
                  # "Type Casting id subtypes\nCheck if wireable"
                  n979 = Variant To Data(type=w2825, Variant=w2826) -> (data=w2824:variant, error out=w2823:errorcluster)  [unwired: 1 in]
                  n980 = Select(t=w2825, s=w2823, f=w2824) -> (s? t:f=w2828:variant)
                  n981 = Not(x=w2823) -> (.not. x?=w2827:bool)
                }
              }
            }
            frame 80 {
              # "CLUSTER (0x50)"
              n982 = call "Variant_ExtractClusterElements.vi"("Cluster"=w2839) -> ("Elements"=w2830:variant[])  [unwired: 8 in, 2 out]
              n983 = call "Variant_ExtractClusterElements.vi"("Cluster"=w2840) -> ("name"=w2837:string, "Elements"=w2838:variant[])  [unwired: 8 in, 1 out]
              n984 = for {
                tunnel: w2838 -> [w2849] mode=indexing
                tunnel: [w2848] -> w2829 mode=indexing
                tunnel: [w2847] -> w2835 mode=indexing
                n985 = call "Variant_GetName.vi"("Variant"=w2849) -> ("Name"=w2848:string, "Variant dup"=w2847:variant)  [unwired: 8 in, 1 out]
              }
              n986 = for {
                tunnel: w2836 -> [w2846]
                tunnel: w2835 -> [w2845] mode=indexing
                tunnel: [w2844] -> w2834 mode=indexing
                tunnel: [w2843] -> w2833 mode=indexing
                tunnel: w2830 -> [w2842]
                tunnel: w2829 -> [w2841]
                n987 = call "KVP Parser.vi"("Values"=w2842, "Keys"=w2841, "Strict type matching? (F)"=w2846, "Default Value"=w2845) -> ("any found?"=w2843:bool, "Value"=w2844:variant)  [unwired: 4 in, 2 out]
              }
              n988 = Or Array Elements(Boolean array=w2833) -> (logical OR=w2832:bool)
              n989 = call "Variant_BuildClusterFromElementArray.vi"("name"=w2837, "Elements"=w2834) -> ("Cluster"=w2831:variant)  [unwired: 9 in]
            }
            frame 112 {
              # "REFNUMS (0x70)"
              n990 = Variant To Flattened String(Variant=w2864) -> (data string=w2863:string, 1:w2862:i16[])
              n991 = call "TypeDescriptor_GetType.vi"("type descriptor"=w2862) -> ("Type"=w2854:u8, "type descriptor dup"=w2859:i16[])  [unwired: 9 in]
              n992 = Equal?(x=w2850, y=w2854) -> (x = y?=w2853:bool)
              n993 = Index Array(array=w2857, index=2) -> (element=w2856:i16)
              n994 = Compound Arithmetic op=OR(w2853, invert w2852) -> (w2851:bool)
              n995 = case shown="True" w2851 {
                tunnel: w2863 -> [_ w2873]
                tunnel: w2861 -> [w2865 w2872]
                tunnel: [w2865 w2871] -> w2860
                tunnel: w2859 -> [_ w2870]
                tunnel: w2857 -> [_ w2869]
                tunnel: w2856 -> [_ w2868]
                tunnel: [_ w2867] -> w2855
                tunnel: w2854 -> [_ w2866]
                frame False {
                }
                frame True {
                  n996 = case shown="1..8" w2866 {
                    tunnel: w2873 -> [_ w2878 w2893]
                    tunnel: w2872 -> [w2874 w2876 w2890]
                    tunnel: [w2874 w2877 w2889] -> w2871
                    tunnel: w2869 -> [_ w2879 w2892]
                    tunnel: w2870 -> [_ w2882 _]
                    tunnel: w2868 -> [_ w2881 w2891]
                    tunnel: [_ _ w2888] -> w2867
                    frame Default {
                      # "INCOMPATIBLE DATATYPES"
                    }
                    frame 112 {
                      # "Check if subtype matches"
                      # "REFNUM - CHECK SUBTYPE"
                      n997 = Index Array(array=w2882, index=2) -> (element=w2880:i16)
                      n998 = Equal?(x=w2881, y=w2880) -> (x = y?=w2875:bool)
                      n999 = case shown="True" w2875 {
                        tunnel: w2879 -> [_ w2887]
                        tunnel: w2878 -> [_ w2886]
                        tunnel: [w2884 w2885] -> w2877
                        tunnel: w2876 -> [w2884 _]
                        frame False {
                        }
                        frame True {
                          n1000 = Flattened String To Variant(6:w2886, 7:w2887) -> (3:w2885:variant)  [unwired: 1 in, 1 out]
                        }
                      }
                    }
                    frame 1..8 {
                      # "4-byte types or higher resolution"
                      n1001 = case shown="1, 4, 8, 9, 11, 12, 14, 15, 17, 19" w2891 {
                        tunnel: w2893 -> [_ w2904]
                        tunnel: w2892 -> [_ w2898]
                        tunnel: w2890 -> [w2894 _]
                        tunnel: [w2894 w2896] -> w2889
                        tunnel: [_ TRUE] -> w2888
                        frame Default {
                        }
                        frame 1, 4, 8, 9, 17, 18, 20, 21, 23, 25 {
                          # "Any types that have at least\n4 bytes."
                          n1002 = String To Byte Array(string=w2904) -> (unsigned byte array=w2903:u8[])
                          n1003 = Reverse 1D Array(array=w2903) -> (reversed array=w2902:u8[])
                          n1004 = Array Subset(array=w2902, length=4) -> (w2900:u8[])  [unwired: 1 in]
                          n1005 = Reverse 1D Array(array=w2900) -> (reversed array=w2899:u8[])
                          n1006 = Byte Array To String(unsigned byte array=w2899) -> (string=w2897:string)
                          n1007 = Flattened String To Variant(6:w2897, 7:w2898) -> (3:w2896:variant)  [unwired: 1 in, 1 out]
                        }
                      }
                    }
                  }
                }
              }
            }
          }
        }
      }
    }
  }
  "Value" <- w13
  "name out" <- w14
  "any found?" <- w7
  "all found?" <- w8
